vi "main.vi"() -> ()   [LabVIEW 2019]
uses:
  <vilib>/measure/mamon.llb/Trigger Detection for 1 Channel.vi
  <vilib>/addons/Fuzzy Logic/FL Fuzzy Controller (MISO).vi
  Setting Lib.lvlib
  detectedPellet.lvlib
  D02.lvlib
  D03.lvlib
  D04.lvlib
  D05.lvlib
  D01.lvlib
  database.lvlib
  <vilib>/measure/NI_MAPro.lvlib
  User Lib.lvlib
  <vilib>/addons/Fuzzy Logic/NI_Fuzzy_Logic_API.lvlib
  Maintenance.lvlib
  <vilib>/userDefined/High Color/IMAQdx.ctl
  <vilib>/Analysis/NI_AALPro.lvlib
  D06.lvlib
  <userlib>/DAQNavi Polymorphic VI/create/DAQNavi Create Channel(AI-Voltage).vi
  <userlib>/DAQNavi Polymorphic VI/create/DAQNavi Create Channel(DI-Digital Input).vi
  <userlib>/DAQNavi Polymorphic VI/read/DAQNavi Read (Digital 1D U8 NChan 1Samp).vi
  <userlib>/DAQNavi Polymorphic VI/read/DAQNavi Read (Analog 1D DBL NChan 1Samp).vi
  <userlib>/DAQNavi Polymorphic VI/create/DAQNavi Create Channel(DO-Digital Output).vi
  <userlib>/DAQNavi Polymorphic VI/write/DAQNavi Write (Digtial 1D U8 NChan 1Samp).vi
panel:
  out "Warning array 06":bool[](array[boolean])
  out "speed  min 06":bool
  out "speed max 06":bool
  out "10-14 6":dbl(slide) caption="10-14 mm" scale=0.0..100.0 scale format="%#.1f"
  out "8-16mm 6":dbl format="%.1g"
  out "AUTO/MAN 06":bool
  out "DISC 06":bool
  out "SPEED 07":dbl caption="SPEED" format="%#.2g"
  out "AVG 07":dbl caption="AVG" format="%#.2g"
  in  "Info 07":bool
  out "Warning 07":bool
  out "disc name 07":string="DISC 07"
  in  "Graph 07":bool
  in  "Live 07":bool
  out "AUTO/MAN 07":bool
  out "projector 07":bool
  out "cam 07":bool
  out "8-12.5 32":dbl(slide) caption="9-12.5 mm" scale=0.0..100.0 scale format="%#.1f"
  out "12.5-16 32":dbl(slide) caption="12.5-16 mm" scale=0.0..100.0 scale format="%#.1f"
  out "DISC 07":bool
  out "SPEED 06":dbl caption="SPEED" format="%#.2g"
  out "AVG 06":dbl caption="AVG" format="%#.2g"
  in  "Info 06":bool
  out "Warning 06":bool
  out "disc name 06":string="DISC 06"
  in  "Graph 06":bool
  in  "Live 06":bool
  out "projector 06":bool
  out "cam 06":bool
  out "8-12.5 06":dbl(slide) caption="9-12.5 mm" scale=0.0..100.0 scale format="%#.1f"
  out "12.5-16 06":dbl(slide) caption="12.5-16 mm" scale=0.0..100.0 scale format="%#.1f"
  out "rules as text out":string[](array[string])
  out "sudden change D05":bool
  out "pulse width D05":dbl
  out "slope D05":dbl
  out "previouse speed D05":dbl
  out "increase D05":bool
  out "decrease D05":bool
  out "sudden change D04":bool
  out "pulse width D04":dbl
  out "slope D04":dbl
  out "previouse speed D04":dbl
  out "increase D04":bool
  out "decrease D04":bool
  out "slope D03":dbl
  out "sudden change D03":bool
  out "pulse width D03":dbl
  out "previous speed D03":dbl
  out "increase D03":bool
  out "decrease D03":bool
  out "sudden change D02":bool
  out "pulse width D02":dbl
  out "slope D02":dbl
  out "previous speed D02":dbl
  out "increase D02":bool
  out "decrease D02":bool
  out "slope D01":dbl
  out "previous speed D01":dbl
  out "decrease D01":bool
  out "increase D01":bool
  out "last error 05":dbl
  out "no change D05":bool
  out "last error 04":dbl
  out "no change D04":bool
  out "last error 03":dbl
  out "no change D03":bool
  out "last error 02":dbl
  out "no change D02":bool
  out "sudden change D01":bool
  out "last error 01":dbl
  out "speed  min 05":bool
  out "speed max 05":bool
  out "speed  min 03":bool
  out "speed max 03":bool
  out "speed  min 04":bool
  out "speed max 04":bool
  out "speed  min 02":bool
  out "speed max 02":bool
  out "speed max 01":bool
  out "speed  min 01":bool
  out "no change D01":bool
  out "SPEED 05":dbl caption="SPEED" format="%#.2g"
  out "SPEED 04":dbl caption="SPEED" format="%#.2g"
  out "SPEED 03":dbl caption="SPEED" format="%#.2g"
  out "SPEED 02":dbl caption="SPEED" format="%#.2g"
  out "SPEED 01":dbl caption="SPEED" format="%#.2g"
  out "AVG 05":dbl caption="AVG" format="%#.2g"
  out "AVG 04":dbl caption="AVG" format="%#.2g"
  out "AVG 03":dbl caption="AVG" format="%#.2g"
  out "AVG 02":dbl caption="AVG" format="%#.2g"
  out "AVG 01":dbl caption="AVG" format="%#.2g"
  out "8-16mm total":dbl format="%.1g"
  out "8-16mm 05":dbl format="%.1g"
  out "8-16mm 04":dbl format="%.1g"
  out "8-16mm 03":dbl format="%.1g"
  out "8-16mm 27":dbl format="%.1g"
  out "8-16mm 26":dbl format="%.1g"
  out "10-14 total":dbl(slide) caption="10-14 mm" scale=0.0..100.0 scale format="%#.1f"
  out "10-14 05":dbl(slide) caption="10-14 mm" scale=0.0..100.0 scale format="%#.1f"
  out "10-14 04":dbl(slide) caption="10-14 mm" scale=0.0..100.0 scale format="%#.1f"
  out "10-14 03":dbl(slide) caption="10-14 mm" scale=0.0..100.0 scale format="%#.1f"
  out "10-14 02":dbl(slide) caption="10-14 mm" scale=0.0..100.0 scale format="%#.1f"
  out "10-14 01":dbl(slide) caption="10-14 mm" scale=0.0..100.0 scale format="%#.1f"
  out "error out 14":errorcluster
  out "error out 13":errorcluster
  out "error out 12":errorcluster
  in  "Info 05":bool
  in  "Info 04":bool
  in  "Info 03":bool
  in  "Info 02":bool
  in  "Info 01":bool
  out "error out":errorcluster
  out "avg grading array size":i32=4000
  out "live grading array size":i32=2000
  out "error out 8":errorcluster
  out "error out 7":errorcluster
  out "error out 6":errorcluster
  out "Elapsed Time (s) 6":dbl caption="Elapsed Time (s)"
  out "output value 5":dbl
  out "Elapsed Time (s) 5":dbl caption="Elapsed Time (s)"
  out "output value 4":dbl
  out "Elapsed Time (s) 4":dbl caption="Elapsed Time (s)"
  out "output value 3":dbl
  out "error out 5":errorcluster
  out "Elapsed Time (s) 3":dbl caption="Elapsed Time (s)"
  out "output value 2":dbl
  out "error out 3":errorcluster
  out "puls width D01":dbl
  out "Elapsed Time (s) 2":dbl caption="Elapsed Time (s)"
  out "2D array out":dbl[][](array[numeric])
  out "Warning array 01":bool[](array[boolean])
  out "Warning array 02":bool[](array[boolean])
  out "Warning array 03":bool[](array[boolean])
  out "Warning array 04":bool[](array[boolean])
  out "Warning array 05":bool[](array[boolean])
  out "Warning 05":bool
  in  "speed disc 30":i32
  in  "speed disc 29":i32
  in  "Error in 18":errorcluster
  in  "speed disc 28":i32
  in  "speed disc 27":i32
  in  "speed disc 26":i32
  out "Warning 04":bool
  out "Warning 03":bool
  out "Warning 02":bool
  out "Warning 01":bool
  out "overal result":string="Overal Result"
  out "disc name 05":string="DISC 05"
  out "disc name 04":string="DISC 04"
  out "disc name 03":string="DISC 03"
  out "disc name 02":string="DISC 02"
  in  "Setting":bool
  out "disc name 01":string="DISC 01"
  in  "Graph 05":bool
  in  "Live 05":bool
  in  "Graph 04":bool
  in  "Live 04":bool
  in  "Graph 03":bool
  in  "Live 03":bool
  in  "Graph 02":bool
  in  "Live 02":bool
  out "Software name":string="DORSA Smart Grading System (DSGS)"
  out "time&date":string="2020/11/22"
  in  "Maintenance":bool
  in  "Shutdown":bool
  in  "Restart":bool
  in  "Close":bool
  in  "View":bool
  in  "Report":bool
  in  "Login":bool=TRUE
  in  "Graph 01":bool
  in  "Live 01":bool
  out "8-12.5 02":dbl(slide) caption="9-12.5 mm" scale=0.0..100.0 scale format="%#.1f"
  out "12.5-16 02":dbl(slide) caption="12.5-16 mm" scale=0.0..100.0 scale format="%#.1f"
  out "AUTO/MAN 05":bool
  out "projector 05":bool
  out "cam 05":bool
  out "8-12.5 05":dbl(slide) caption="9-12.5 mm" scale=0.0..100.0 scale format="%#.1f"
  out "12.5-16 05":dbl(slide) caption="12.5-16 mm" scale=0.0..100.0 scale format="%#.1f"
  out "DISC 05":bool
  out "AUTO/MAN 04":bool
  out "projector 04":bool
  out "cam 04":bool
  out "8-12.5 04":dbl(slide) caption="9-12.5 mm" scale=0.0..100.0 scale format="%#.1f"
  out "12.5-16 04":dbl(slide) caption="12.5-16 mm" scale=0.0..100.0 scale format="%#.1f"
  out "DISC 04":bool
  out "AUTO/MAN 03":bool
  out "projector 03":bool
  out "cam 03":bool
  out "8-12.5 03":dbl(slide) caption="9-12.5 mm" scale=0.0..100.0 scale format="%#.1f"
  out "12.5-16 03":dbl(slide) caption="12.5-16 mm" scale=0.0..100.0 scale format="%#.1f"
  out "DISC 03":bool
  out "AUTO/MAN 02":bool
  out "projector 02":bool
  out "cam 02":bool
  out "DISC 02":bool
  out "AUTO/MAN 01":bool
  out "projector 01":bool
  out "cam 01":bool
  out "8-12.5 01":dbl(slide) caption="8-12.5 mm" scale=0.0..100.0 scale format="%#.1f"
  out "12.5-16 01":dbl(slide) caption="12.5-16 mm" scale=0.0..100.0 scale format="%#.1f"
  out "DISC 01":bool
  out "12.5-16 total":dbl(slide) caption="12.5-16 mm" scale=0.0..100.0 scale format="%#.1f"
  out "8-12.5 total":dbl(slide) caption="9-12.5mm" scale=0.0..100.0 scale format="%#.1f"
  out "Over Size":dbl format="%#.2g"
  out "AVG":dbl format="%#.2g"
  out "Under Size":dbl format="%#.2g"
types:
  T1 = cluster{"disc 06":bool, "auto/man 06":bool, "projector 06":bool, "cam 06":bool}
  T2 = cluster{"disc 05":bool, "auto/man 05":bool, "projector 05":bool, "cam 05":bool}
  T3 = cluster{"disc 04":bool, "auto/man 04":bool, "projector 04":bool, "cam 04":bool}
  T4 = cluster{"disc 03":bool, "auto/man 03":bool, "projector 03":bool, "cam 03":bool}
  T5 = cluster{"disc 02":bool, "auto/man 02":bool, "projector 02":bool, "cam 02":bool}
  T6 = cluster{"disc 01":bool, "auto/man 01":bool, "projector 01":bool, "cam 01":bool}
  T7 = typedef "IMAQ Image.ctl" = refnum<image>
  T8 = enum32{"Invalid", "Standard", "Closed", "Hidden", "Minimized", "Maximized"}
  T9 = typedef "IMAQdx.ctl" = refnum<k21>
  T10 = enum8{"Enabled", "Disabled", "Disabled and Grayed Out"}
  T11 = cluster{string, "date/time string":string, "date/time string":string, string}
  T12 = cluster{i32, "date/time string":string, "date/time string":string, string}
  T13 = cluster{"disc 01":bool, "auto/man 01":bool, "projector 01":bool, "cam 01":bool}[]
  T14 = cluster{"disc 02":bool, "auto/man 02":bool, "projector 02":bool, "cam 02":bool}[]
  T15 = cluster{"disc 06":bool, "auto/man 06":bool, "projector 06":bool, "cam 06":bool}[]
  T16 = cluster{"disc 05":bool, "auto/man 05":bool, "projector 05":bool, "cam 05":bool}[]
  T17 = cluster{"disc 03":bool, "auto/man 03":bool, "projector 03":bool, "cam 03":bool}[]
  T18 = cluster{"disc 04":bool, "auto/man 04":bool, "projector 04":bool, "cam 04":bool}[]
  T19 = typedef "LVDateTimeRec.ctl" = cluster{"fractional second":dbl, "second":i32, "minute":i32, "hour":i32, "day of month":i32, "month":i32, "year":i32, "day of week":i32, "day of year":i32, "DST":i32}
  T20 = cluster{"date/time string":string, "date/time string":string, dbl, dbl, dbl, dbl, dbl, dbl, dbl, dbl, "f":string, "f":string, "time format string (%c)":string, "time format string (%c)":string}
  T21 = cluster{"date/time string":string, "date/time string":string, dbl, dbl, "f":string, "f":string, "time format string (%c)":string, "time format string (%c)":string}
  T22 = cluster{"date/time string":string, "date/time string":string, string, "spreadsheet string":string}
  T23 = typedef "NI_Fuzzy_Logic_API.lvlib/FL System.ctl" = cluster{"input variables":T24[], "output variables":T24[], "rules":T27[], "defuzzification method":T33, "description":string, "user MF interpolating polynomials":T34[]}
  T24 = typedef "NI_Fuzzy_Logic_API.lvlib/FL Variable.ctl" = cluster{"name":string, "range":dbl[], "MFs":T25[]}
  T25 = typedef "NI_Fuzzy_Logic_API.lvlib/FL Membership Function.ctl" = cluster{"name":string, "shape":T26, "points":dbl[], "color":u32, "user-defined shape index":i32}
  T26 = typedef "NI_Fuzzy_Logic_API.lvlib/FL Membership Function Shape.ctl" = u16
  T27 = typedef "NI_Fuzzy_Logic_API.lvlib/FL Rule.ctl" = cluster{"antecedents":T28[], "antecedent connective":T30, "consequents":T31[], "consequent implication":T32, "degree of support":dbl}
  T28 = typedef "NI_Fuzzy_Logic_API.lvlib/FL Antecedent.ctl" = cluster{"Var Index":i32, "MF Index":i32, "Cond":T29}
  T29 = typedef "NI_Fuzzy_Logic_API.lvlib/FL Modifier.ctl" = u16
  T30 = typedef "NI_Fuzzy_Logic_API.lvlib/FL Antecedent Connective.ctl" = u16
  T31 = typedef "NI_Fuzzy_Logic_API.lvlib/FL Consequent.ctl" = cluster{"Var Index":i32, "MF Index":i32, "Cond":T29}
  T32 = typedef "NI_Fuzzy_Logic_API.lvlib/FL Consequent Implication.ctl" = u16
  T33 = typedef "NI_Fuzzy_Logic_API.lvlib/FL Defuzzification.ctl" = u16
  T34 = typedef "NI_Fuzzy_Logic_API.lvlib/FL Interpolating polynomials.ctl" = cluster{"X":dbl[], "Y":dbl[], "Y(x) coeff":dbl[][], "X(y) coeff":dbl[][], "Area(y) coeff":dbl[][], "coa_x(y) coeff":dbl[][]}
  T35 = cluster{"decrease D01":bool, "increase D01":bool, "no change D01":bool, "sudden change D01":bool, "last error 01":dbl, "previous speed D01":dbl, "puls width D01":dbl, "slope D01":dbl}
  T36 = cluster{"decrease D05":bool, "increase D05":bool, "no change D05":bool, "sudden change D05":bool, "last error 05":dbl, "previouse speed D05":dbl, "pulse width D05":dbl, "slope D05":dbl}
  T37 = cluster{"decrease D02":bool, "increase D02":bool, "no change D02":bool, "sudden change D02":bool, "last error 02":dbl, "previous speed D02":dbl, "pulse width D02":dbl, "slope D02":dbl}
  T38 = cluster{"decrease D04":bool, "increase D04":bool, "no change D04":bool, "sudden change D04":bool, "last error 04":dbl, "previouse speed D04":dbl, "pulse width D04":dbl, "slope D04":dbl}
  T39 = cluster{"decrease D03":bool, "increase D03":bool, "no change D03":bool, "sudden change D03":bool, "last error 03":dbl, "previous speed D03":dbl, "pulse width D03":dbl, "slope D03":dbl}
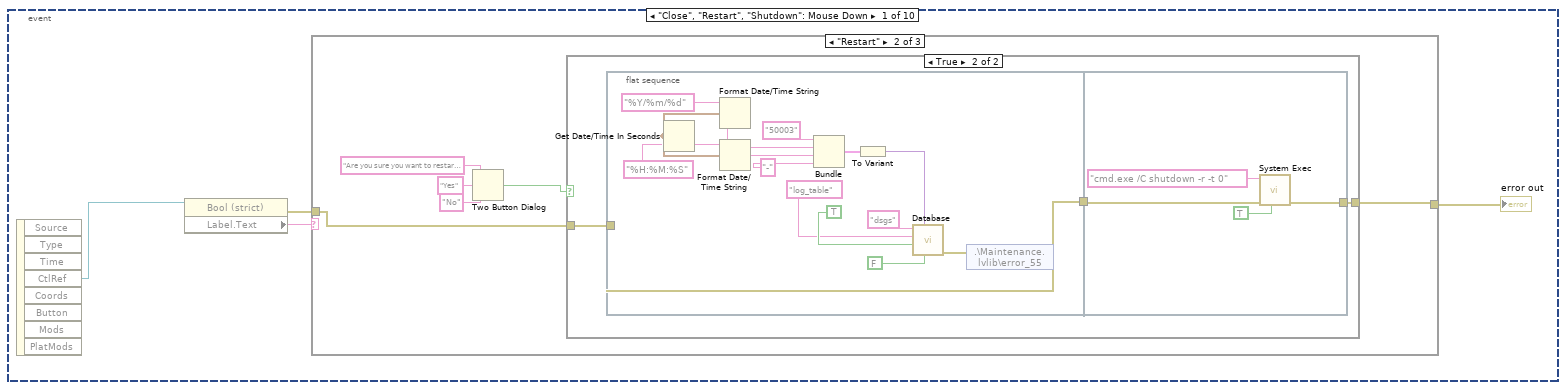
[diagram p3: hidden frame]
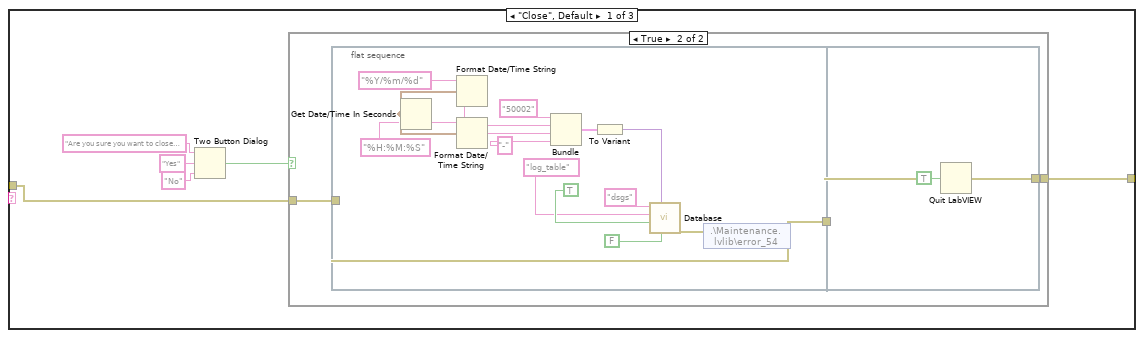
[diagram p4: hidden frame]
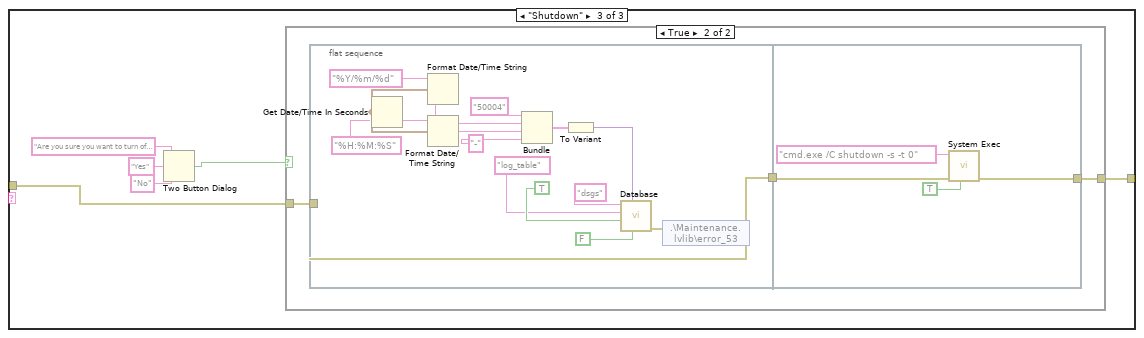
[diagram p7: hidden frame]
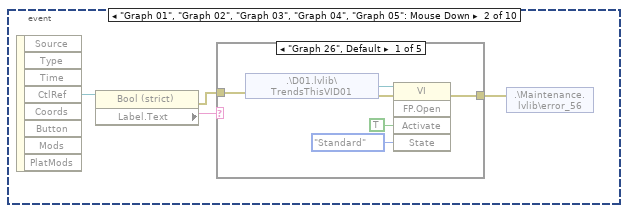
[diagram p9: hidden frame]
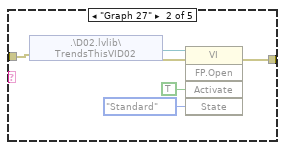
[diagram p10: hidden frame]
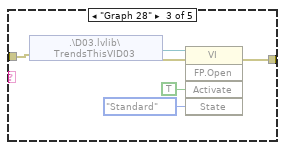
[diagram p11: hidden frame]
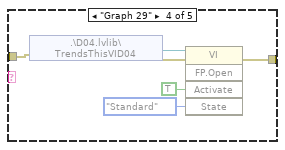
[diagram p12: hidden frame]
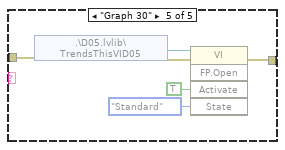
[diagram p13: hidden frame]
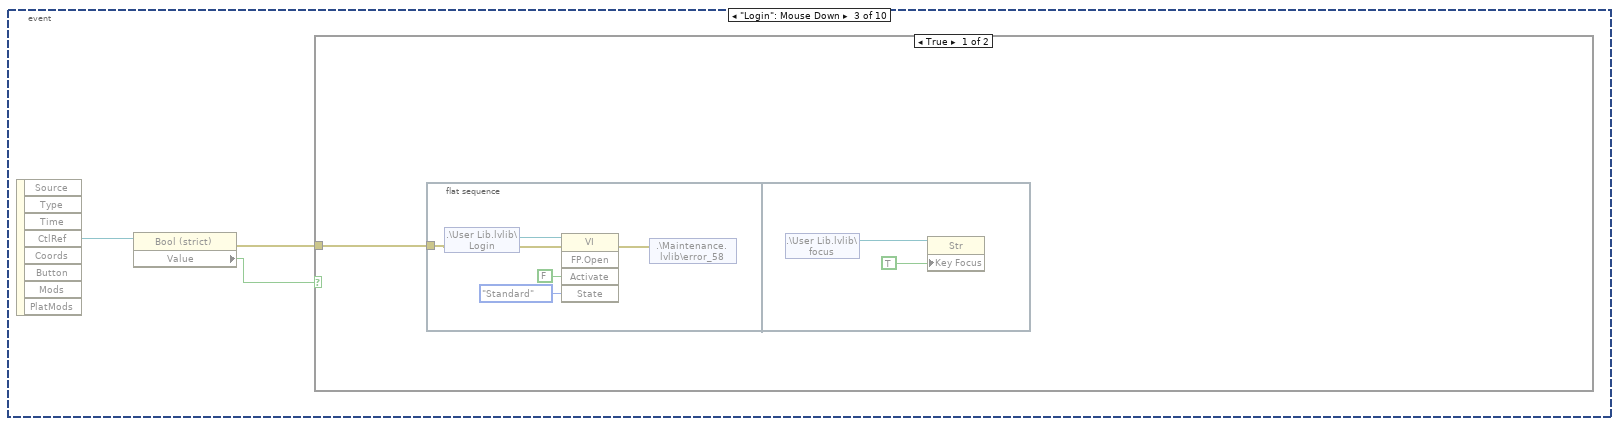
[diagram p14: hidden frame]
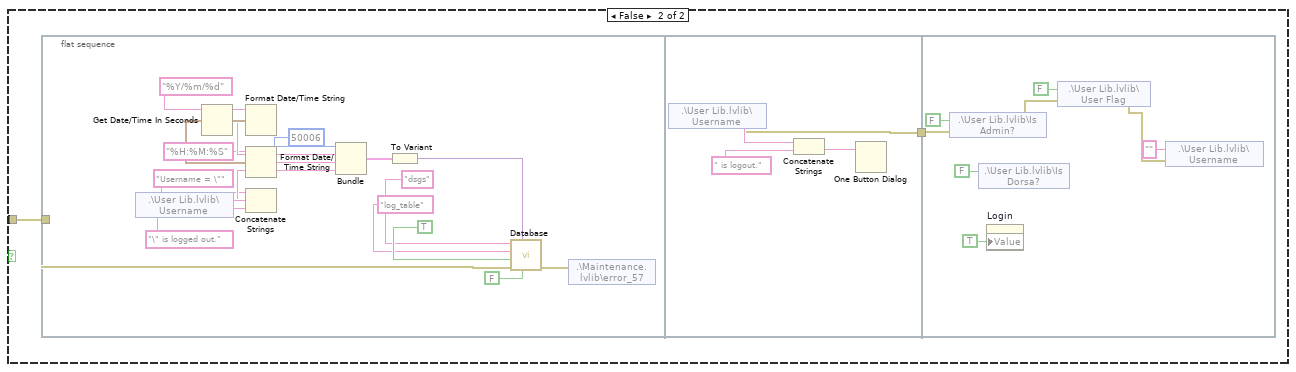
[diagram p15: hidden frame]
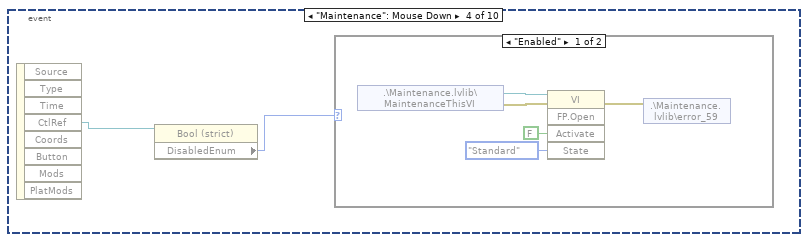
[diagram p16: hidden frame]
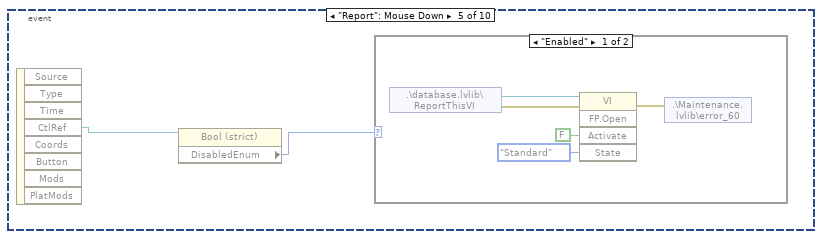
[diagram p18: hidden frame]
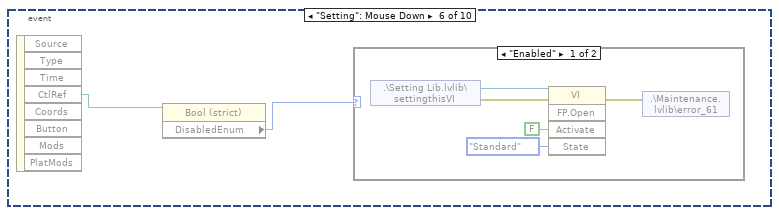
[diagram p20: hidden frame]
diagram:
  w80 = 4000 ("dimension size")
  w85 = 1000 ("dimension size")
  n1 = call "IMAQ Create"("Image Name"="img in D01") -> ("New Image"=w53:T7, "error out"=w44:errorcluster)  [unwired: 4 in]
  n2 = shared-variable ".\\Maintenance.lvlib\\error_2"(w44) -> ()  [unwired: 1 in, 1 out]
  n3 = call "IMAQ Create"("Image Name"="img in D02") -> ("New Image"=w27:T7, "error out"=w43:errorcluster)  [unwired: 4 in]
  n4 = shared-variable ".\\Maintenance.lvlib\\error_3"(w43) -> ()  [unwired: 1 in, 1 out]
  n5 = call "IMAQ Create"("Image Name"="img in D03") -> ("New Image"=w48:T7, "error out"=w42:errorcluster)  [unwired: 4 in]
  n6 = shared-variable ".\\Maintenance.lvlib\\error_4"(w42) -> ()  [unwired: 1 in, 1 out]
  n7 = call "IMAQ Create"("Image Name"="img in D04") -> ("New Image"=w47:T7, "error out"=w41:errorcluster)  [unwired: 4 in]
  n8 = shared-variable ".\\Maintenance.lvlib\\error_5"(w41) -> ()  [unwired: 1 in, 1 out]
  n9 = call "IMAQ Create"("Image Name"="img in D05") -> ("New Image"=w46:T7, "error out"=w40:errorcluster)  [unwired: 4 in]
  n10 = call "IMAQ Create"("Image Name"="img out D01") -> ("New Image"=w96:T7, "error out"=w39:errorcluster)  [unwired: 4 in]
  n11 = shared-variable ".\\Maintenance.lvlib\\error_6"(w40) -> ()  [unwired: 1 in, 1 out]
  n12 = shared-variable ".\\Maintenance.lvlib\\error_7"(w39) -> ()  [unwired: 1 in, 1 out]
  n13 = call "IMAQ Create"("Image Name"="img out D02") -> ("New Image"=w94:T7, "error out"=w38:errorcluster)  [unwired: 4 in]
  n14 = call "IMAQ Create"("Image Name"="img in D06") -> ("New Image"=w6:T7)  [unwired: 4 in, 1 out]
  n15 = shared-variable ".\\Maintenance.lvlib\\error_8"(w38) -> ()  [unwired: 1 in, 1 out]
  n16 = call "IMAQ Create"("Image Name"="img out D03") -> ("New Image"=w92:T7, "error out"=w37:errorcluster)  [unwired: 4 in]
  n17 = shared-variable ".\\Maintenance.lvlib\\error_9"(w37) -> ()  [unwired: 1 in, 1 out]
  n18 = call "IMAQ Create"("Image Name"="img out D04") -> ("New Image"=w89:T7, "error out"=w36:errorcluster)  [unwired: 4 in]
  n19 = shared-variable ".\\Maintenance.lvlib\\error_10"(w36) -> ()  [unwired: 1 in, 1 out]
  n20 = disable-structure shown="Disabled" {
    frame Disabled {
      n21 = call-poly <userlib>:"DAQNavi Create Channel.vi"("physical channels"="PCI-1710,BID#0/ai0:9", "signal type"="Differential", "value range"="0 ~ 10 V") -> ("task out"=w112:i32, "error out"=w111:errorcluster)  [unwired: 11 in]
      n22 = call-poly <userlib>:"DAQNavi Create Channel.vi"("physical channels"="PCI-1710,BID#0/port0:1") -> ("task out"=w110:i32, "error out"=w109:errorcluster)  [unwired: 13 in]
      n23 = while {
        tunnel: w112 -> [w123]
        tunnel: w111 -> [w122]
        tunnel: w110 -> [w121]
        tunnel: w109 -> [w120]
        stop <- FALSE stop-if-true
        n24 = event shown="[9] Timeout" {
          selector: _ -> [_ _ _ _ _ _ _ _ _ _]
          dyn-events: _ -> [_ _ _ _ _ _ _ _ _ _]
          timeout: 0 -> [_ _ _ _ _ _ _ _ _ _]
          tunnel: w123 -> [_ _ _ _ _ _ _ _ _ w610]
          tunnel: w122 -> [_ _ _ _ _ _ _ _ _ w609]
          tunnel: w121 -> [_ _ _ _ _ _ _ _ _ w595]
          tunnel: w120 -> [_ _ _ _ _ _ _ _ _ w594]
          event "Close", "Restart", "Shutdown": Mouse Down {
            n25 = event-data() -> ("CtlRef"=w129:refnum<vi>)  [unwired: 1 in, 7 out]
            n26 = property class="Bool (strict)"(reference=w129) -> (error out=w128:errorcluster, "Label.Text"=w130:string)  [unwired: 1 in, 1 out]
            n27 = case shown="\"Restart\"" w130 {
              tunnel: [w131 w158 w188] -> w127
              tunnel: w128 -> [w132 w159 w187]
              frame "Close", Default {
                n28 = Two Button Dialog(message="Are you sure you want to close the application?", 1:"No" ("F button name (\"Cancel\")"), 2:"Yes" ("T button name (\"OK\")")) -> (T button?=w133:bool)
                n29 = case shown="True" w133 {
                  tunnel: w132 -> [w137 w138]
                  tunnel: [w137 w140] -> w131
                  frame False {
                  }
                  frame True {
                    n30 = flat-sequence {
                      tunnel: [w141] -> w139
                      tunnel: w138 -> [w141]
                      tunnel: [w156] -> w140
                      tunnel: w139 -> [w156]
                      frame #0 {
                        n31 = Get Date/Time In Seconds() -> (seconds since 1Jan1904=w151:timestamp)
                        n32 = Format Date/Time String(time format string (%c)="%Y/%m/%d", seconds (now)=w151) -> (date/time string=w152:string)  [unwired: 1 in]
                        n33 = Format Date/Time String(time format string (%c)="%H:%M:%S", seconds (now)=w151) -> (date/time string=w153:string)  [unwired: 1 in]
                        n34 = Bundle("50002", "date/time string"=w152, "date/time string"=w153, "-") -> (w154:T11)  [unwired: 1 in]
                        n35 = To Variant(anything=w154) -> (Variant=w155:variant)
                        n36 = call "Database.vi"("Delete row?"=FALSE, "Data"=w155, "Auto Increment ID?"=TRUE, "Table"="log_table", "Connection"="dsgs") -> ("Error out"=w142:errorcluster)  [unwired: 6 in]
                        n37 = shared-variable ".\\Maintenance.lvlib\\error_54"(w142) -> ()  [unwired: 1 in, 1 out]
                      }
                      frame #1 {
                        n38 = Quit LabVIEW(quit? (T)=TRUE) -> ()
                      }
                    }
                  }
                }
              }
              frame "Restart" {
                n39 = Two Button Dialog(message="Are you sure you want to restart the system?", 1:"No" ("F button name (\"Cancel\")"), 2:"Yes" ("T button name (\"OK\")")) -> (T button?=w160:bool)
                n40 = case shown="True" w160 {
                  tunnel: w159 -> [w164 w167]
                  tunnel: [w164 w165] -> w158
                  frame False {
                  }
                  frame True {
                    n41 = flat-sequence {
                      tunnel: w167 -> [w169]
                      tunnel: [w169] -> w166
                      tunnel: w166 -> [w184]
                      tunnel: [w183] -> w165
                      frame #0 {
                        n42 = Get Date/Time In Seconds() -> (seconds since 1Jan1904=w178:timestamp)
                        n43 = Format Date/Time String(time format string (%c)="%Y/%m/%d", seconds (now)=w178) -> (date/time string=w179:string)  [unwired: 1 in]
                        n44 = Format Date/Time String(time format string (%c)="%H:%M:%S", seconds (now)=w178) -> (date/time string=w180:string)  [unwired: 1 in]
                        n45 = Bundle("50003", "date/time string"=w179, "date/time string"=w180, "-") -> (w181:T11)  [unwired: 1 in]
                        n46 = To Variant(anything=w181) -> (Variant=w182:variant)
                        n47 = call "Database.vi"("Delete row?"=FALSE, "Data"=w182, "Auto Increment ID?"=TRUE, "Table"="log_table", "Connection"="dsgs") -> ("Error out"=w168:errorcluster)  [unwired: 6 in]
                        n48 = shared-variable ".\\Maintenance.lvlib\\error_55"(w168) -> ()  [unwired: 1 in, 1 out]
                      }
                      frame #1 {
                        n49 = call <vilib>:"System Exec.vi"("run minimized? (F)"=TRUE, "error in (no error)"=w184, "command line"="cmd.exe /C shutdown -r -t 0") -> ("error out"=w183:errorcluster)  [unwired: 5 in, 3 out]
                      }
                    }
                  }
                }
              }
              frame "Shutdown" {
                n50 = Two Button Dialog(message="Are you sure you want to turn off the system?", 1:"No" ("F button name (\"Cancel\")"), 2:"Yes" ("T button name (\"OK\")")) -> (T button?=w189:bool)
                n51 = case shown="True" w189 {
                  tunnel: [w193 w196] -> w188
                  tunnel: w187 -> [w193 w195]
                  frame False {
                  }
                  frame True {
                    n52 = flat-sequence {
                      tunnel: w195 -> [w197]
                      tunnel: [w197] -> w194
                      tunnel: [w213] -> w196
                      tunnel: w194 -> [w212]
                      frame #0 {
                        n53 = Get Date/Time In Seconds() -> (seconds since 1Jan1904=w207:timestamp)
                        n54 = Format Date/Time String(time format string (%c)="%Y/%m/%d", seconds (now)=w207) -> (date/time string=w208:string)  [unwired: 1 in]
                        n55 = Format Date/Time String(time format string (%c)="%H:%M:%S", seconds (now)=w207) -> (date/time string=w209:string)  [unwired: 1 in]
                        n56 = Bundle("50004", "date/time string"=w208, "date/time string"=w209, "-") -> (w210:T11)  [unwired: 1 in]
                        n57 = To Variant(anything=w210) -> (Variant=w211:variant)
                        n58 = call "Database.vi"("Delete row?"=FALSE, "Data"=w211, "Auto Increment ID?"=TRUE, "Table"="log_table", "Connection"="dsgs") -> ("Error out"=w198:errorcluster)  [unwired: 6 in]
                        n59 = shared-variable ".\\Maintenance.lvlib\\error_53"(w198) -> ()  [unwired: 1 in, 1 out]
                      }
                      frame #1 {
                        n60 = call <vilib>:"System Exec.vi"("run minimized? (F)"=TRUE, "error in (no error)"=w212, "command line"="cmd.exe /C shutdown -s -t 0") -> ("error out"=w213:errorcluster)  [unwired: 5 in, 3 out]
                      }
                    }
                  }
                }
              }
            }
            "error out" <- w127
          }
          event "Graph 01", "Graph 02", "Graph 03", "Graph 04", "Graph 05": Mouse Down {
            n61 = event-data() -> ("CtlRef"=w217:refnum<vi>)  [unwired: 1 in, 7 out]
            n62 = property class="Bool (strict)"(reference=w217) -> (error out=w218:errorcluster, "Label.Text"=w219:string)  [unwired: 1 in, 1 out]
            n63 = case shown="\"Graph 26\", Default" w219 {
              tunnel: w218 -> [w222 w227 w233 w239 w245]
              tunnel: [w220 w226 w232 w238 w244] -> w216
              frame "Graph 26", Default {
                n64 = shared-variable ".\\D01.lvlib\\TrendsThisVID01"(error in=w222) -> (w225:refnum<vi>, error out=w221:errorcluster)
                n65 = invoke class="VI" method="FP.Open"(reference=w225, error in=w221, "Activate"=TRUE ("Activate?"), "State"=T8."Standard") -> (error out=w220:errorcluster)  [unwired: 1 in, 4 out]
              }
              frame "Graph 27" {
                n66 = shared-variable ".\\D02.lvlib\\TrendsThisVID02"(error in=w227) -> (w230:refnum<vi>, error out=w231:errorcluster)
                n67 = invoke class="VI" method="FP.Open"(reference=w230, error in=w231, "Activate"=TRUE ("Activate?"), "State"=T8."Standard") -> (error out=w226:errorcluster)  [unwired: 1 in, 4 out]
              }
              frame "Graph 28" {
                n68 = shared-variable ".\\D03.lvlib\\TrendsThisVID03"(error in=w233) -> (w236:refnum<vi>, error out=w237:errorcluster)
                n69 = invoke class="VI" method="FP.Open"(reference=w236, error in=w237, "Activate"=TRUE ("Activate?"), "State"=T8."Standard") -> (error out=w232:errorcluster)  [unwired: 1 in, 4 out]
              }
              frame "Graph 29" {
                n70 = shared-variable ".\\D04.lvlib\\TrendsThisVID04"(error in=w239) -> (w242:refnum<vi>, error out=w243:errorcluster)
                n71 = invoke class="VI" method="FP.Open"(reference=w242, error in=w243, "Activate"=TRUE ("Activate?"), "State"=T8."Standard") -> (error out=w238:errorcluster)  [unwired: 1 in, 4 out]
              }
              frame "Graph 30" {
                n72 = shared-variable ".\\D05.lvlib\\TrendsThisVID05"(error in=w245) -> (w248:refnum<vi>, error out=w249:errorcluster)
                n73 = invoke class="VI" method="FP.Open"(reference=w248, error in=w249, "Activate"=TRUE ("Activate?"), "State"=T8."Standard") -> (error out=w244:errorcluster)  [unwired: 1 in, 4 out]
              }
            }
            n74 = shared-variable ".\\Maintenance.lvlib\\error_56"(w216) -> ()  [unwired: 1 in, 1 out]
          }
          event "Login": Mouse Down {
            n75 = event-data() -> ("CtlRef"=w252:refnum<vi>)  [unwired: 1 in, 7 out]
            n76 = property class="Bool (strict)"(reference=w252) -> (error out=w250:errorcluster, "Value"=w251:bool)  [unwired: 1 in, 1 out]
            n77 = case shown="True" w251 {
              tunnel: w250 -> [w253 w262]
              frame True {
                n78 = flat-sequence {
                  tunnel: w253 -> [w258]
                  frame #0 {
                    n79 = shared-variable ".\\User Lib.lvlib\\Login"() -> (w257:refnum<vi>)  [unwired: 1 in, 1 out]
                    n80 = invoke class="VI" method="FP.Open"(reference=w257, error in=w258, "Activate"=FALSE ("Activate?"), "State"=T8."Standard") -> (error out=w254:errorcluster)  [unwired: 1 in, 4 out]
                    n81 = shared-variable ".\\Maintenance.lvlib\\error_58"(w254) -> ()  [unwired: 1 in, 1 out]
                  }
                  frame #1 {
                    n82 = shared-variable ".\\User Lib.lvlib\\focus"() -> (w260:refnum<vi>)  [unwired: 1 in, 1 out]
                    n83 = property class="Str"(reference=w260, "Key Focus"=TRUE) -> ()  [unwired: 1 in, 2 out]
                  }
                }
              }
              frame False {
                n84 = flat-sequence {
                  tunnel: w262 -> [w264]
                  tunnel: [w281] -> w261
                  tunnel: w261 -> [w288]
                  frame #0 {
                    n85 = shared-variable ".\\User Lib.lvlib\\Username"() -> (w280:string)  [unwired: 1 in, 1 out]
                    n86 = Get Date/Time In Seconds() -> (seconds since 1Jan1904=w278:timestamp)
                    n87 = Format Date/Time String(time format string (%c)="%Y/%m/%d", seconds (now)=w278) -> (date/time string=w277:string)  [unwired: 1 in]
                    n88 = Format Date/Time String(time format string (%c)="%H:%M:%S", seconds (now)=w278) -> (date/time string=w276:string)  [unwired: 1 in]
                    n89 = Concatenate Strings("Username = \"" ("string"), w280, "\" is logged out." ("string")) -> (w279:string)
                    n90 = Bundle(50006, "date/time string"=w277, "date/time string"=w276, w279) -> (w275:T12)  [unwired: 1 in]
                    n91 = To Variant(anything=w275) -> (Variant=w274:variant)
                    n92 = call "Database.vi"("Delete row?"=FALSE, "Data"=w274, "Error in"=w264, "Auto Increment ID?"=TRUE, "Table"="log_table" ("table"), "Connection"="dsgs" ("table")) -> ("Error out"=w263:errorcluster)  [unwired: 5 in]
                    n93 = shared-variable ".\\Maintenance.lvlib\\error_57"(w263) -> ()  [unwired: 1 in, 1 out]
                  }
                  frame #1 {
                    n94 = shared-variable ".\\User Lib.lvlib\\Username"() -> (w283:string, error out=w281:errorcluster)  [unwired: 1 in]
                    n95 = Concatenate Strings(w283, " is logout." ("string")) -> (w284:string)
                    n96 = One Button Dialog(message=w284) -> ()  [unwired: 1 in, 1 out]
                  }
                  frame #2 {
                    n97 = shared-variable ".\\User Lib.lvlib\\Is Admin?"(FALSE ("Is Admin?"), error in=w288) -> (error out=w287:errorcluster)
                    n98 = shared-variable ".\\User Lib.lvlib\\Is Dorsa?"(FALSE ("Is Admin?")) -> ()  [unwired: 1 in, 1 out]
                    n99 = property on="Login" class="Bool (strict)"("Value"=TRUE ("Login")) -> ()  [unwired: 2 in, 2 out]
                    n100 = shared-variable ".\\User Lib.lvlib\\User Flag"(FALSE ("User Flag"), error in=w287) -> (error out=w286:errorcluster)
                    n101 = shared-variable ".\\User Lib.lvlib\\Username"("" ("Username"), error in=w286) -> ()  [unwired: 1 out]
                  }
                }
              }
            }
          }
          event "Maintenance": Mouse Down {
            n102 = event-data() -> ("CtlRef"=w294:refnum<vi>)  [unwired: 1 in, 7 out]
            n103 = property class="Bool (strict)"(reference=w294) -> ("DisabledEnum"=w293:T10)  [unwired: 1 in, 2 out]
            n104 = case shown="\"Enabled\"" w293 {
              frame "Enabled" {
                n105 = shared-variable ".\\Maintenance.lvlib\\MaintenanceThisVI"() -> (w299:refnum<vi>, error out=w298:errorcluster)  [unwired: 1 in]
                n106 = invoke class="VI" method="FP.Open"(reference=w299, error in=w298, "Activate"=FALSE ("Activate?"), "State"=T8."Standard") -> (error out=w297:errorcluster)  [unwired: 1 in, 4 out]
                n107 = shared-variable ".\\Maintenance.lvlib\\error_59"(w297) -> ()  [unwired: 1 in, 1 out]
              }
              frame "Disabled", Default {
              }
            }
          }
          event "Report": Mouse Down {
            n108 = event-data() -> ("CtlRef"=w301:refnum<vi>)  [unwired: 1 in, 7 out]
            n109 = property class="Bool (strict)"(reference=w301) -> ("DisabledEnum"=w300:T10)  [unwired: 1 in, 2 out]
            n110 = case shown="\"Enabled\"" w300 {
              frame "Enabled" {
                n111 = shared-variable ".\\database.lvlib\\ReportThisVI"() -> (w304:refnum<vi>, error out=w306:errorcluster)  [unwired: 1 in]
                n112 = invoke class="VI" method="FP.Open"(reference=w304, error in=w306, "Activate"=FALSE ("Activate?"), "State"=T8."Standard") -> (error out=w305:errorcluster)  [unwired: 1 in, 4 out]
                n113 = shared-variable ".\\Maintenance.lvlib\\error_60"(w305) -> ()  [unwired: 1 in, 1 out]
              }
              frame "Disabled", Default {
              }
            }
          }
          event "Setting": Mouse Down {
            n114 = event-data() -> ("CtlRef"=w308:refnum<vi>)  [unwired: 1 in, 7 out]
            n115 = property class="Bool (strict)"(reference=w308) -> ("DisabledEnum"=w307:T10)  [unwired: 1 in, 2 out]
            n116 = case shown="\"Enabled\"" w307 {
              frame "Enabled" {
                n117 = shared-variable ".\\Setting Lib.lvlib\\settingthisVI"() -> (w312:refnum<vi>, error out=w311:errorcluster)  [unwired: 1 in]
                n118 = invoke class="VI" method="FP.Open"(reference=w312, error in=w311, "Activate"=FALSE ("Activate?"), "State"=T8."Standard") -> (error out=w313:errorcluster)  [unwired: 1 in, 4 out]
                n119 = shared-variable ".\\Maintenance.lvlib\\error_61"(w313) -> ()  [unwired: 1 in, 1 out]
              }
              frame "Disabled", Default {
              }
            }
          }
          event "View", "Live 01", "Live 02", "Live 03", "Live 04", "Live 05": Mouse Down {
            n120 = event-data() -> ("CtlRef"=w315:refnum<vi>)  [unwired: 1 in, 7 out]
            n121 = property class="Bool (strict)"(reference=w315) -> (error out=w316:errorcluster, "Label.Text"=w317:string)  [unwired: 1 in, 1 out]
            n122 = case shown="\"View\"" w317 {
              tunnel: w316 -> [w320 w329 w331 w337 w343 w350]
              tunnel: [w318 w324 w330 w336 w342 w351] -> w314
              frame "Live 26", Default {
                n123 = shared-variable ".\\D01.lvlib\\D01thisVI"(error in=w320) -> (w323:refnum<vi>, error out=w319:errorcluster)
                n124 = invoke class="VI" method="FP.Open"(reference=w323, error in=w319, "Activate"=FALSE ("Activate?"), "State"=T8."Standard") -> (error out=w318:errorcluster)  [unwired: 1 in, 4 out]
              }
              frame "Live 27" {
                n125 = shared-variable ".\\D02.lvlib\\D02thisVI"(error in=w329) -> (w328:refnum<vi>, error out=w327:errorcluster)
                n126 = invoke class="VI" method="FP.Open"(reference=w328, error in=w327, "Activate"=TRUE ("Activate?"), "State"=T8."Standard") -> (error out=w324:errorcluster)  [unwired: 1 in, 4 out]
              }
              frame "Live 28" {
                n127 = shared-variable ".\\D03.lvlib\\D03thisVI"(error in=w331) -> (w333:refnum<vi>, error out=w332:errorcluster)
                n128 = invoke class="VI" method="FP.Open"(reference=w333, error in=w332, "Activate"=TRUE ("Activate?"), "State"=T8."Standard") -> (error out=w330:errorcluster)  [unwired: 1 in, 4 out]
              }
              frame "Live 29" {
                n129 = shared-variable ".\\D04.lvlib\\D04thisVI"(error in=w337) -> (w339:refnum<vi>, error out=w338:errorcluster)
                n130 = invoke class="VI" method="FP.Open"(reference=w339, error in=w338, "Activate"=TRUE ("Activate?"), "State"=T8."Standard") -> (error out=w336:errorcluster)  [unwired: 1 in, 4 out]
              }
              frame "Live 30" {
                n131 = shared-variable ".\\D05.lvlib\\D05thisVI"(error in=w343) -> (w347:refnum<vi>, error out=w346:errorcluster)
                n132 = invoke class="VI" method="FP.Open"(reference=w347, error in=w346, "Activate"=TRUE ("Activate?"), "State"=T8."Standard") -> (error out=w342:errorcluster)  [unwired: 1 in, 4 out]
              }
              frame "View" {
                n133 = shared-variable ".\\detectedPellet.lvlib\\open flag"(TRUE ("open flag"), error in=w350) -> (error out=w349:errorcluster)
                n134 = shared-variable ".\\detectedPellet.lvlib\\DetectedPelletThisVi"(error in=w349) -> (w352:refnum<vi>, error out=w353:errorcluster)
                n135 = invoke class="VI" method="FP.Open"(reference=w352, error in=w353, "Activate"=TRUE ("Activate?"), "State"=T8."Standard") -> (error out=w351:errorcluster)  [unwired: 1 in, 4 out]
              }
            }
            n136 = shared-variable ".\\Maintenance.lvlib\\error_62"(w314) -> ()  [unwired: 1 in, 1 out]
          }
          event "Info 01", "Info 02", "Info 03", "Info 04", "Info 05": Mouse Down {
            n137 = event-data() -> ("CtlRef"=w357:refnum<vi>)  [unwired: 1 in, 7 out]
            n138 = property class="Bool (strict)"(reference=w357) -> ("Label.Text"=w356:string)  [unwired: 1 in, 2 out]
            n139 = case shown="\"Info 26\", Default" w356 {
              frame "Info 26", Default {
                n140 = call "camera info.vi"("Disc Number"="Disc 26", "Camera Name"=T9 "disc26" ("Session In")) -> ()  [unwired: 10 in]
              }
              frame "Info 27" {
                n141 = call "camera info.vi"("Disc Number"="Disc 27", "Camera Name"=T9 "disc27" ("Session In")) -> ()  [unwired: 10 in]
              }
              frame "Info 28" {
                n142 = call "camera info.vi"("Disc Number"="Disc 28", "Camera Name"=T9 "disc28" ("Session In")) -> ()  [unwired: 10 in]
              }
              frame "Info 29" {
                n143 = call "camera info.vi"("Disc Number"="Disc 29", "Camera Name"=T9 "disc29" ("Session In")) -> ()  [unwired: 10 in]
              }
              frame "Info 30" {
                n144 = call "camera info.vi"("Disc Number"="Disc 30", "Camera Name"=T9 "disc30" ("Session In")) -> ()  [unwired: 10 in]
              }
            }
          }
          event "Warning 01", "Warning 02", "Warning 03", "Warning 04", "Warning 05": Mouse Down {
            n145 = event-data() -> ("CtlRef"=w370:refnum<vi>)  [unwired: 1 in, 7 out]
            n146 = property class="Bool (strict)"(reference=w370) -> (error out=w368:errorcluster, "Label.Text"=w369:string)  [unwired: 1 in, 1 out]
            n147 = case shown="\"Warning 26\", Default" w369 {
              tunnel: w368 -> [w371 w406 w441 w476 w511]
              frame "Warning 26", Default {
                n148 = property on="Warning array 01" class="Arr (strict)"(error in=w371) -> ("Value"=w373:bool[])  [unwired: 1 in, 2 out]
                n149 = Boolean Array To Number(Boolean array=w373) -> (number=w372:u32)
                n150 = case shown="15" w372 {
                  frame 0, Default {
                  }
                  frame 1 {
                    n151 = One Button Dialog(message="Warning1: Camera of disc 26 is off.") -> ()  [unwired: 1 in, 1 out]
                  }
                  frame 2 {
                    n152 = One Button Dialog(message="Warning2: Projector of disc 26 is off.") -> ()  [unwired: 1 in, 1 out]
                  }
                  frame 3 {
                    n153 = flat-sequence {
                      frame #0 {
                        n154 = One Button Dialog(message="Warning1: Camera of disc 26 is off.") -> ()  [unwired: 1 in, 1 out]
                      }
                      frame #1 {
                        n155 = One Button Dialog(message="Warning2: Projector of disc 26 is off.") -> ()  [unwired: 1 in, 1 out]
                      }
                    }
                  }
                  frame 4 {
                    n156 = One Button Dialog(message="Warning3: control mode of disc 26 is manual.") -> ()  [unwired: 1 in, 1 out]
                  }
                  frame 5 {
                    n157 = flat-sequence {
                      frame #0 {
                        n158 = One Button Dialog(message="Warning1: Camera of disc 26 is off.") -> ()  [unwired: 1 in, 1 out]
                      }
                      frame #1 {
                        n159 = One Button Dialog(message="Warning3: Control mode of disc 26 is manual.") -> ()  [unwired: 1 in, 1 out]
                      }
                    }
                  }
                  frame 6 {
                    n160 = flat-sequence {
                      frame #0 {
                        n161 = One Button Dialog(message="Warning2: Projector of disc 26 is off.") -> ()  [unwired: 1 in, 1 out]
                      }
                      frame #1 {
                        n162 = One Button Dialog(message="Warning3: Control mode of disc 26 is manual.") -> ()  [unwired: 1 in, 1 out]
                      }
                    }
                  }
                  frame 7 {
                    n163 = flat-sequence {
                      frame #0 {
                        n164 = One Button Dialog(message="Warning1: Camera of disc 26 is off.") -> ()  [unwired: 1 in, 1 out]
                      }
                      frame #1 {
                        n165 = One Button Dialog(message="Warning2: Projector of disc 26 is off.") -> ()  [unwired: 1 in, 1 out]
                      }
                      frame #2 {
                        n166 = One Button Dialog(message="Warning3: Control mode of disc 26 is manual.") -> ()  [unwired: 1 in, 1 out]
                      }
                    }
                  }
                  frame 8 {
                    n167 = One Button Dialog(message="Warning4: Disc 26 is stop.") -> ()  [unwired: 1 in, 1 out]
                  }
                  frame 9 {
                    n168 = flat-sequence {
                      frame #0 {
                        n169 = One Button Dialog(message="Warning1: Camera of disc 26 is off.") -> ()  [unwired: 1 in, 1 out]
                      }
                      frame #1 {
                        n170 = One Button Dialog(message="Warning4: Disc 26 is stop.") -> ()  [unwired: 1 in, 1 out]
                      }
                    }
                  }
                  frame 10 {
                    n171 = flat-sequence {
                      frame #0 {
                        n172 = One Button Dialog(message="Warning2: Projector of disc 26 is off.") -> ()  [unwired: 1 in, 1 out]
                      }
                      frame #1 {
                        n173 = One Button Dialog(message="Warning4: Disc 26 is stop.") -> ()  [unwired: 1 in, 1 out]
                      }
                    }
                  }
                  frame 11 {
                    n174 = flat-sequence {
                      frame #0 {
                        n175 = One Button Dialog(message="Warning1: Camera of disc 26 is off.") -> ()  [unwired: 1 in, 1 out]
                      }
                      frame #1 {
                        n176 = One Button Dialog(message="Warning2: Projector of disc 26 is off.") -> ()  [unwired: 1 in, 1 out]
                      }
                      frame #2 {
                        n177 = One Button Dialog(message="Warning4: Disc 26 is stop.") -> ()  [unwired: 1 in, 1 out]
                      }
                    }
                  }
                  frame 12 {
                    n178 = flat-sequence {
                      frame #0 {
                        n179 = One Button Dialog(message="Warning3: control mode of disc 26 is manual.") -> ()  [unwired: 1 in, 1 out]
                      }
                      frame #1 {
                        n180 = One Button Dialog(message="Warning4: Disc 26 is stop.") -> ()  [unwired: 1 in, 1 out]
                      }
                    }
                  }
                  frame 13 {
                    n181 = flat-sequence {
                      frame #0 {
                        n182 = One Button Dialog(message="Warning1: Camera of disc 26 is off.") -> ()  [unwired: 1 in, 1 out]
                      }
                      frame #1 {
                        n183 = One Button Dialog(message="Warning3: control mode of disc 26 is manual.") -> ()  [unwired: 1 in, 1 out]
                      }
                      frame #2 {
                        n184 = One Button Dialog(message="Warning4: Disc 26 is stop.") -> ()  [unwired: 1 in, 1 out]
                      }
                    }
                  }
                  frame 14 {
                    n185 = flat-sequence {
                      frame #0 {
                        n186 = One Button Dialog(message="Warning2: Projector of disc 26 is off.") -> ()  [unwired: 1 in, 1 out]
                      }
                      frame #1 {
                        n187 = One Button Dialog(message="Warning3: control mode of disc 26 is manual.") -> ()  [unwired: 1 in, 1 out]
                      }
                      frame #2 {
                        n188 = One Button Dialog(message="Warning4: Disc 26 is stop.") -> ()  [unwired: 1 in, 1 out]
                      }
                    }
                  }
                  frame 15 {
                    n189 = flat-sequence {
                      frame #0 {
                        n190 = One Button Dialog(message="Warning1: Camera of disc 26 is off.") -> ()  [unwired: 1 in, 1 out]
                      }
                      frame #1 {
                        n191 = One Button Dialog(message="Warning2: Projector of disc 26 is off.") -> ()  [unwired: 1 in, 1 out]
                      }
                      frame #2 {
                        n192 = One Button Dialog(message="Warning3: control mode of disc 26 is manual.") -> ()  [unwired: 1 in, 1 out]
                      }
                      frame #3 {
                        n193 = One Button Dialog(message="Warning4: Disc 26 is stop.") -> ()  [unwired: 1 in, 1 out]
                      }
                    }
                  }
                }
              }
              frame "Warning 27" {
                n194 = property on="Warning array 02" class="Arr (strict)"(error in=w406) -> ("Value"=w408:bool[])  [unwired: 1 in, 2 out]
                n195 = Boolean Array To Number(Boolean array=w408) -> (number=w407:u32)
                n196 = case shown="14" w407 {
                  frame 0, Default {
                  }
                  frame 1 {
                    n197 = One Button Dialog(message="Warning1: Camera of disc 27 is off.") -> ()  [unwired: 1 in, 1 out]
                  }
                  frame 2 {
                    n198 = One Button Dialog(message="Warning2: Projector of disc 27 is off.") -> ()  [unwired: 1 in, 1 out]
                  }
                  frame 3 {
                    n199 = flat-sequence {
                      frame #0 {
                        n200 = One Button Dialog(message="Warning1: Camera of disc 27 is off.") -> ()  [unwired: 1 in, 1 out]
                      }
                      frame #1 {
                        n201 = One Button Dialog(message="Warning2: Projector of disc 27 is off.") -> ()  [unwired: 1 in, 1 out]
                      }
                    }
                  }
                  frame 4 {
                    n202 = One Button Dialog(message="Warning3: control mode of disc 27 is manual.") -> ()  [unwired: 1 in, 1 out]
                  }
                  frame 5 {
                    n203 = flat-sequence {
                      frame #0 {
                        n204 = One Button Dialog(message="Warning1: Camera of disc 27 is off.") -> ()  [unwired: 1 in, 1 out]
                      }
                      frame #1 {
                        n205 = One Button Dialog(message="Warning3: Control mode of disc 27 is manual.") -> ()  [unwired: 1 in, 1 out]
                      }
                    }
                  }
                  frame 6 {
                    n206 = flat-sequence {
                      frame #0 {
                        n207 = One Button Dialog(message="Warning2: Projector of disc 27 is off.") -> ()  [unwired: 1 in, 1 out]
                      }
                      frame #1 {
                        n208 = One Button Dialog(message="Warning3: Control mode of disc 27 is manual.") -> ()  [unwired: 1 in, 1 out]
                      }
                    }
                  }
                  frame 7 {
                    n209 = flat-sequence {
                      frame #0 {
                        n210 = One Button Dialog(message="Warning1: Camera of disc 27 is off.") -> ()  [unwired: 1 in, 1 out]
                      }
                      frame #1 {
                        n211 = One Button Dialog(message="Warning2: Projector of disc 27 is off.") -> ()  [unwired: 1 in, 1 out]
                      }
                      frame #2 {
                        n212 = One Button Dialog(message="Warning3: Control mode of disc 27 is manual.") -> ()  [unwired: 1 in, 1 out]
                      }
                    }
                  }
                  frame 8 {
                    n213 = One Button Dialog(message="Warning4: Disc 27 is stop.") -> ()  [unwired: 1 in, 1 out]
                  }
                  frame 9 {
                    n214 = flat-sequence {
                      frame #0 {
                        n215 = One Button Dialog(message="Warning1: Camera of disc 27 is off.") -> ()  [unwired: 1 in, 1 out]
                      }
                      frame #1 {
                        n216 = One Button Dialog(message="Warning4: Disc 27 is stop.") -> ()  [unwired: 1 in, 1 out]
                      }
                    }
                  }
                  frame 10 {
                    n217 = flat-sequence {
                      frame #0 {
                        n218 = One Button Dialog(message="Warning2: Projector of disc 27 is off.") -> ()  [unwired: 1 in, 1 out]
                      }
                      frame #1 {
                        n219 = One Button Dialog(message="Warning4: Disc 27 is stop.") -> ()  [unwired: 1 in, 1 out]
                      }
                    }
                  }
                  frame 11 {
                    n220 = flat-sequence {
                      frame #0 {
                        n221 = One Button Dialog(message="Warning1: Camera of disc 27 is off.") -> ()  [unwired: 1 in, 1 out]
                      }
                      frame #1 {
                        n222 = One Button Dialog(message="Warning2: Projector of disc 27 is off.") -> ()  [unwired: 1 in, 1 out]
                      }
                      frame #2 {
                        n223 = One Button Dialog(message="Warning4: Disc 27 is stop.") -> ()  [unwired: 1 in, 1 out]
                      }
                    }
                  }
                  frame 12 {
                    n224 = flat-sequence {
                      frame #0 {
                        n225 = One Button Dialog(message="Warning3: control mode of disc 27 is manual.") -> ()  [unwired: 1 in, 1 out]
                      }
                      frame #1 {
                        n226 = One Button Dialog(message="Warning4: Disc 27 is stop.") -> ()  [unwired: 1 in, 1 out]
                      }
                    }
                  }
                  frame 13 {
                    n227 = flat-sequence {
                      frame #0 {
                        n228 = One Button Dialog(message="Warning1: Camera of disc 27 is off.") -> ()  [unwired: 1 in, 1 out]
                      }
                      frame #1 {
                        n229 = One Button Dialog(message="Warning3: control mode of disc 27 is manual.") -> ()  [unwired: 1 in, 1 out]
                      }
                      frame #2 {
                        n230 = One Button Dialog(message="Warning4: Disc 27 is stop.") -> ()  [unwired: 1 in, 1 out]
                      }
                    }
                  }
                  frame 14 {
                    n231 = flat-sequence {
                      frame #0 {
                        n232 = One Button Dialog(message="Warning2: Projector of disc 27 is off.") -> ()  [unwired: 1 in, 1 out]
                      }
                      frame #1 {
                        n233 = One Button Dialog(message="Warning3: control mode of disc 27 is manual.") -> ()  [unwired: 1 in, 1 out]
                      }
                      frame #2 {
                        n234 = One Button Dialog(message="Warning4: Disc 27 is stop.") -> ()  [unwired: 1 in, 1 out]
                      }
                    }
                  }
                  frame 15 {
                    n235 = flat-sequence {
                      frame #0 {
                        n236 = One Button Dialog(message="Warning1: Camera of disc 27 is off.") -> ()  [unwired: 1 in, 1 out]
                      }
                      frame #1 {
                        n237 = One Button Dialog(message="Warning2: Projector of disc 27 is off.") -> ()  [unwired: 1 in, 1 out]
                      }
                      frame #2 {
                        n238 = One Button Dialog(message="Warning3: control mode of disc 27 is manual.") -> ()  [unwired: 1 in, 1 out]
                      }
                      frame #3 {
                        n239 = One Button Dialog(message="Warning4: Disc 27 is stop.") -> ()  [unwired: 1 in, 1 out]
                      }
                    }
                  }
                }
              }
              frame "Warning 28" {
                n240 = property on="Warning array 03" class="Arr (strict)"(error in=w441) -> ("Value"=w443:bool[])  [unwired: 1 in, 2 out]
                n241 = Boolean Array To Number(Boolean array=w443) -> (number=w442:u32)
                n242 = case shown="0, Default" w442 {
                  frame 0, Default {
                  }
                  frame 1 {
                    n243 = One Button Dialog(message="Warning1: Camera of disc 28 is off.") -> ()  [unwired: 1 in, 1 out]
                  }
                  frame 2 {
                    n244 = One Button Dialog(message="Warning2: Projector of disc 28 is off.") -> ()  [unwired: 1 in, 1 out]
                  }
                  frame 3 {
                    n245 = flat-sequence {
                      frame #0 {
                        n246 = One Button Dialog(message="Warning1: Camera of disc 28 is off.") -> ()  [unwired: 1 in, 1 out]
                      }
                      frame #1 {
                        n247 = One Button Dialog(message="Warning2: Projector of disc 28 is off.") -> ()  [unwired: 1 in, 1 out]
                      }
                    }
                  }
                  frame 4 {
                    n248 = One Button Dialog(message="Warning3: control mode of disc 28 is manual.") -> ()  [unwired: 1 in, 1 out]
                  }
                  frame 5 {
                    n249 = flat-sequence {
                      frame #0 {
                        n250 = One Button Dialog(message="Warning1: Camera of disc 28 is off.") -> ()  [unwired: 1 in, 1 out]
                      }
                      frame #1 {
                        n251 = One Button Dialog(message="Warning3: Control mode of disc 28 is manual.") -> ()  [unwired: 1 in, 1 out]
                      }
                    }
                  }
                  frame 6 {
                    n252 = flat-sequence {
                      frame #0 {
                        n253 = One Button Dialog(message="Warning2: Projector of disc 28 is off.") -> ()  [unwired: 1 in, 1 out]
                      }
                      frame #1 {
                        n254 = One Button Dialog(message="Warning3: Control mode of disc 28 is manual.") -> ()  [unwired: 1 in, 1 out]
                      }
                    }
                  }
                  frame 7 {
                    n255 = flat-sequence {
                      frame #0 {
                        n256 = One Button Dialog(message="Warning1: Camera of disc 28 is off.") -> ()  [unwired: 1 in, 1 out]
                      }
                      frame #1 {
                        n257 = One Button Dialog(message="Warning2: Projector of disc 28 is off.") -> ()  [unwired: 1 in, 1 out]
                      }
                      frame #2 {
                        n258 = One Button Dialog(message="Warning3: Control mode of disc 28 is manual.") -> ()  [unwired: 1 in, 1 out]
                      }
                    }
                  }
                  frame 8 {
                    n259 = One Button Dialog(message="Warning4: Disc 28 is stop.") -> ()  [unwired: 1 in, 1 out]
                  }
                  frame 9 {
                    n260 = flat-sequence {
                      frame #0 {
                        n261 = One Button Dialog(message="Warning1: Camera of disc 28 is off.") -> ()  [unwired: 1 in, 1 out]
                      }
                      frame #1 {
                        n262 = One Button Dialog(message="Warning4: Disc 28 is stop.") -> ()  [unwired: 1 in, 1 out]
                      }
                    }
                  }
                  frame 10 {
                    n263 = flat-sequence {
                      frame #0 {
                        n264 = One Button Dialog(message="Warning2: Projector of disc 28 is off.") -> ()  [unwired: 1 in, 1 out]
                      }
                      frame #1 {
                        n265 = One Button Dialog(message="Warning4: Disc 28 is stop.") -> ()  [unwired: 1 in, 1 out]
                      }
                    }
                  }
                  frame 11 {
                    n266 = flat-sequence {
                      frame #0 {
                        n267 = One Button Dialog(message="Warning1: Camera of disc 28 is off.") -> ()  [unwired: 1 in, 1 out]
                      }
                      frame #1 {
                        n268 = One Button Dialog(message="Warning2: Projector of disc 28 is off.") -> ()  [unwired: 1 in, 1 out]
                      }
                      frame #2 {
                        n269 = One Button Dialog(message="Warning4: Disc 28 is stop.") -> ()  [unwired: 1 in, 1 out]
                      }
                    }
                  }
                  frame 12 {
                    n270 = flat-sequence {
                      frame #0 {
                        n271 = One Button Dialog(message="Warning3: control mode of disc 28 is manual.") -> ()  [unwired: 1 in, 1 out]
                      }
                      frame #1 {
                        n272 = One Button Dialog(message="Warning4: Disc 28 is stop.") -> ()  [unwired: 1 in, 1 out]
                      }
                    }
                  }
                  frame 13 {
                    n273 = flat-sequence {
                      frame #0 {
                        n274 = One Button Dialog(message="Warning1: Camera of disc 28 is off.") -> ()  [unwired: 1 in, 1 out]
                      }
                      frame #1 {
                        n275 = One Button Dialog(message="Warning3: control mode of disc 28 is manual.") -> ()  [unwired: 1 in, 1 out]
                      }
                      frame #2 {
                        n276 = One Button Dialog(message="Warning4: Disc 28 is stop.") -> ()  [unwired: 1 in, 1 out]
                      }
                    }
                  }
                  frame 14 {
                    n277 = flat-sequence {
                      frame #0 {
                        n278 = One Button Dialog(message="Warning2: Projector of disc 28 is off.") -> ()  [unwired: 1 in, 1 out]
                      }
                      frame #1 {
                        n279 = One Button Dialog(message="Warning3: control mode of disc 28 is manual.") -> ()  [unwired: 1 in, 1 out]
                      }
                      frame #2 {
                        n280 = One Button Dialog(message="Warning4: Disc 28 is stop.") -> ()  [unwired: 1 in, 1 out]
                      }
                    }
                  }
                  frame 15 {
                    n281 = flat-sequence {
                      frame #0 {
                        n282 = One Button Dialog(message="Warning1: Camera of disc 28 is off.") -> ()  [unwired: 1 in, 1 out]
                      }
                      frame #1 {
                        n283 = One Button Dialog(message="Warning2: Projector of disc 28 is off.") -> ()  [unwired: 1 in, 1 out]
                      }
                      frame #2 {
                        n284 = One Button Dialog(message="Warning3: control mode of disc 28 is manual.") -> ()  [unwired: 1 in, 1 out]
                      }
                      frame #3 {
                        n285 = One Button Dialog(message="Warning4: Disc 28 is stop.") -> ()  [unwired: 1 in, 1 out]
                      }
                    }
                  }
                }
              }
              frame "Warning 29" {
                n286 = property on="Warning array 04" class="Arr (strict)"(error in=w476) -> ("Value"=w478:bool[])  [unwired: 1 in, 2 out]
                n287 = Boolean Array To Number(Boolean array=w478) -> (number=w477:u32)
                n288 = case shown="0, Default" w477 {
                  frame 0, Default {
                  }
                  frame 1 {
                    n289 = One Button Dialog(message="Warning1: Camera of disc 29 is off.") -> ()  [unwired: 1 in, 1 out]
                  }
                  frame 2 {
                    n290 = One Button Dialog(message="Warning2: Projector of disc 29 is off.") -> ()  [unwired: 1 in, 1 out]
                  }
                  frame 3 {
                    n291 = flat-sequence {
                      frame #0 {
                        n292 = One Button Dialog(message="Warning1: Camera of disc 29 is off.") -> ()  [unwired: 1 in, 1 out]
                      }
                      frame #1 {
                        n293 = One Button Dialog(message="Warning2: Projector of disc 29 is off.") -> ()  [unwired: 1 in, 1 out]
                      }
                    }
                  }
                  frame 4 {
                    n294 = One Button Dialog(message="Warning3: control mode of disc 29 is manual.") -> ()  [unwired: 1 in, 1 out]
                  }
                  frame 5 {
                    n295 = flat-sequence {
                      frame #0 {
                        n296 = One Button Dialog(message="Warning1: Camera of disc 29 is off.") -> ()  [unwired: 1 in, 1 out]
                      }
                      frame #1 {
                        n297 = One Button Dialog(message="Warning3: Control mode of disc 29 is manual.") -> ()  [unwired: 1 in, 1 out]
                      }
                    }
                  }
                  frame 6 {
                    n298 = flat-sequence {
                      frame #0 {
                        n299 = One Button Dialog(message="Warning2: Projector of disc 29 is off.") -> ()  [unwired: 1 in, 1 out]
                      }
                      frame #1 {
                        n300 = One Button Dialog(message="Warning3: Control mode of disc 29 is manual.") -> ()  [unwired: 1 in, 1 out]
                      }
                    }
                  }
                  frame 7 {
                    n301 = flat-sequence {
                      frame #0 {
                        n302 = One Button Dialog(message="Warning1: Camera of disc 29 is off.") -> ()  [unwired: 1 in, 1 out]
                      }
                      frame #1 {
                        n303 = One Button Dialog(message="Warning2: Projector of disc 29 is off.") -> ()  [unwired: 1 in, 1 out]
                      }
                      frame #2 {
                        n304 = One Button Dialog(message="Warning3: Control mode of disc 29 is manual.") -> ()  [unwired: 1 in, 1 out]
                      }
                    }
                  }
                  frame 8 {
                    n305 = One Button Dialog(message="Warning4: Disc 29 is stop.") -> ()  [unwired: 1 in, 1 out]
                  }
                  frame 9 {
                    n306 = flat-sequence {
                      frame #0 {
                        n307 = One Button Dialog(message="Warning1: Camera of disc 29 is off.") -> ()  [unwired: 1 in, 1 out]
                      }
                      frame #1 {
                        n308 = One Button Dialog(message="Warning4: Disc 29 is stop.") -> ()  [unwired: 1 in, 1 out]
                      }
                    }
                  }
                  frame 10 {
                    n309 = flat-sequence {
                      frame #0 {
                        n310 = One Button Dialog(message="Warning2: Projector of disc 29 is off.") -> ()  [unwired: 1 in, 1 out]
                      }
                      frame #1 {
                        n311 = One Button Dialog(message="Warning4: Disc 29 is stop.") -> ()  [unwired: 1 in, 1 out]
                      }
                    }
                  }
                  frame 11 {
                    n312 = flat-sequence {
                      frame #0 {
                        n313 = One Button Dialog(message="Warning1: Camera of disc 29 is off.") -> ()  [unwired: 1 in, 1 out]
                      }
                      frame #1 {
                        n314 = One Button Dialog(message="Warning2: Projector of disc 29 is off.") -> ()  [unwired: 1 in, 1 out]
                      }
                      frame #2 {
                        n315 = One Button Dialog(message="Warning4: Disc 29 is stop.") -> ()  [unwired: 1 in, 1 out]
                      }
                    }
                  }
                  frame 12 {
                    n316 = flat-sequence {
                      frame #0 {
                        n317 = One Button Dialog(message="Warning3: control mode of disc 29 is manual.") -> ()  [unwired: 1 in, 1 out]
                      }
                      frame #1 {
                        n318 = One Button Dialog(message="Warning4: Disc 29 is stop.") -> ()  [unwired: 1 in, 1 out]
                      }
                    }
                  }
                  frame 13 {
                    n319 = flat-sequence {
                      frame #0 {
                        n320 = One Button Dialog(message="Warning1: Camera of disc 29 is off.") -> ()  [unwired: 1 in, 1 out]
                      }
                      frame #1 {
                        n321 = One Button Dialog(message="Warning3: control mode of disc 29 is manual.") -> ()  [unwired: 1 in, 1 out]
                      }
                      frame #2 {
                        n322 = One Button Dialog(message="Warning4: Disc 29 is stop.") -> ()  [unwired: 1 in, 1 out]
                      }
                    }
                  }
                  frame 14 {
                    n323 = flat-sequence {
                      frame #0 {
                        n324 = One Button Dialog(message="Warning2: Projector of disc 29 is off.") -> ()  [unwired: 1 in, 1 out]
                      }
                      frame #1 {
                        n325 = One Button Dialog(message="Warning3: control mode of disc 29 is manual.") -> ()  [unwired: 1 in, 1 out]
                      }
                      frame #2 {
                        n326 = One Button Dialog(message="Warning4: Disc 29 is stop.") -> ()  [unwired: 1 in, 1 out]
                      }
                    }
                  }
                  frame 15 {
                    n327 = flat-sequence {
                      frame #0 {
                        n328 = One Button Dialog(message="Warning1: Camera of disc 29 is off.") -> ()  [unwired: 1 in, 1 out]
                      }
                      frame #1 {
                        n329 = One Button Dialog(message="Warning2: Projector of disc 29 is off.") -> ()  [unwired: 1 in, 1 out]
                      }
                      frame #2 {
                        n330 = One Button Dialog(message="Warning3: control mode of disc 29 is manual.") -> ()  [unwired: 1 in, 1 out]
                      }
                      frame #3 {
                        n331 = One Button Dialog(message="Warning4: Disc 29 is stop.") -> ()  [unwired: 1 in, 1 out]
                      }
                    }
                  }
                }
              }
              frame "Warning 30" {
                n332 = property on="Warning array 05" class="Arr (strict)"(error in=w511) -> ("Value"=w513:bool[])  [unwired: 1 in, 2 out]
                n333 = Boolean Array To Number(Boolean array=w513) -> (number=w512:u32)
                n334 = case shown="14" w512 {
                  frame 0, Default {
                  }
                  frame 1 {
                    n335 = One Button Dialog(message="Warning1: Camera of disc 30 is off.") -> ()  [unwired: 1 in, 1 out]
                  }
                  frame 2 {
                    n336 = One Button Dialog(message="Warning2: Projector of disc 30 is off.") -> ()  [unwired: 1 in, 1 out]
                  }
                  frame 3 {
                    n337 = flat-sequence {
                      frame #0 {
                        n338 = One Button Dialog(message="Warning1: Camera of disc 30 is off.") -> ()  [unwired: 1 in, 1 out]
                      }
                      frame #1 {
                        n339 = One Button Dialog(message="Warning2: Projector of disc 30 is off.") -> ()  [unwired: 1 in, 1 out]
                      }
                    }
                  }
                  frame 4 {
                    n340 = One Button Dialog(message="Warning3: control mode of disc 30 is manual.") -> ()  [unwired: 1 in, 1 out]
                  }
                  frame 5 {
                    n341 = flat-sequence {
                      frame #0 {
                        n342 = One Button Dialog(message="Warning1: Camera of disc 30 is off.") -> ()  [unwired: 1 in, 1 out]
                      }
                      frame #1 {
                        n343 = One Button Dialog(message="Warning3: Control mode of disc 30 is manual.") -> ()  [unwired: 1 in, 1 out]
                      }
                    }
                  }
                  frame 6 {
                    n344 = flat-sequence {
                      frame #0 {
                        n345 = One Button Dialog(message="Warning2: Projector of disc 30 is off.") -> ()  [unwired: 1 in, 1 out]
                      }
                      frame #1 {
                        n346 = One Button Dialog(message="Warning3: Control mode of disc 30 is manual.") -> ()  [unwired: 1 in, 1 out]
                      }
                    }
                  }
                  frame 7 {
                    n347 = flat-sequence {
                      frame #0 {
                        n348 = One Button Dialog(message="Warning1: Camera of disc 30 is off.") -> ()  [unwired: 1 in, 1 out]
                      }
                      frame #1 {
                        n349 = One Button Dialog(message="Warning2: Projector of disc 30 is off.") -> ()  [unwired: 1 in, 1 out]
                      }
                      frame #2 {
                        n350 = One Button Dialog(message="Warning3: Control mode of disc 30 is manual.") -> ()  [unwired: 1 in, 1 out]
                      }
                    }
                  }
                  frame 8 {
                    n351 = One Button Dialog(message="Warning4: Disc 30 is stop.") -> ()  [unwired: 1 in, 1 out]
                  }
                  frame 9 {
                    n352 = flat-sequence {
                      frame #0 {
                        n353 = One Button Dialog(message="Warning1: Camera of disc 30 is off.") -> ()  [unwired: 1 in, 1 out]
                      }
                      frame #1 {
                        n354 = One Button Dialog(message="Warning4: Disc 30 is stop.") -> ()  [unwired: 1 in, 1 out]
                      }
                    }
                  }
                  frame 10 {
                    n355 = flat-sequence {
                      frame #0 {
                        n356 = One Button Dialog(message="Warning2: Projector of disc 30 is off.") -> ()  [unwired: 1 in, 1 out]
                      }
                      frame #1 {
                        n357 = One Button Dialog(message="Warning4: Disc 30 is stop.") -> ()  [unwired: 1 in, 1 out]
                      }
                    }
                  }
                  frame 11 {
                    n358 = flat-sequence {
                      frame #0 {
                        n359 = One Button Dialog(message="Warning1: Camera of disc 30 is off.") -> ()  [unwired: 1 in, 1 out]
                      }
                      frame #1 {
                        n360 = One Button Dialog(message="Warning2: Projector of disc 30 is off.") -> ()  [unwired: 1 in, 1 out]
                      }
                      frame #2 {
                        n361 = One Button Dialog(message="Warning4: Disc 30 is stop.") -> ()  [unwired: 1 in, 1 out]
                      }
                    }
                  }
                  frame 12 {
                    n362 = flat-sequence {
                      frame #0 {
                        n363 = One Button Dialog(message="Warning3: control mode of disc 30 is manual.") -> ()  [unwired: 1 in, 1 out]
                      }
                      frame #1 {
                        n364 = One Button Dialog(message="Warning4: Disc 30 is stop.") -> ()  [unwired: 1 in, 1 out]
                      }
                    }
                  }
                  frame 13 {
                    n365 = flat-sequence {
                      frame #0 {
                        n366 = One Button Dialog(message="Warning1: Camera of disc 30 is off.") -> ()  [unwired: 1 in, 1 out]
                      }
                      frame #1 {
                        n367 = One Button Dialog(message="Warning3: control mode of disc 30 is manual.") -> ()  [unwired: 1 in, 1 out]
                      }
                      frame #2 {
                        n368 = One Button Dialog(message="Warning4: Disc 30 is stop.") -> ()  [unwired: 1 in, 1 out]
                      }
                    }
                  }
                  frame 14 {
                    n369 = flat-sequence {
                      frame #0 {
                        n370 = One Button Dialog(message="Warning2: Projector of disc 30 is off.") -> ()  [unwired: 1 in, 1 out]
                      }
                      frame #1 {
                        n371 = One Button Dialog(message="Warning3: control mode of disc 30 is manual.") -> ()  [unwired: 1 in, 1 out]
                      }
                      frame #2 {
                        n372 = One Button Dialog(message="Warning4: Disc 30 is stop.") -> ()  [unwired: 1 in, 1 out]
                      }
                    }
                  }
                  frame 15 {
                    n373 = flat-sequence {
                      frame #0 {
                        n374 = One Button Dialog(message="Warning1: Camera of disc 30 is off.") -> ()  [unwired: 1 in, 1 out]
                      }
                      frame #1 {
                        n375 = One Button Dialog(message="Warning2: Projector of disc 30 is off.") -> ()  [unwired: 1 in, 1 out]
                      }
                      frame #2 {
                        n376 = One Button Dialog(message="Warning3: control mode of disc 30 is manual.") -> ()  [unwired: 1 in, 1 out]
                      }
                      frame #3 {
                        n377 = One Button Dialog(message="Warning4: Disc 30 is stop.") -> ()  [unwired: 1 in, 1 out]
                      }
                    }
                  }
                }
              }
            }
          }
          event Timeout {
            w579 = 4
            n378 = event-data() -> ()  [unwired: 1 in, 3 out]
            n379 = call-poly <userlib>:"DAQNavi Read.vi"("error in (no error)"=w594, "task in"=w595) -> ("error out"=→"error out 14":errorcluster, "data"=w608:u8[])  [unwired: 7 in, 1 out]
            n380 = call-poly <userlib>:"DAQNavi Read.vi"("error in (no error)"=w609, "task in"=w610) -> ("error out"=→"error out 12":errorcluster, "data"=w582:dbl[])  [unwired: 7 in, 1 out]
            n381 = shared-variable ".\\User Lib.lvlib\\Cancel Login"() -> (w617:bool, error out=w613:errorcluster)  [unwired: 1 in]
            n382 = Get Date/Time In Seconds() -> (seconds since 1Jan1904=w616:timestamp)
            n383 = case shown="True" w617 {
              tunnel: w613 -> [_ w624]
              frame False {
              }
              frame True {
                n384 = property on="Login" class="Bool (strict)"(error in=w624, "Value"=TRUE ("Login")) -> ()  [unwired: 1 in, 2 out]
              }
            }
            n385 = Format Date/Time String(time format string (%c)="%Y/%m/%d  %H:%M:%S", seconds (now)=w616) -> (date/time string=→"time&date":string)  [unwired: 1 in]
            n386 = Index Array(array=w608, index #1=0 ("index")) -> (element #1=w602:u8, element #2=w606:u8)  [unwired: 1 in]
            n387 = Multiply(x=w582, y=w579) -> (x*y=w581:dbl[])
            n388 = Number To Boolean Array(number=w602) -> (Boolean array=w605:bool[])
            n389 = Number To Boolean Array(number=w606) -> (Boolean array=w603:bool[])
            n390 = Round To Nearest(number=w581) -> (nearest integer value=w580:dbl[])
            n391 = shared-variable ".\\User Lib.lvlib\\Is Dorsa?"() -> (w611:bool)  [unwired: 1 in, 1 out]
            n392 = shared-variable ".\\User Lib.lvlib\\User Flag"() -> (w612:bool)  [unwired: 1 in, 1 out]
            n393 = Index Array(array=w603) -> (element #1=w556:bool, element #2=w555:bool, element #3=w554:bool, element #4=w552:bool)  [unwired: 4 in]
            n394 = Index Array(array=w605, index #1=0 ("index")) -> (element #1=w599:bool, element #2=w598:bool, element #3=w597:bool, element #4=w596:bool, element #5=w600:bool, element #6=w558:bool, element #7=w560:bool, element #8=w559:bool)  [unwired: 7 in]
            n395 = Divide(x=w580, y=w579) -> (x/y=w561:dbl[])
            n396 = Not(x=w599) -> (.not. x?=→"DISC 01":bool)
            n397 = Not(x=w598) -> (.not. x?=→"DISC 02":bool)
            n398 = Not(x=w597) -> (.not. x?=→"DISC 03":bool)
            n399 = Not(x=w596) -> (.not. x?=→"DISC 04":bool)
            n400 = Not(x=w600) -> (.not. x?=→"DISC 05":bool)
            n401 = Not(x=w558) -> (.not. x?=→"DISC 06":bool)
            n402 = Not(x=w560) -> (.not. x?=→"AUTO/MAN 01":bool)
            n403 = Not(x=w559) -> (.not. x?=→"AUTO/MAN 02":bool)
            n404 = Not(x=w556) -> (.not. x?=→"AUTO/MAN 03":bool)
            n405 = Not(x=w555) -> (.not. x?=→"AUTO/MAN 04":bool)
            n406 = Not(x=w554) -> (.not. x?=→"AUTO/MAN 05":bool)
            n407 = Not(x=w552) -> (.not. x?=→"AUTO/MAN 06":bool)
            n408 = case shown="False" w612 {
              frame False {
                n409 = property on="Setting" class="Bool (strict)"("DisabledEnum"=T10."Disabled and Grayed Out" ("Disabled")) -> ()  [unwired: 2 in, 2 out]
                n410 = property on="Report" class="Bool (strict)"("DisabledEnum"=T10."Disabled and Grayed Out" ("Disabled")) -> ()  [unwired: 2 in, 2 out]
              }
              frame True {
                n411 = property on="Report" class="Bool (strict)"("DisabledEnum"=T10."Enabled" ("Disabled")) -> ()  [unwired: 2 in, 2 out]
                n412 = property on="Setting" class="Bool (strict)"("DisabledEnum"=T10."Enabled" ("Disabled")) -> ()  [unwired: 2 in, 2 out]
              }
            }
            n413 = case shown="False" w611 {
              frame False {
                n414 = property on="Maintenance" class="Bool (strict)"("DisabledEnum"=T10."Disabled and Grayed Out" ("Disabled")) -> ()  [unwired: 2 in, 2 out]
              }
              frame True {
                n415 = property on="Maintenance" class="Bool (strict)"("DisabledEnum"=T10."Enabled" ("Disabled")) -> ()  [unwired: 2 in, 2 out]
              }
            }
            n416 = shared-variable ".\\trends.lvlib\\SpeedArray"(w561) -> ()  [unwired: 1 in, 1 out]
            n417 = Index Array(array=w561, index #1=0 ("index")) -> (element #1=w574:dbl, element #2=w573:dbl, element #3=w572:dbl, element #4=w571:dbl, element #5=w570:dbl, element #6=w548:dbl)  [unwired: 5 in]
            "SPEED 01" <- w574
            "SPEED 02" <- w573
            "SPEED 03" <- w572
            "SPEED 04" <- w571
            "SPEED 05" <- w570
            "SPEED 06" <- w548
            n418 = shared-variable ".\\control setting.lvlib\\SpeedLimit"() -> (w578:dbl[])  [unwired: 1 in, 1 out]
            n419 = Index Array(array=w578, index #1=0 ("index")) -> (element #1=w546:dbl, element #2=w547:dbl)  [unwired: 1 in]
            n420 = Less Or Equal?(x=w574, y=w547) -> (x <= y?=→"speed  min 01":bool)
            n421 = Greater Or Equal?(x=w574, y=w546) -> (x >= y?=→"speed max 01":bool)
            n422 = Less Or Equal?(x=w573, y=w547) -> (x <= y?=→"speed  min 02":bool)
            n423 = Greater Or Equal?(x=w573, y=w546) -> (x >= y?=→"speed max 02":bool)
            n424 = Less Or Equal?(x=w572, y=w547) -> (x <= y?=→"speed  min 03":bool)
            n425 = Greater Or Equal?(x=w572, y=w546) -> (x >= y?=→"speed max 03":bool)
            n426 = Less Or Equal?(x=w571, y=w547) -> (x <= y?=→"speed  min 04":bool)
            n427 = Greater Or Equal?(x=w571, y=w546) -> (x >= y?=→"speed max 04":bool)
            n428 = Less Or Equal?(x=w570, y=w547) -> (x <= y?=→"speed  min 05":bool)
            n429 = Greater Or Equal?(x=w570, y=w546) -> (x >= y?=→"speed max 05":bool)
            n430 = Less Or Equal?(x=w548, y=w547) -> (x <= y?=→"speed  min 06":bool)
            n431 = Greater Or Equal?(x=w548, y=w546) -> (x >= y?=→"speed max 06":bool)
          }
        }
        n432 = Wait (ms)(milliseconds to wait=u32 100) -> ()  [unwired: 1 out]
      }
      "Software name" <- "DORSA Smart Grading System (DSGS)" ("time format string (%c)")
      "disc name 01" <- "DISC 01" ("disc 26 name")
      "disc name 02" <- "DISC 02" ("disc name 27")
      "disc name 03" <- "DISC 03" ("disc name 28")
      "disc name 04" <- "DISC 04" ("disc name 29")
      "disc name 05" <- "DISC 05" ("disc name 30")
      "overal result" <- "Overal Result" ("overal result")
    }
    frame Enabled {
    }
  }
  n433 = Initialize Array(0.0 ("element"), w80, 5 ("dimension size")) -> (w81:dbl[][])
  n434 = call "IMAQ Create"("Image Name"="img out D05") -> ("New Image"=w88:T7, "error out"=w35:errorcluster)  [unwired: 4 in]
  n435 = shared-variable ".\\Maintenance.lvlib\\error_11"(w35) -> ()  [unwired: 1 in, 1 out]
  n436 = Initialize Array(0.0 ("element"), w85, 5 ("dimension size")) -> (w86:dbl[][])
  n437 = Open Python Session(python version="3.6" ("Python version"), 3:errorcluster {"status"=FALSE, "code"=0, "source"=""} ("error in (no error)")) -> (session out=w103:refnum<k35>, error out=w45:errorcluster)  [unwired: 1 in]
  n438 = shared-variable ".\\Maintenance.lvlib\\error_1"(w45) -> ()  [unwired: 1 in, 1 out]
  n439 = Initialize Array(12.0 ("element"), 24 ("dimension size"), 6 ("dimension size")) -> (w79:dbl[][])
  n440 = Initialize Array(0.0 ("element"), 600 ("dimension size"), 3 ("dimension size")) -> (w98:dbl[][])
  n441 = call "IMAQ Create"("Image Name"="img out D05") -> ("New Image"=w4:T7)  [unwired: 4 in, 1 out]
  n442 = Initialize Array(T6 {"disc 01"=FALSE, "auto/man 01"=FALSE, "projector 01"=FALSE, "cam 01"=FALSE}, 2 ("dimension size")) -> (w72:T13)
  n443 = Initialize Array(T5 {"disc 02"=FALSE, "auto/man 02"=FALSE, "projector 02"=FALSE, "cam 02"=FALSE}, 2 ("dimension size")) -> (w69:T14)
  n444 = Initialize Array(T1 {"disc 06"=FALSE, "auto/man 06"=FALSE, "projector 06"=FALSE, "cam 06"=FALSE}, 2 ("dimension size")) -> (w1:T15)
  n445 = Initialize Array(T2 {"disc 05"=FALSE, "auto/man 05"=FALSE, "projector 05"=FALSE, "cam 05"=FALSE}, 2 ("dimension size")) -> (w60:T16)
  n446 = Initialize Array(T4 {"disc 03"=FALSE, "auto/man 03"=FALSE, "projector 03"=FALSE, "cam 03"=FALSE}, 2 ("dimension size")) -> (w64:T17)
  n447 = Initialize Array(T3 {"disc 04"=FALSE, "auto/man 04"=FALSE, "projector 04"=FALSE, "cam 04"=FALSE}, 2 ("dimension size")) -> (w63:T18)
  n448 = while {
    tunnel: w103 -> [w1264]
    tunnel: w98 -> [w1263]
    tunnel: [w1262] -> w97
    tunnel: w96 -> [w1261]
    tunnel: w94 -> [w1260]
    tunnel: w92 -> [w1259]
    tunnel: w89 -> [w1257]
    tunnel: w88 -> [w1256]
    shift-right: [w1254] -> _
    shift-left: w86 -> [w1255]
    shift-right: [w1252] -> _
    shift-left: w81 -> [w1253]
    shift-right: [w1250] -> _
    shift-left: w79 -> [w1251]
    shift-right: [w1248] -> _
    shift-left: w72 -> [w1249]
    shift-right: [w1244] -> _
    shift-left: w69 -> [w1247]
    shift-right: [w1243] -> _
    shift-left: w63 -> [w1245]
    shift-right: [w1242] -> _
    shift-left: w64 -> [w1246]
    shift-right: [w1240] -> _
    shift-left: w60 -> [w1241]
    tunnel: w53 -> [w988]
    tunnel: w27 -> [w986]
    tunnel: w48 -> [w979]
    tunnel: w47 -> [w970]
    tunnel: w46 -> [w956]
    tunnel: w6 -> [w755]
    tunnel: w4 -> [w728]
    shift-right: [w626] -> _
    shift-left: w1 -> [w662]
    stop <- FALSE stop-if-true
    n449 = Wait (ms)(milliseconds to wait=u32 5) -> ()  [unwired: 1 out]
    n450 = flat-sequence {
      tunnel: w1249 -> [w1353]
      tunnel: w1251 -> [w1368]
      tunnel: w1253 -> [w1369]
      tunnel: w1255 -> [w1370]
      tunnel: w1256 -> [w1371]
      tunnel: w1257 -> [w1372]
      tunnel: w1259 -> [w1373]
      tunnel: w1260 -> [w1374]
      tunnel: w1264 -> [w1375]
      tunnel: w1261 -> [w1376]
      tunnel: w1263 -> [w1377]
      tunnel: [w1377] -> w1238
      tunnel: [w1376] -> w1237
      tunnel: [w1375] -> w1236
      tunnel: [w1374] -> w1235
      tunnel: [w1373] -> w1234
      tunnel: [w1372] -> w1233
      tunnel: [w1371] -> w1232
      tunnel: [w1370] -> w1231
      tunnel: [w1369] -> w1230
      tunnel: [w1368] -> w1229
      tunnel: [w1357] -> w1228
      tunnel: [w1356] -> w1227
      tunnel: [w1355] -> w1226
      tunnel: [w1354] -> w1225
      tunnel: [w1353] -> w1224
      tunnel: w1247 -> [w1306]
      tunnel: [w1340] -> w1223
      tunnel: [w1339] -> w1222
      tunnel: [w1338] -> w1221
      tunnel: [w1337] -> w1220
      tunnel: w1246 -> [w1305]
      tunnel: w1245 -> [w1304]
      tunnel: [w1314] -> w1219
      tunnel: [w1313] -> w1218
      tunnel: [w1312] -> w1217
      tunnel: [w1311] -> w1216
      tunnel: [w1310] -> w1215
      tunnel: [w1309] -> w1214
      tunnel: [w1308] -> w1213
      tunnel: [w1307] -> w1212
      tunnel: [w1306] -> w1211
      tunnel: [w1305] -> w1210
      tunnel: [w1304] -> w1209
      tunnel: w1241 -> [w1292]
      tunnel: [w1292] -> w1208
      tunnel: [w1291] -> w1207
      tunnel: [w1290] -> w1206
      tunnel: [w1289] -> w1205
      tunnel: [w1288] -> w1204
      tunnel: [w1287] -> w989
      tunnel: w988 -> [w1287]
      tunnel: [w1286] -> w987
      tunnel: w986 -> [w1286]
      tunnel: [w1285] -> w980
      tunnel: w979 -> [w1285]
      tunnel: w970 -> [w1284]
      tunnel: [w1284] -> w969
      tunnel: [w1283] -> w957
      tunnel: w956 -> [w1283]
      tunnel: [w1282] -> w756
      tunnel: w755 -> [w1282]
      tunnel: w728 -> [w1281]
      tunnel: [w1281] -> w701
      tunnel: w662 -> [w1265]
      tunnel: [w1269] -> w661
      tunnel: [w1268] -> w660
      tunnel: [w1267] -> w659
      tunnel: [w1266] -> w658
      tunnel: [w1265] -> w656
      tunnel: w1238 -> [w1442]
      tunnel: [w1442] -> w796
      tunnel: w1237 -> [w1441]
      tunnel: [w1441] -> w795
      tunnel: w1236 -> [w1440]
      tunnel: [w1440] -> w794
      tunnel: w1235 -> [w1439]
      tunnel: [w1439] -> w793
      tunnel: w1234 -> [w1438]
      tunnel: [w1438] -> w792
      tunnel: w1233 -> [w1437]
      tunnel: [w1437] -> w791
      tunnel: w1232 -> [w1436]
      tunnel: [w1436] -> w790
      tunnel: w1231 -> [w1435]
      tunnel: [w1435] -> w789
      tunnel: w1230 -> [w1434]
      tunnel: [w1434] -> w788
      tunnel: w1229 -> [w1433]
      tunnel: [w1433] -> w787
      tunnel: w1228 -> [w1410]
      tunnel: w1227 -> [w1409]
      tunnel: w1226 -> [w1408]
      tunnel: w1225 -> [w1411]
      tunnel: w1224 -> [w1432]
      tunnel: [w1432] -> w786
      tunnel: w1223 -> [w1418]
      tunnel: w1222 -> [w1416]
      tunnel: w1221 -> [w1417]
      tunnel: w1220 -> [w1419]
      tunnel: w1219 -> [w1421]
      tunnel: w1218 -> [w1423]
      tunnel: w1217 -> [w1422]
      tunnel: w1216 -> [w1420]
      tunnel: w1215 -> [w1412]
      tunnel: w1214 -> [w1415]
      tunnel: w1213 -> [w1414]
      tunnel: w1212 -> [w1413]
      tunnel: w1211 -> [w1431]
      tunnel: [w1431] -> w785
      tunnel: w1210 -> [w1430]
      tunnel: [w1430] -> w784
      tunnel: w1209 -> [w1429]
      tunnel: [w1429] -> w783
      tunnel: w1208 -> [w1428]
      tunnel: [w1428] -> w782
      tunnel: w1207 -> [w1427]
      tunnel: w1206 -> [w1426]
      tunnel: w1205 -> [w1425]
      tunnel: w1204 -> [w1424]
      tunnel: w989 -> [w1392]
      tunnel: [w1392] -> w781
      tunnel: w987 -> [w1391]
      tunnel: [w1391] -> w780
      tunnel: w980 -> [w1390]
      tunnel: [w1390] -> w779
      tunnel: [w1389] -> w778
      tunnel: w969 -> [w1389]
      tunnel: w957 -> [w1388]
      tunnel: [w1388] -> w777
      tunnel: w756 -> [w1387]
      tunnel: [w1387] -> w729
      tunnel: [w1386] -> w702
      tunnel: w701 -> [w1386]
      tunnel: w661 -> [w1382]
      tunnel: w660 -> [w1381]
      tunnel: w659 -> [w1380]
      tunnel: w658 -> [w1379]
      tunnel: [w1378] -> w657
      tunnel: w656 -> [w1378]
      tunnel: [w1557] -> w1037
      tunnel: [w1619] -> w1035
      tunnel: [w1559] -> w1033
      tunnel: [w1618] -> w1031
      tunnel: [w1617] -> w1029
      tunnel: [w1616] -> w1027
      tunnel: [w1615] -> w1025
      tunnel: [w1614] -> w1023
      tunnel: [w1613] -> w1021
      tunnel: [w1607] -> w1019
      tunnel: [w1602] -> w1017
      tunnel: [w1590] -> w1015
      tunnel: [w1589] -> w1013
      tunnel: [w1583] -> w1011
      tunnel: [w1555] -> w1009
      tunnel: [w1554] -> w993
      tunnel: [w1562] -> w990
      tunnel: [w1550] -> w981
      tunnel: [w1549] -> w971
      tunnel: [w1548] -> w958
      tunnel: [w1547] -> w951
      tunnel: w777 -> [w1547]
      tunnel: w778 -> [w1548]
      tunnel: w779 -> [w1549]
      tunnel: w780 -> [w1550]
      tunnel: w781 -> [w1553]
      tunnel: w782 -> [w1585]
      tunnel: w783 -> [w1592]
      tunnel: w784 -> [w1591]
      tunnel: w785 -> [w1604]
      tunnel: w786 -> [w1611]
      tunnel: w787 -> [w1613]
      tunnel: w788 -> [w1614]
      tunnel: w789 -> [w1615]
      tunnel: w790 -> [w1616]
      tunnel: w791 -> [w1617]
      tunnel: w792 -> [w1618]
      tunnel: w793 -> [w1619]
      tunnel: w794 -> [w1558]
      tunnel: w795 -> [w1561]
      tunnel: w796 -> [w1559]
      tunnel: [w1503] -> w730
      tunnel: w729 -> [w1503]
      tunnel: [w1502] -> w703
      tunnel: w702 -> [w1502]
      tunnel: w657 -> [w1486]
      tunnel: [w1485] -> w655
      tunnel: w1037 -> [w1635]
      tunnel: [w1634] -> w1036
      tunnel: w1035 -> [w1655]
      tunnel: [w1655] -> w1034
      tunnel: w1033 -> [w1654]
      tunnel: [w1654] -> w1032
      tunnel: w1031 -> [w1653]
      tunnel: [w1653] -> w1030
      tunnel: w1029 -> [w1652]
      tunnel: [w1652] -> w1028
      tunnel: w1027 -> [w1651]
      tunnel: [w1651] -> w1026
      tunnel: w1025 -> [w1650]
      tunnel: [w1650] -> w1024
      tunnel: w1023 -> [w1649]
      tunnel: [w1649] -> w1022
      tunnel: w1021 -> [w1648]
      tunnel: [w1648] -> w1020
      tunnel: w1019 -> [w1647]
      tunnel: [w1647] -> w1018
      tunnel: w1017 -> [w1646]
      tunnel: [w1646] -> w1016
      tunnel: w1015 -> [w1645]
      tunnel: [w1645] -> w1014
      tunnel: w1013 -> [w1644]
      tunnel: [w1644] -> w1012
      tunnel: w1011 -> [w1643]
      tunnel: [w1643] -> w1010
      tunnel: w1009 -> [w1628]
      tunnel: w993 -> [w1641]
      tunnel: [w1641] -> w992
      tunnel: w990 -> [w1620]
      tunnel: [w1639] -> w982
      tunnel: w981 -> [w1639]
      tunnel: [w1638] -> w972
      tunnel: w971 -> [w1638]
      tunnel: [w1637] -> w959
      tunnel: w958 -> [w1637]
      tunnel: [w1636] -> w952
      tunnel: w951 -> [w1636]
      tunnel: [w1633] -> w904
      tunnel: [w1623] -> w731
      tunnel: w730 -> [w1623]
      tunnel: [w1622] -> w704
      tunnel: w703 -> [w1622]
      tunnel: w655 -> [w1621]
      tunnel: [w1621] -> w654
      tunnel: w1036 -> [w1709]
      tunnel: [w1709] -> w1008
      tunnel: w1034 -> [w1708]
      tunnel: [w1708] -> w1007
      tunnel: w1032 -> [w1707]
      tunnel: [w1707] -> w1006
      tunnel: w1030 -> [w1706]
      tunnel: [w1706] -> w1005
      tunnel: w1028 -> [w1705]
      tunnel: [w1705] -> w1004
      tunnel: w1026 -> [w1704]
      tunnel: [w1704] -> w1003
      tunnel: w1024 -> [w1703]
      tunnel: [w1702] -> w1002
      tunnel: w1022 -> [w1701]
      tunnel: [w1700] -> w1001
      tunnel: w1020 -> [w1699]
      tunnel: [w1698] -> w1000
      tunnel: [w1686] -> w999
      tunnel: [w1685] -> w998
      tunnel: w1018 -> [w1685]
      tunnel: w1016 -> [w1684]
      tunnel: [w1684] -> w997
      tunnel: [w1683] -> w996
      tunnel: w1014 -> [w1683]
      tunnel: w1012 -> [w1682]
      tunnel: [w1682] -> w995
      tunnel: [w1681] -> w994
      tunnel: w1010 -> [w1681]
      tunnel: w992 -> [w1680]
      tunnel: [w1679] -> w991
      tunnel: [w1678] -> w983
      tunnel: w982 -> [w1678]
      tunnel: [w1677] -> w973
      tunnel: w972 -> [w1677]
      tunnel: [w1676] -> w960
      tunnel: w959 -> [w1676]
      tunnel: [w1675] -> w953
      tunnel: w952 -> [w1675]
      tunnel: w904 -> [w1674]
      tunnel: [w1672] -> w806
      tunnel: [w1670] -> w801
      tunnel: [w1669] -> w732
      tunnel: w731 -> [w1669]
      tunnel: [w1668] -> w705
      tunnel: w704 -> [w1668]
      tunnel: w654 -> [w1667]
      tunnel: [w1667] -> w653
      tunnel: [w1813] -> w1154
      tunnel: [w1812] -> w1152
      tunnel: [w1811] -> w1150
      tunnel: [w1810] -> w1148
      tunnel: [w1809] -> w1146
      tunnel: [w1808] -> w1144
      tunnel: [w1799] -> w1142
      tunnel: [w1807] -> w1140
      tunnel: [w1806] -> w1138
      tunnel: [w1805] -> w1136
      tunnel: [w1804] -> w1134
      tunnel: [w1803] -> w1132
      tunnel: [w1802] -> w1130
      tunnel: [w1801] -> w1128
      tunnel: [w1800] -> w1126
      tunnel: w994 -> [w1800]
      tunnel: w995 -> [w1801]
      tunnel: w996 -> [w1802]
      tunnel: w997 -> [w1803]
      tunnel: w998 -> [w1804]
      tunnel: w999 -> [w1805]
      tunnel: w1000 -> [w1806]
      tunnel: w1001 -> [w1807]
      tunnel: w1002 -> [w1799]
      tunnel: w1003 -> [w1808]
      tunnel: w1004 -> [w1809]
      tunnel: w1005 -> [w1810]
      tunnel: w1006 -> [w1811]
      tunnel: w1007 -> [w1812]
      tunnel: w1008 -> [w1813]
      tunnel: w991 -> [w1791]
      tunnel: [w1788] -> w984
      tunnel: w983 -> [w1788]
      tunnel: [w1787] -> w974
      tunnel: w973 -> [w1787]
      tunnel: [w1786] -> w961
      tunnel: w960 -> [w1786]
      tunnel: [w1785] -> w954
      tunnel: w953 -> [w1785]
      tunnel: w806 -> [w1784]
      tunnel: w801 -> [w1783]
      tunnel: [w1781] -> w800
      tunnel: [w1779] -> w733
      tunnel: w732 -> [w1779]
      tunnel: [w1778] -> w706
      tunnel: w705 -> [w1778]
      tunnel: w653 -> [w1777]
      tunnel: [w1777] -> w627
      tunnel: w1154 -> [w1921]
      tunnel: [w1921] -> w1153
      tunnel: w1152 -> [w1920]
      tunnel: [w1920] -> w1151
      tunnel: w1150 -> [w1919]
      tunnel: [w1919] -> w1149
      tunnel: w1148 -> [w1918]
      tunnel: [w1918] -> w1147
      tunnel: w1146 -> [w1917]
      tunnel: [w1917] -> w1145
      tunnel: w1144 -> [w1916]
      tunnel: [w1916] -> w1143
      tunnel: w1142 -> [w1915]
      tunnel: [w1915] -> w1141
      tunnel: w1140 -> [w1914]
      tunnel: [w1914] -> w1139
      tunnel: w1138 -> [w1913]
      tunnel: [w1913] -> w1137
      tunnel: w1136 -> [w1912]
      tunnel: [w1912] -> w1135
      tunnel: w1134 -> [w1911]
      tunnel: [w1911] -> w1133
      tunnel: w1132 -> [w1910]
      tunnel: [w1910] -> w1131
      tunnel: w1130 -> [w1909]
      tunnel: [w1909] -> w1129
      tunnel: w1128 -> [w1908]
      tunnel: [w1908] -> w1127
      tunnel: w1126 -> [w1907]
      tunnel: [w1907] -> w1125
      tunnel: [w1905] -> w985
      tunnel: w984 -> [w1905]
      tunnel: [w1904] -> w975
      tunnel: w974 -> [w1904]
      tunnel: [w1903] -> w962
      tunnel: w961 -> [w1903]
      tunnel: [w1902] -> w955
      tunnel: w954 -> [w1902]
      tunnel: w800 -> [w1899]
      tunnel: [w1897] -> w734
      tunnel: w733 -> [w1897]
      tunnel: [w1896] -> w707
      tunnel: w706 -> [w1896]
      tunnel: [w1895] -> w628
      tunnel: w627 -> [w1895]
      tunnel: w1153 -> [w2022]
      tunnel: w1151 -> [w2012]
      tunnel: w1149 -> [w2016]
      tunnel: [w2021] -> w941
      tunnel: w1147 -> [w2020]
      tunnel: [w2020] -> w940
      tunnel: [w2016] -> w938
      tunnel: w1145 -> [w2019]
      tunnel: [w2019] -> w936
      tunnel: w1143 -> [w2018]
      tunnel: [w2018] -> w934
      tunnel: [w2017] -> w932
      tunnel: w1141 -> [w2017]
      tunnel: [w2015] -> w930
      tunnel: [w2014] -> w928
      tunnel: w1139 -> [w2014]
      tunnel: [w2013] -> w926
      tunnel: w1137 -> [w2013]
      tunnel: [w1996] -> w924
      tunnel: w1135 -> [w2011]
      tunnel: [w2011] -> w923
      tunnel: [w2010] -> w921
      tunnel: w1133 -> [w2010]
      tunnel: [w2009] -> w919
      tunnel: w1131 -> [w2009]
      tunnel: w1129 -> [w2008]
      tunnel: [w2008] -> w917
      tunnel: [w2007] -> w915
      tunnel: w1127 -> [w2007]
      tunnel: w1125 -> [w2006]
      tunnel: [w2006] -> w913
      tunnel: w985 -> [w2005]
      tunnel: [w2003] -> w911
      tunnel: w975 -> [w2003]
      tunnel: [w2002] -> w909
      tunnel: w962 -> [w2002]
      tunnel: w955 -> [w2001]
      tunnel: [w2001] -> w907
      tunnel: [w2000] -> w901
      tunnel: [w1989] -> w735
      tunnel: w734 -> [w1989]
      tunnel: [w1988] -> w708
      tunnel: w707 -> [w1988]
      tunnel: [w1987] -> w629
      tunnel: w628 -> [w1987]
      tunnel: w941 -> [w2042]
      tunnel: w940 -> [w2059]
      tunnel: [w2059] -> w939
      tunnel: w938 -> [w2058]
      tunnel: [w2058] -> w937
      tunnel: w936 -> [w2057]
      tunnel: [w2057] -> w935
      tunnel: w934 -> [w2056]
      tunnel: [w2056] -> w933
      tunnel: w932 -> [w2055]
      tunnel: [w2055] -> w931
      tunnel: w930 -> [w2034]
      tunnel: [w2040] -> w929
      tunnel: w928 -> [w2054]
      tunnel: [w2054] -> w927
      tunnel: w926 -> [w2053]
      tunnel: [w2053] -> w925
      tunnel: w924 -> [w2025]
      tunnel: w923 -> [w2052]
      tunnel: [w2052] -> w922
      tunnel: w921 -> [w2051]
      tunnel: [w2051] -> w920
      tunnel: w919 -> [w2050]
      tunnel: [w2050] -> w918
      tunnel: w917 -> [w2049]
      tunnel: [w2049] -> w916
      tunnel: w915 -> [w2048]
      tunnel: [w2048] -> w914
      tunnel: w913 -> [w2047]
      tunnel: [w2047] -> w912
      tunnel: w911 -> [w2046]
      tunnel: [w2046] -> w910
      tunnel: w909 -> [w2045]
      tunnel: [w2045] -> w908
      tunnel: w907 -> [w2044]
      tunnel: [w2044] -> w906
      tunnel: [w2041] -> w905
      tunnel: [w2039] -> w902
      tunnel: w901 -> [w2039]
      tunnel: [w2028] -> w736
      tunnel: w735 -> [w2028]
      tunnel: [w2027] -> w709
      tunnel: w708 -> [w2027]
      tunnel: [w2026] -> w630
      tunnel: w629 -> [w2026]
      tunnel: [w2097] -> w1203
      tunnel: w939 -> [w2096]
      tunnel: [w2096] -> w1202
      tunnel: w937 -> [w2095]
      tunnel: [w2095] -> w1201
      tunnel: w935 -> [w2094]
      tunnel: [w2094] -> w1200
      tunnel: w933 -> [w2093]
      tunnel: [w2093] -> w1199
      tunnel: w931 -> [w2091]
      tunnel: [w2090] -> w1198
      tunnel: w929 -> [w2092]
      tunnel: w927 -> [w2089]
      tunnel: [w2088] -> w1197
      tunnel: [w2086] -> w1196
      tunnel: w925 -> [w2087]
      tunnel: [w2085] -> w1195
      tunnel: w922 -> [w2085]
      tunnel: [w2084] -> w1194
      tunnel: w920 -> [w2084]
      tunnel: [w2083] -> w1193
      tunnel: w918 -> [w2083]
      tunnel: [w2082] -> w1192
      tunnel: w916 -> [w2082]
      tunnel: w914 -> [w2081]
      tunnel: [w2081] -> w1191
      tunnel: [w2080] -> w1190
      tunnel: w912 -> [w2080]
      tunnel: [w2079] -> w976
      tunnel: w910 -> [w2079]
      tunnel: [w2078] -> w963
      tunnel: w908 -> [w2078]
      tunnel: [w2077] -> w942
      tunnel: w906 -> [w2077]
      tunnel: w905 -> [w2097]
      tunnel: [w2076] -> w903
      tunnel: w902 -> [w2075]
      tunnel: [w2074] -> w805
      tunnel: [w2073] -> w737
      tunnel: w736 -> [w2073]
      tunnel: [w2072] -> w710
      tunnel: w709 -> [w2072]
      tunnel: [w2071] -> w631
      tunnel: w630 -> [w2071]
      tunnel: w1203 -> [w2198]
      tunnel: [w2198] -> w1124
      tunnel: w1202 -> [w2197]
      tunnel: [w2197] -> w1122
      tunnel: w1201 -> [w2196]
      tunnel: [w2196] -> w1120
      tunnel: w1200 -> [w2195]
      tunnel: [w2195] -> w1118
      tunnel: w1199 -> [w2194]
      tunnel: [w2194] -> w1116
      tunnel: w1198 -> [w2171]
      tunnel: [w2171] -> w1114
      tunnel: w1197 -> [w2193]
      tunnel: [w2193] -> w1112
      tunnel: w1196 -> [w2192]
      tunnel: [w2192] -> w1110
      tunnel: w1195 -> [w2191]
      tunnel: [w2191] -> w1108
      tunnel: w1194 -> [w2190]
      tunnel: [w2190] -> w1106
      tunnel: w1193 -> [w2189]
      tunnel: [w2189] -> w1104
      tunnel: [w2188] -> w1102
      tunnel: w1192 -> [w2188]
      tunnel: [w2187] -> w1100
      tunnel: w1191 -> [w2187]
      tunnel: [w2186] -> w1098
      tunnel: w1190 -> [w2186]
      tunnel: [w2185] -> w977
      tunnel: w976 -> [w2185]
      tunnel: [w2184] -> w964
      tunnel: w963 -> [w2184]
      tunnel: [w2183] -> w943
      tunnel: w942 -> [w2183]
      tunnel: w903 -> [w2182]
      tunnel: w805 -> [w2170]
      tunnel: [w2169] -> w799
      tunnel: [w2167] -> w738
      tunnel: w737 -> [w2167]
      tunnel: [w2166] -> w711
      tunnel: w710 -> [w2166]
      tunnel: [w2165] -> w632
      tunnel: w631 -> [w2165]
      tunnel: w1124 -> [w2303]
      tunnel: [w2303] -> w1123
      tunnel: w1122 -> [w2302]
      tunnel: [w2302] -> w1121
      tunnel: w1120 -> [w2301]
      tunnel: [w2301] -> w1119
      tunnel: w1118 -> [w2300]
      tunnel: [w2300] -> w1117
      tunnel: w1116 -> [w2299]
      tunnel: [w2299] -> w1115
      tunnel: w1114 -> [w2298]
      tunnel: [w2298] -> w1113
      tunnel: w1112 -> [w2297]
      tunnel: [w2297] -> w1111
      tunnel: w1110 -> [w2296]
      tunnel: [w2296] -> w1109
      tunnel: w1108 -> [w2295]
      tunnel: [w2295] -> w1107
      tunnel: w1106 -> [w2294]
      tunnel: [w2294] -> w1105
      tunnel: w1104 -> [w2293]
      tunnel: [w2293] -> w1103
      tunnel: w1102 -> [w2292]
      tunnel: [w2292] -> w1101
      tunnel: w1100 -> [w2291]
      tunnel: [w2291] -> w1099
      tunnel: w1098 -> [w2290]
      tunnel: [w2290] -> w1097
      tunnel: [w2288] -> w978
      tunnel: w977 -> [w2288]
      tunnel: [w2287] -> w965
      tunnel: w964 -> [w2287]
      tunnel: [w2286] -> w944
      tunnel: w943 -> [w2286]
      tunnel: w799 -> [w2284]
      tunnel: [w2281] -> w739
      tunnel: w738 -> [w2281]
      tunnel: [w2280] -> w712
      tunnel: w711 -> [w2280]
      tunnel: [w2279] -> w633
      tunnel: w632 -> [w2279]
      tunnel: w1123 -> [w2402]
      tunnel: w1121 -> [w2393]
      tunnel: w1119 -> [w2400]
      tunnel: [w2401] -> w900
      tunnel: [w2400] -> w898
      tunnel: [w2399] -> w896
      tunnel: w1117 -> [w2399]
      tunnel: [w2398] -> w894
      tunnel: w1115 -> [w2398]
      tunnel: [w2397] -> w892
      tunnel: w1113 -> [w2397]
      tunnel: [w2396] -> w890
      tunnel: [w2395] -> w888
      tunnel: w1111 -> [w2395]
      tunnel: [w2394] -> w886
      tunnel: w1109 -> [w2394]
      tunnel: [w2376] -> w884
      tunnel: [w2392] -> w883
      tunnel: w1107 -> [w2392]
      tunnel: [w2391] -> w881
      tunnel: w1105 -> [w2391]
      tunnel: [w2390] -> w879
      tunnel: w1103 -> [w2390]
      tunnel: w1101 -> [w2389]
      tunnel: [w2389] -> w877
      tunnel: w1099 -> [w2388]
      tunnel: [w2388] -> w875
      tunnel: w1097 -> [w2387]
      tunnel: [w2387] -> w873
      tunnel: w978 -> [w2386]
      tunnel: [w2382] -> w871
      tunnel: w965 -> [w2382]
      tunnel: [w2381] -> w869
      tunnel: w944 -> [w2381]
      tunnel: [w2380] -> w865
      tunnel: [w2371] -> w740
      tunnel: w739 -> [w2371]
      tunnel: [w2370] -> w713
      tunnel: w712 -> [w2370]
      tunnel: [w2369] -> w634
      tunnel: w633 -> [w2369]
      tunnel: w900 -> [w2421]
      tunnel: [w2422] -> w899
      tunnel: w898 -> [w2439]
      tunnel: [w2439] -> w897
      tunnel: w896 -> [w2438]
      tunnel: [w2438] -> w895
      tunnel: w894 -> [w2437]
      tunnel: [w2437] -> w893
      tunnel: w892 -> [w2436]
      tunnel: [w2436] -> w891
      tunnel: w890 -> [w2412]
      tunnel: [w2420] -> w889
      tunnel: w888 -> [w2435]
      tunnel: [w2435] -> w887
      tunnel: w886 -> [w2434]
      tunnel: [w2434] -> w885
      tunnel: w884 -> [w2415]
      tunnel: w883 -> [w2433]
      tunnel: [w2433] -> w882
      tunnel: w881 -> [w2432]
      tunnel: [w2432] -> w880
      tunnel: w879 -> [w2431]
      tunnel: [w2431] -> w878
      tunnel: w877 -> [w2430]
      tunnel: [w2430] -> w876
      tunnel: w875 -> [w2429]
      tunnel: [w2429] -> w874
      tunnel: w873 -> [w2428]
      tunnel: [w2428] -> w872
      tunnel: w871 -> [w2427]
      tunnel: [w2427] -> w870
      tunnel: w869 -> [w2426]
      tunnel: [w2426] -> w868
      tunnel: [w2419] -> w866
      tunnel: w865 -> [w2419]
      tunnel: [w2407] -> w741
      tunnel: w740 -> [w2407]
      tunnel: [w2406] -> w714
      tunnel: w713 -> [w2406]
      tunnel: [w2405] -> w635
      tunnel: w634 -> [w2405]
      tunnel: w899 -> [w2475]
      tunnel: [w2475] -> w1189
      tunnel: w897 -> [w2474]
      tunnel: [w2474] -> w1188
      tunnel: w895 -> [w2473]
      tunnel: [w2473] -> w1187
      tunnel: w893 -> [w2472]
      tunnel: [w2472] -> w1186
      tunnel: w891 -> [w2470]
      tunnel: [w2469] -> w1185
      tunnel: w889 -> [w2471]
      tunnel: w887 -> [w2468]
      tunnel: [w2467] -> w1184
      tunnel: [w2465] -> w1183
      tunnel: w885 -> [w2466]
      tunnel: [w2464] -> w1182
      tunnel: w882 -> [w2464]
      tunnel: [w2463] -> w1181
      tunnel: w880 -> [w2463]
      tunnel: w878 -> [w2462]
      tunnel: [w2462] -> w1180
      tunnel: w876 -> [w2461]
      tunnel: [w2461] -> w1179
      tunnel: [w2460] -> w1178
      tunnel: w874 -> [w2460]
      tunnel: [w2459] -> w1177
      tunnel: w872 -> [w2459]
      tunnel: [w2458] -> w966
      tunnel: w870 -> [w2458]
      tunnel: [w2457] -> w945
      tunnel: w868 -> [w2457]
      tunnel: [w2456] -> w867
      tunnel: w866 -> [w2455]
      tunnel: [w2454] -> w804
      tunnel: [w2453] -> w742
      tunnel: w741 -> [w2453]
      tunnel: [w2452] -> w715
      tunnel: w714 -> [w2452]
      tunnel: [w2451] -> w636
      tunnel: w635 -> [w2451]
      tunnel: w1189 -> [w2573]
      tunnel: [w2573] -> w1096
      tunnel: w1188 -> [w2572]
      tunnel: [w2572] -> w1094
      tunnel: w1187 -> [w2571]
      tunnel: [w2571] -> w1092
      tunnel: w1186 -> [w2570]
      tunnel: [w2570] -> w1090
      tunnel: w1185 -> [w2548]
      tunnel: [w2548] -> w1088
      tunnel: w1184 -> [w2569]
      tunnel: [w2569] -> w1086
      tunnel: w1183 -> [w2568]
      tunnel: [w2568] -> w1084
      tunnel: w1182 -> [w2567]
      tunnel: [w2567] -> w1082
      tunnel: [w2566] -> w1080
      tunnel: w1181 -> [w2566]
      tunnel: [w2565] -> w1078
      tunnel: w1180 -> [w2565]
      tunnel: [w2564] -> w1076
      tunnel: w1179 -> [w2564]
      tunnel: w1178 -> [w2563]
      tunnel: [w2563] -> w1074
      tunnel: [w2562] -> w1072
      tunnel: w1177 -> [w2562]
      tunnel: [w2561] -> w967
      tunnel: w966 -> [w2561]
      tunnel: [w2560] -> w946
      tunnel: w945 -> [w2560]
      tunnel: w867 -> [w2559]
      tunnel: w804 -> [w2547]
      tunnel: [w2546] -> w776
      tunnel: [w2545] -> w743
      tunnel: w742 -> [w2545]
      tunnel: [w2544] -> w716
      tunnel: w715 -> [w2544]
      tunnel: [w2543] -> w637
      tunnel: w636 -> [w2543]
      tunnel: w1096 -> [w2677]
      tunnel: [w2677] -> w1095
      tunnel: w1094 -> [w2676]
      tunnel: [w2676] -> w1093
      tunnel: w1092 -> [w2675]
      tunnel: [w2675] -> w1091
      tunnel: w1090 -> [w2674]
      tunnel: [w2674] -> w1089
      tunnel: w1088 -> [w2673]
      tunnel: [w2673] -> w1087
      tunnel: w1086 -> [w2672]
      tunnel: [w2672] -> w1085
      tunnel: w1084 -> [w2671]
      tunnel: [w2671] -> w1083
      tunnel: w1082 -> [w2670]
      tunnel: [w2670] -> w1081
      tunnel: w1080 -> [w2669]
      tunnel: [w2669] -> w1079
      tunnel: w1078 -> [w2668]
      tunnel: [w2668] -> w1077
      tunnel: w1076 -> [w2667]
      tunnel: [w2667] -> w1075
      tunnel: w1074 -> [w2666]
      tunnel: [w2666] -> w1073
      tunnel: w1072 -> [w2665]
      tunnel: [w2665] -> w1071
      tunnel: [w2662] -> w968
      tunnel: w967 -> [w2662]
      tunnel: [w2661] -> w947
      tunnel: w946 -> [w2661]
      tunnel: w776 -> [w2658]
      tunnel: [w2657] -> w775
      tunnel: [w2656] -> w744
      tunnel: w743 -> [w2656]
      tunnel: [w2655] -> w717
      tunnel: w716 -> [w2655]
      tunnel: [w2654] -> w638
      tunnel: w637 -> [w2654]
      tunnel: w1095 -> [w2775]
      tunnel: [w2774] -> w864
      tunnel: w1093 -> [w2772]
      tunnel: w1091 -> [w2767]
      tunnel: [w2773] -> w862
      tunnel: w1089 -> [w2773]
      tunnel: [w2772] -> w860
      tunnel: [w2771] -> w858
      tunnel: w1087 -> [w2771]
      tunnel: [w2770] -> w856
      tunnel: [w2769] -> w854
      tunnel: w1085 -> [w2769]
      tunnel: [w2768] -> w852
      tunnel: w1083 -> [w2768]
      tunnel: [w2751] -> w850
      tunnel: w1081 -> [w2766]
      tunnel: [w2766] -> w849
      tunnel: [w2765] -> w847
      tunnel: w1079 -> [w2765]
      tunnel: w1077 -> [w2764]
      tunnel: [w2764] -> w845
      tunnel: w1075 -> [w2763]
      tunnel: [w2763] -> w843
      tunnel: w1073 -> [w2762]
      tunnel: [w2762] -> w841
      tunnel: w1071 -> [w2761]
      tunnel: [w2761] -> w839
      tunnel: w968 -> [w2760]
      tunnel: [w2756] -> w837
      tunnel: w947 -> [w2756]
      tunnel: [w2755] -> w833
      tunnel: w775 -> [w2746]
      tunnel: [w2745] -> w745
      tunnel: w744 -> [w2745]
      tunnel: [w2744] -> w718
      tunnel: w717 -> [w2744]
      tunnel: [w2743] -> w639
      tunnel: w638 -> [w2743]
      tunnel: w864 -> [w2792]
      tunnel: [w2794] -> w863
      tunnel: w862 -> [w2808]
      tunnel: [w2808] -> w861
      tunnel: w860 -> [w2807]
      tunnel: [w2807] -> w859
      tunnel: w858 -> [w2806]
      tunnel: [w2806] -> w857
      tunnel: w856 -> [w2786]
      tunnel: [w2793] -> w855
      tunnel: w854 -> [w2805]
      tunnel: [w2805] -> w853
      tunnel: w852 -> [w2804]
      tunnel: [w2804] -> w851
      tunnel: w850 -> [w2778]
      tunnel: w849 -> [w2803]
      tunnel: [w2803] -> w848
      tunnel: w847 -> [w2802]
      tunnel: [w2802] -> w846
      tunnel: w845 -> [w2801]
      tunnel: [w2801] -> w844
      tunnel: w843 -> [w2800]
      tunnel: [w2800] -> w842
      tunnel: w841 -> [w2799]
      tunnel: [w2799] -> w840
      tunnel: w839 -> [w2798]
      tunnel: [w2798] -> w838
      tunnel: w837 -> [w2797]
      tunnel: [w2797] -> w836
      tunnel: [w2791] -> w834
      tunnel: w833 -> [w2791]
      tunnel: [w2781] -> w746
      tunnel: w745 -> [w2781]
      tunnel: [w2780] -> w719
      tunnel: w718 -> [w2780]
      tunnel: [w2779] -> w640
      tunnel: w639 -> [w2779]
      tunnel: w863 -> [w2842]
      tunnel: [w2842] -> w1176
      tunnel: w861 -> [w2841]
      tunnel: [w2841] -> w1175
      tunnel: w859 -> [w2840]
      tunnel: [w2840] -> w1174
      tunnel: w857 -> [w2838]
      tunnel: [w2837] -> w1173
      tunnel: w855 -> [w2839]
      tunnel: w853 -> [w2836]
      tunnel: [w2835] -> w1172
      tunnel: [w2833] -> w1171
      tunnel: w851 -> [w2834]
      tunnel: w848 -> [w2832]
      tunnel: [w2832] -> w1170
      tunnel: [w2831] -> w1169
      tunnel: w846 -> [w2831]
      tunnel: [w2830] -> w1168
      tunnel: w844 -> [w2830]
      tunnel: [w2829] -> w1167
      tunnel: w842 -> [w2829]
      tunnel: w840 -> [w2828]
      tunnel: [w2828] -> w1166
      tunnel: [w2827] -> w1165
      tunnel: w838 -> [w2827]
      tunnel: [w2826] -> w948
      tunnel: w836 -> [w2826]
      tunnel: [w2825] -> w835
      tunnel: w834 -> [w2824]
      tunnel: [w2823] -> w803
      tunnel: [w2822] -> w747
      tunnel: w746 -> [w2822]
      tunnel: [w2821] -> w720
      tunnel: w719 -> [w2821]
      tunnel: [w2820] -> w641
      tunnel: w640 -> [w2820]
      tunnel: w1176 -> [w2939]
      tunnel: [w2939] -> w1070
      tunnel: w1175 -> [w2938]
      tunnel: [w2938] -> w1068
      tunnel: w1174 -> [w2937]
      tunnel: [w2937] -> w1066
      tunnel: w1173 -> [w2916]
      tunnel: [w2916] -> w1064
      tunnel: w1172 -> [w2936]
      tunnel: [w2936] -> w1062
      tunnel: w1171 -> [w2935]
      tunnel: [w2935] -> w1060
      tunnel: w1170 -> [w2934]
      tunnel: [w2934] -> w1058
      tunnel: [w2933] -> w1056
      tunnel: w1169 -> [w2933]
      tunnel: [w2932] -> w1054
      tunnel: w1168 -> [w2932]
      tunnel: [w2931] -> w1052
      tunnel: w1167 -> [w2931]
      tunnel: [w2930] -> w1050
      tunnel: w1166 -> [w2930]
      tunnel: w1165 -> [w2929]
      tunnel: [w2929] -> w1048
      tunnel: [w2928] -> w949
      tunnel: w948 -> [w2928]
      tunnel: w835 -> [w2927]
      tunnel: w803 -> [w2915]
      tunnel: [w2914] -> w798
      tunnel: [w2912] -> w748
      tunnel: w747 -> [w2912]
      tunnel: [w2911] -> w721
      tunnel: w720 -> [w2911]
      tunnel: [w2910] -> w642
      tunnel: w641 -> [w2910]
      tunnel: w1070 -> [w3040]
      tunnel: [w3040] -> w1069
      tunnel: w1068 -> [w3039]
      tunnel: [w3039] -> w1067
      tunnel: w1066 -> [w3038]
      tunnel: [w3038] -> w1065
      tunnel: w1064 -> [w3037]
      tunnel: [w3037] -> w1063
      tunnel: w1062 -> [w3036]
      tunnel: [w3036] -> w1061
      tunnel: w1060 -> [w3035]
      tunnel: [w3035] -> w1059
      tunnel: w1058 -> [w3034]
      tunnel: [w3034] -> w1057
      tunnel: w1056 -> [w3033]
      tunnel: [w3033] -> w1055
      tunnel: w1054 -> [w3032]
      tunnel: [w3032] -> w1053
      tunnel: w1052 -> [w3031]
      tunnel: [w3031] -> w1051
      tunnel: w1050 -> [w3030]
      tunnel: [w3030] -> w1049
      tunnel: w1048 -> [w3029]
      tunnel: [w3029] -> w1047
      tunnel: [w3027] -> w950
      tunnel: w949 -> [w3027]
      tunnel: w798 -> [w3024]
      tunnel: [w3022] -> w749
      tunnel: w748 -> [w3022]
      tunnel: [w3021] -> w722
      tunnel: w721 -> [w3021]
      tunnel: [w3020] -> w643
      tunnel: w642 -> [w3020]
      tunnel: w1069 -> [w3135]
      tunnel: w1067 -> [w3129]
      tunnel: w1065 -> [w3107]
      tunnel: w1063 -> [w3133]
      tunnel: [w3134] -> w832
      tunnel: [w3133] -> w830
      tunnel: [w3132] -> w828
      tunnel: [w3131] -> w827
      tunnel: w1061 -> [w3131]
      tunnel: [w3130] -> w825
      tunnel: w1059 -> [w3130]
      tunnel: [w3115] -> w823
      tunnel: [w3128] -> w822
      tunnel: w1057 -> [w3128]
      tunnel: w1055 -> [w3127]
      tunnel: [w3127] -> w820
      tunnel: w1053 -> [w3126]
      tunnel: [w3126] -> w818
      tunnel: w1051 -> [w3125]
      tunnel: [w3125] -> w816
      tunnel: w1049 -> [w3124]
      tunnel: [w3124] -> w814
      tunnel: [w3123] -> w812
      tunnel: w1047 -> [w3123]
      tunnel: w950 -> [w3122]
      tunnel: [w3118] -> w807
      tunnel: [w3109] -> w750
      tunnel: w749 -> [w3109]
      tunnel: [w3108] -> w723
      tunnel: w722 -> [w3108]
      tunnel: [w3107] -> w700
      tunnel: [w3106] -> w644
      tunnel: w643 -> [w3106]
      tunnel: w832 -> [w3155]
      tunnel: [w3154] -> w831
      tunnel: w830 -> [w3166]
      tunnel: [w3166] -> w829
      tunnel: w828 -> [w3147]
      tunnel: w827 -> [w3165]
      tunnel: [w3165] -> w826
      tunnel: w825 -> [w3164]
      tunnel: [w3164] -> w824
      tunnel: w823 -> [w3138]
      tunnel: w822 -> [w3163]
      tunnel: [w3163] -> w821
      tunnel: w820 -> [w3162]
      tunnel: [w3162] -> w819
      tunnel: w818 -> [w3161]
      tunnel: [w3161] -> w817
      tunnel: w816 -> [w3160]
      tunnel: [w3160] -> w815
      tunnel: w814 -> [w3159]
      tunnel: [w3159] -> w813
      tunnel: w812 -> [w3158]
      tunnel: [w3158] -> w811
      tunnel: [w3153] -> w810
      tunnel: [w3152] -> w808
      tunnel: w807 -> [w3152]
      tunnel: [w3142] -> w751
      tunnel: w750 -> [w3142]
      tunnel: [w3141] -> w724
      tunnel: w723 -> [w3141]
      tunnel: w700 -> [w3140]
      tunnel: [w3140] -> w696
      tunnel: [w3139] -> w645
      tunnel: w644 -> [w3139]
      tunnel: w831 -> [w3198]
      tunnel: w829 -> [w3196]
      tunnel: w826 -> [w3194]
      tunnel: w824 -> [w3192]
      tunnel: [w3198] -> w1164
      tunnel: [w3195] -> w1163
      tunnel: [w3193] -> w1162
      tunnel: [w3191] -> w1161
      tunnel: w821 -> [w3190]
      tunnel: [w3190] -> w1160
      tunnel: [w3189] -> w1159
      tunnel: w819 -> [w3189]
      tunnel: [w3188] -> w1158
      tunnel: w817 -> [w3188]
      tunnel: [w3187] -> w1157
      tunnel: w815 -> [w3187]
      tunnel: [w3186] -> w1156
      tunnel: w813 -> [w3186]
      tunnel: w811 -> [w3185]
      tunnel: [w3185] -> w1155
      tunnel: w810 -> [w3197]
      tunnel: [w3184] -> w809
      tunnel: w808 -> [w3183]
      tunnel: [w3182] -> w802
      tunnel: [w3181] -> w752
      tunnel: w751 -> [w3181]
      tunnel: [w3180] -> w725
      tunnel: w724 -> [w3180]
      tunnel: [w3179] -> w697
      tunnel: w696 -> [w3179]
      tunnel: [w3178] -> w646
      tunnel: w645 -> [w3178]
      tunnel: w1164 -> [w3293]
      tunnel: w1163 -> [w3273]
      tunnel: w1162 -> [w3292]
      tunnel: w1161 -> [w3291]
      tunnel: w1160 -> [w3285]
      tunnel: w1159 -> [w3290]
      tunnel: w1158 -> [w3289]
      tunnel: w1157 -> [w3288]
      tunnel: w1156 -> [w3287]
      tunnel: w1155 -> [w3286]
      tunnel: [w3293] -> w1046
      tunnel: [w3273] -> w1045
      tunnel: [w3292] -> w1044
      tunnel: [w3291] -> w1043
      tunnel: [w3290] -> w1042
      tunnel: [w3289] -> w1041
      tunnel: [w3288] -> w1040
      tunnel: [w3287] -> w1039
      tunnel: [w3286] -> w1038
      tunnel: w809 -> [w3284]
      tunnel: w802 -> [w3272]
      tunnel: [w3271] -> w797
      tunnel: [w3269] -> w753
      tunnel: w752 -> [w3269]
      tunnel: [w3268] -> w726
      tunnel: w725 -> [w3268]
      tunnel: [w3267] -> w698
      tunnel: w697 -> [w3267]
      tunnel: [w3266] -> w647
      tunnel: w646 -> [w3266]
      tunnel: w1046 -> [w3391]
      tunnel: [w3391] -> w766
      tunnel: w1045 -> [w3390]
      tunnel: [w3390] -> w767
      tunnel: w1044 -> [w3389]
      tunnel: [w3389] -> w768
      tunnel: w1043 -> [w3388]
      tunnel: [w3388] -> w769
      tunnel: w1042 -> [w3387]
      tunnel: [w3387] -> w770
      tunnel: w1041 -> [w3386]
      tunnel: [w3386] -> w771
      tunnel: w1040 -> [w3385]
      tunnel: [w3385] -> w772
      tunnel: w1039 -> [w3384]
      tunnel: [w3384] -> w773
      tunnel: w1038 -> [w3383]
      tunnel: [w3383] -> w774
      tunnel: w797 -> [w3379]
      tunnel: [w3377] -> w754
      tunnel: w753 -> [w3377]
      tunnel: [w3376] -> w727
      tunnel: w726 -> [w3376]
      tunnel: [w3375] -> w699
      tunnel: w698 -> [w3375]
      tunnel: [w3374] -> w648
      tunnel: w647 -> [w3374]
      tunnel: w774 -> [w3483]
      tunnel: [w3483] -> w765
      tunnel: w773 -> [w3482]
      tunnel: [w3482] -> w764
      tunnel: w772 -> [w3481]
      tunnel: [w3481] -> w763
      tunnel: w771 -> [w3480]
      tunnel: [w3480] -> w762
      tunnel: w770 -> [w3479]
      tunnel: [w3479] -> w761
      tunnel: w769 -> [w3478]
      tunnel: [w3478] -> w760
      tunnel: w768 -> [w3477]
      tunnel: [w3477] -> w759
      tunnel: w767 -> [w3476]
      tunnel: [w3476] -> w758
      tunnel: w766 -> [w3475]
      tunnel: [w3475] -> w757
      tunnel: w754 -> [w3463]
      tunnel: w727 -> [w3462]
      tunnel: w699 -> [w3461]
      tunnel: [w3460] -> w695
      tunnel: [w3459] -> w694
      tunnel: [w3458] -> w684
      tunnel: [w3457] -> w681
      tunnel: [w3456] -> w649
      tunnel: w648 -> [w3456]
      tunnel: w765 -> [w3509]
      tunnel: [w3509] -> w693
      tunnel: w764 -> [w3508]
      tunnel: [w3508] -> w692
      tunnel: w763 -> [w3507]
      tunnel: [w3507] -> w691
      tunnel: w762 -> [w3506]
      tunnel: [w3506] -> w690
      tunnel: w761 -> [w3505]
      tunnel: [w3505] -> w689
      tunnel: w760 -> [w3504]
      tunnel: [w3504] -> w688
      tunnel: w759 -> [w3503]
      tunnel: [w3503] -> w687
      tunnel: w758 -> [w3502]
      tunnel: [w3502] -> w686
      tunnel: w757 -> [w3501]
      tunnel: [w3501] -> w685
      tunnel: w695 -> [w3489]
      tunnel: w694 -> [w3488]
      tunnel: w684 -> [w3487]
      tunnel: [w3486] -> w683
      tunnel: [w3485] -> w682
      tunnel: w681 -> [w3485]
      tunnel: [w3484] -> w650
      tunnel: w649 -> [w3484]
      tunnel: w693 -> [w3535]
      tunnel: [w3535] -> w680
      tunnel: w692 -> [w3534]
      tunnel: [w3534] -> w678
      tunnel: w691 -> [w3533]
      tunnel: [w3533] -> w676
      tunnel: w690 -> [w3532]
      tunnel: [w3532] -> w674
      tunnel: w689 -> [w3531]
      tunnel: [w3531] -> w672
      tunnel: w688 -> [w3529]
      tunnel: [w3528] -> w670
      tunnel: w687 -> [w3524]
      tunnel: [w3523] -> w668
      tunnel: w686 -> [w3527]
      tunnel: [w3526] -> w666
      tunnel: w685 -> [w3530]
      tunnel: [w3530] -> w664
      tunnel: w683 -> [w3525]
      tunnel: w682 -> [w3522]
      tunnel: [w3521] -> w651
      tunnel: w650 -> [w3521]
      tunnel: w680 -> [w3612]
      tunnel: [w3612] -> w679
      tunnel: w678 -> [w3611]
      tunnel: [w3611] -> w677
      tunnel: w676 -> [w3610]
      tunnel: [w3610] -> w675
      tunnel: w674 -> [w3609]
      tunnel: [w3609] -> w673
      tunnel: w672 -> [w3608]
      tunnel: [w3608] -> w671
      tunnel: w670 -> [w3607]
      tunnel: [w3607] -> w669
      tunnel: w668 -> [w3606]
      tunnel: [w3606] -> w667
      tunnel: w666 -> [w3605]
      tunnel: [w3605] -> w665
      tunnel: w664 -> [w3604]
      tunnel: [w3604] -> w663
      tunnel: [w3603] -> w652
      tunnel: w651 -> [w3603]
      tunnel: [w3742] -> w1240
      tunnel: [w3743] -> w1242
      tunnel: [w3744] -> w1243
      tunnel: [w3745] -> w1244
      tunnel: [w3746] -> w1248
      tunnel: [w3619] -> w1250
      tunnel: [w3747] -> w1252
      tunnel: [w3748] -> w1254
      tunnel: [w3749] -> w1262
      tunnel: w679 -> [w3742]
      tunnel: w677 -> [w3743]
      tunnel: w675 -> [w3744]
      tunnel: w673 -> [w3745]
      tunnel: w671 -> [w3746]
      tunnel: w669 -> [w3619]
      tunnel: w667 -> [w3747]
      tunnel: w665 -> [w3748]
      tunnel: w663 -> [w3749]
      tunnel: [w3613] -> w626
      tunnel: w652 -> [w3613]
      frame #0 {
        n451 = Index Array(array=w1292, index #1=0 ("index")) -> (element #1=w1294:T2, element #2=w1295:T2)  [unwired: 1 in]
        n452 = Index Array(array=w1304, index #1=0 ("index")) -> (element #1=w1327:T3, element #2=w1328:T3)  [unwired: 1 in]
        n453 = Index Array(array=w1306, index #1=0 ("index")) -> (element #1=w1350:T5, element #2=w1349:T5)  [unwired: 1 in]
        n454 = Index Array(array=w1305, index #1=0 ("index")) -> (element #1=w1315:T4, element #2=w1316:T4)  [unwired: 1 in]
        n455 = Index Array(array=w1353, index #1=0 ("index")) -> (element #1=w1367:T6, element #2=w1366:T6)  [unwired: 1 in]
        n456 = Index Array(array=w1265, index #1=0 ("index")) -> (element #1=w1279:T1, element #2=w1278:T1)  [unwired: 1 in]
        n457 = Unbundle By Name(w1294) -> ("disc 05"=w1296:bool, "auto/man 05"=w1297:bool, "projector 05"=w1298:bool, "cam 05"=w1299:bool)
        n458 = Unbundle By Name(w1295) -> ("cam 05"=w1300:bool, "projector 05"=w1301:bool, "auto/man 05"=w1302:bool, "disc 05"=w1303:bool)
        n459 = Unbundle By Name(w1327) -> ("disc 04"=w1329:bool, "auto/man 04"=w1330:bool, "projector 04"=w1331:bool, "cam 04"=w1332:bool)
        n460 = Unbundle By Name(w1328) -> ("cam 04"=w1333:bool, "projector 04"=w1334:bool, "auto/man 04"=w1335:bool, "disc 04"=w1336:bool)
        n461 = Unbundle By Name(w1315) -> ("disc 03"=w1317:bool, "auto/man 03"=w1319:bool, "projector 03"=w1321:bool, "cam 03"=w1323:bool)
        n462 = Unbundle By Name(w1316) -> ("cam 03"=w1324:bool, "projector 03"=w1322:bool, "auto/man 03"=w1320:bool, "disc 03"=w1318:bool)
        n463 = Unbundle By Name(w1350) -> ("disc 02"=w1348:bool, "auto/man 02"=w1347:bool, "projector 02"=w1346:bool, "cam 02"=w1345:bool)
        n464 = Unbundle By Name(w1349) -> ("cam 02"=w1344:bool, "projector 02"=w1343:bool, "auto/man 02"=w1342:bool, "disc 02"=w1341:bool)
        n465 = Unbundle By Name(w1367) -> ("disc 01"=w1365:bool, "auto/man 01"=w1363:bool, "projector 01"=w1361:bool, "cam 01"=w1359:bool)
        n466 = Unbundle By Name(w1366) -> ("cam 01"=w1358:bool, "projector 01"=w1360:bool, "auto/man 01"=w1362:bool, "disc 01"=w1364:bool)
        n467 = Unbundle By Name(w1279) -> ("disc 06"=w1277:bool, "auto/man 06"=w1276:bool, "projector 06"=w1275:bool, "cam 06"=w1274:bool)
        n468 = Unbundle By Name(w1278) -> ("cam 06"=w1273:bool, "projector 06"=w1272:bool, "auto/man 06"=w1271:bool, "disc 06"=w1270:bool)
        n469 = Not Equal?(x=w1323, y=w1324) -> (x != y?=w1314:bool)
        n470 = Not Equal?(x=w1359, y=w1358) -> (x != y?=w1354:bool)
        n471 = Not Equal?(x=w1299, y=w1300) -> (x != y?=w1291:bool)
        n472 = Not Equal?(x=w1332, y=w1333) -> (x != y?=w1310:bool)
        n473 = Not Equal?(x=w1345, y=w1344) -> (x != y?=w1337:bool)
        n474 = Not Equal?(x=w1274, y=w1273) -> (x != y?=w1269:bool)
        n475 = Not Equal?(x=w1321, y=w1322) -> (x != y?=w1313:bool)
        n476 = Not Equal?(x=w1361, y=w1360) -> (x != y?=w1355:bool)
        n477 = Not Equal?(x=w1298, y=w1301) -> (x != y?=w1290:bool)
        n478 = Not Equal?(x=w1331, y=w1334) -> (x != y?=w1309:bool)
        n479 = Not Equal?(x=w1346, y=w1343) -> (x != y?=w1338:bool)
        n480 = Not Equal?(x=w1275, y=w1272) -> (x != y?=w1268:bool)
        n481 = Not Equal?(x=w1319, y=w1320) -> (x != y?=w1312:bool)
        n482 = Not Equal?(x=w1363, y=w1362) -> (x != y?=w1356:bool)
        n483 = Not Equal?(x=w1297, y=w1302) -> (x != y?=w1289:bool)
        n484 = Not Equal?(x=w1330, y=w1335) -> (x != y?=w1308:bool)
        n485 = Not Equal?(x=w1347, y=w1342) -> (x != y?=w1339:bool)
        n486 = Not Equal?(x=w1276, y=w1271) -> (x != y?=w1267:bool)
        n487 = Not Equal?(x=w1317, y=w1318) -> (x != y?=w1311:bool)
        n488 = Not Equal?(x=w1365, y=w1364) -> (x != y?=w1357:bool)
        n489 = Not Equal?(x=w1296, y=w1303) -> (x != y?=w1288:bool)
        n490 = Not Equal?(x=w1329, y=w1336) -> (x != y?=w1307:bool)
        n491 = Not Equal?(x=w1348, y=w1341) -> (x != y?=w1340:bool)
        n492 = Not Equal?(x=w1277, y=w1270) -> (x != y?=w1266:bool)
      }
      frame #1 {
        n493 = Build Array(w1427, w1426, w1425, w1424) -> (w1393:bool[])
        n494 = Build Array(w1412, w1415, w1414, w1413) -> (w1397:bool[])
        n495 = Build Array(w1421, w1423, w1422, w1420) -> (w1403:bool[])
        n496 = Build Array(w1411, w1408, w1409, w1410) -> (w1406:bool[])
        n497 = Build Array(w1419, w1417, w1416, w1418) -> (w1404:bool[])
        n498 = Build Array(w1382, w1381, w1380, w1379) -> (w1385:bool[])
        n499 = Or Array Elements(Boolean array=w1403) -> (logical OR=w1400:bool)
        n500 = Boolean Array To Number(Boolean array=w1403) -> (number=w1399:u32)
        n501 = Or Array Elements(Boolean array=w1393) -> (logical OR=w1394:bool)
        n502 = Or Array Elements(Boolean array=w1397) -> (logical OR=w1398:bool)
        n503 = Boolean Array To Number(Boolean array=w1393) -> (number=w1395:u32)
        n504 = Boolean Array To Number(Boolean array=w1397) -> (number=w1396:u32)
        n505 = Or Array Elements(Boolean array=w1404) -> (logical OR=w1402:bool)
        n506 = Boolean Array To Number(Boolean array=w1404) -> (number=w1401:u32)
        n507 = Or Array Elements(Boolean array=w1406) -> (logical OR=w1407:bool)
        n508 = Boolean Array To Number(Boolean array=w1406) -> (number=w1405:u32)
        n509 = Or Array Elements(Boolean array=w1385) -> (logical OR=w1384:bool)
        n510 = Boolean Array To Number(Boolean array=w1385) -> (number=w1383:u32)
        n511 = case shown="True" w1394 {
          tunnel: w1395 -> [_ w1455]
          frame False {
          }
          frame True {
            n512 = property on="DISC 05" class="Bool (strict)"() -> ("Value"=w1452:bool)  [unwired: 2 in, 2 out]
            n513 = property on="projector 05" class="Bool (strict)"() -> ("Value"=w1453:bool)  [unwired: 2 in, 2 out]
            n514 = property on="AUTO/MAN 05" class="Bool (strict)"() -> ("Value"=w1451:bool)  [unwired: 2 in, 2 out]
            n515 = property on="cam 05" class="Bool (strict)"() -> ("Value"=w1454:bool)  [unwired: 2 in, 2 out]
            n516 = call "save log.vi"("camera"=w1454, "auto/man"=w1451, "projector"=w1453, "disc"=w1452, "Case Num"=w1455, "Disc Number"="Disc 30") -> ("Error out"=w1450:errorcluster)  [unwired: 5 in]
            n517 = shared-variable ".\\Maintenance.lvlib\\error_16"(w1450) -> ()  [unwired: 1 in, 1 out]
          }
        }
        n518 = case shown="True" w1398 {
          tunnel: w1396 -> [_ w1462]
          frame False {
          }
          frame True {
            n519 = property on="DISC 04" class="Bool (strict)"() -> ("Value"=w1459:bool)  [unwired: 2 in, 2 out]
            n520 = property on="projector 04" class="Bool (strict)"() -> ("Value"=w1460:bool)  [unwired: 2 in, 2 out]
            n521 = property on="AUTO/MAN 04" class="Bool (strict)"() -> ("Value"=w1458:bool)  [unwired: 2 in, 2 out]
            n522 = property on="cam 04" class="Bool (strict)"() -> ("Value"=w1461:bool)  [unwired: 2 in, 2 out]
            n523 = call "save log.vi"("camera"=w1461, "auto/man"=w1458, "projector"=w1460, "disc"=w1459, "Case Num"=w1462, "Disc Number"="Disc 29") -> ("Error out"=w1457:errorcluster)  [unwired: 5 in]
            n524 = shared-variable ".\\Maintenance.lvlib\\error_15"(w1457) -> ()  [unwired: 1 in, 1 out]
          }
        }
        n525 = case shown="True" w1400 {
          tunnel: w1399 -> [_ w1469]
          frame False {
          }
          frame True {
            n526 = property on="DISC 03" class="Bool (strict)"() -> ("Value"=w1466:bool)  [unwired: 2 in, 2 out]
            n527 = property on="projector 03" class="Bool (strict)"() -> ("Value"=w1467:bool)  [unwired: 2 in, 2 out]
            n528 = property on="AUTO/MAN 03" class="Bool (strict)"() -> ("Value"=w1465:bool)  [unwired: 2 in, 2 out]
            n529 = property on="cam 03" class="Bool (strict)"() -> ("Value"=w1468:bool)  [unwired: 2 in, 2 out]
            n530 = call "save log.vi"("camera"=w1468, "auto/man"=w1465, "projector"=w1467, "disc"=w1466, "Case Num"=w1469, "Disc Number"="Disc 28") -> ("Error out"=w1464:errorcluster)  [unwired: 5 in]
            n531 = shared-variable ".\\Maintenance.lvlib\\error_14"(w1464) -> ()  [unwired: 1 in, 1 out]
          }
        }
        n532 = case shown="True" w1402 {
          tunnel: w1401 -> [_ w1476]
          frame False {
          }
          frame True {
            n533 = property on="DISC 02" class="Bool (strict)"() -> ("Value"=w1473:bool)  [unwired: 2 in, 2 out]
            n534 = property on="projector 02" class="Bool (strict)"() -> ("Value"=w1474:bool)  [unwired: 2 in, 2 out]
            n535 = property on="AUTO/MAN 02" class="Bool (strict)"() -> ("Value"=w1472:bool)  [unwired: 2 in, 2 out]
            n536 = property on="cam 02" class="Bool (strict)"() -> ("Value"=w1475:bool)  [unwired: 2 in, 2 out]
            n537 = call "save log.vi"("camera"=w1475, "auto/man"=w1472, "projector"=w1474, "disc"=w1473, "Case Num"=w1476, "Disc Number"="Disc 27") -> ("Error out"=w1471:errorcluster)  [unwired: 5 in]
            n538 = shared-variable ".\\Maintenance.lvlib\\error_13"(w1471) -> ()  [unwired: 1 in, 1 out]
          }
        }
        n539 = case shown="True" w1407 {
          tunnel: w1405 -> [_ w1483]
          frame False {
          }
          frame True {
            n540 = property on="DISC 01" class="Bool (strict)"() -> ("Value"=w1480:bool)  [unwired: 2 in, 2 out]
            n541 = property on="projector 01" class="Bool (strict)"() -> ("Value"=w1481:bool)  [unwired: 2 in, 2 out]
            n542 = property on="AUTO/MAN 01" class="Bool (strict)"() -> ("Value"=w1479:bool)  [unwired: 2 in, 2 out]
            n543 = property on="cam 01" class="Bool (strict)"() -> ("Value"=w1482:bool)  [unwired: 2 in, 2 out]
            n544 = call "save log.vi"("camera"=w1482, "auto/man"=w1479, "projector"=w1481, "disc"=w1480, "Case Num"=w1483, "Disc Number"="Disc 26") -> ("Error out"=w1478:errorcluster)  [unwired: 5 in]
            n545 = shared-variable ".\\Maintenance.lvlib\\error_12"(w1478) -> ()  [unwired: 1 in, 1 out]
          }
        }
        n546 = case shown="True" w1384 {
          tunnel: w1383 -> [_ w1448]
          frame False {
          }
          frame True {
            n547 = property on="DISC 06" class="Bool (strict)"() -> ("Value"=w1445:bool)  [unwired: 2 in, 2 out]
            n548 = property on="projector 06" class="Bool (strict)"() -> ("Value"=w1446:bool)  [unwired: 2 in, 2 out]
            n549 = property on="AUTO/MAN 06" class="Bool (strict)"() -> ("Value"=w1444:bool)  [unwired: 2 in, 2 out]
            n550 = property on="cam 06" class="Bool (strict)"() -> ("Value"=w1447:bool)  [unwired: 2 in, 2 out]
            n551 = call "save log.vi"("camera"=w1447, "auto/man"=w1444, "projector"=w1446, "disc"=w1445, "Case Num"=w1448, "Disc Number"="Disc 06") -> ("Error out"=w1443:errorcluster)  [unwired: 5 in]
            n552 = shared-variable ".\\Maintenance.lvlib\\error_16"(w1443) -> ()  [unwired: 1 in, 1 out]
          }
        }
      }
      frame #2 {
        n553 = shared-variable ".\\Maintenance.lvlib\\error_104"() -> (w1498:errorcluster)  [unwired: 1 in, 1 out]
        n554 = shared-variable ".\\Maintenance.lvlib\\error_104"() -> (w1526:errorcluster)  [unwired: 1 in, 1 out]
        n555 = shared-variable ".\\Maintenance.lvlib\\error_84"() -> (w1538:errorcluster)  [unwired: 1 in, 1 out]
        n556 = shared-variable ".\\Maintenance.lvlib\\error_94"() -> (w1532:errorcluster)  [unwired: 1 in, 1 out]
        n557 = shared-variable ".\\D01.lvlib\\LiveViewD01"() -> (w1552:refnum<image>, error out=w1545:errorcluster)  [unwired: 1 in]
        n558 = shared-variable ".\\Maintenance.lvlib\\error_89"() -> (w1535:errorcluster)  [unwired: 1 in, 1 out]
        n559 = shared-variable ".\\Maintenance.lvlib\\error_99"() -> (w1529:errorcluster)  [unwired: 1 in, 1 out]
        n560 = shared-variable ".\\Setting Lib.lvlib\\processing file path"() -> (w1546:path, error out=w1542:errorcluster)  [unwired: 1 in]
        n561 = property on="AUTO/MAN 06" class="Bool (strict)"() -> ("Value"=w1500:bool)  [unwired: 2 in, 2 out]
        n562 = property on="AUTO/MAN 05" class="Bool (strict)"() -> ("Value"=w1513:bool)  [unwired: 2 in, 2 out]
        n563 = property on="DISC 03" class="Bool (strict)"() -> ("Value"=w1522:bool)  [unwired: 2 in, 2 out]
        n564 = property on="AUTO/MAN 03" class="Bool (strict)"() -> ("Value"=w1511:bool)  [unwired: 2 in, 2 out]
        n565 = property on="AUTO/MAN 04" class="Bool (strict)"() -> ("Value"=w1512:bool)  [unwired: 2 in, 2 out]
        n566 = shared-variable ".\\D06.lvlib\\projector 06"() -> (w1489:bool)  [unwired: 1 in, 1 out]
        "projector 06" <- w1489
        n567 = property on="AUTO/MAN 02" class="Bool (strict)"() -> ("Value"=w1510:bool)  [unwired: 2 in, 2 out]
        n568 = property on="DISC 01" class="Bool (strict)"() -> ("Value"=w1520:bool)  [unwired: 2 in, 2 out]
        n569 = property on="AUTO/MAN 01" class="Bool (strict)"() -> ("Value"=w1509:bool)  [unwired: 2 in, 2 out]
        n570 = shared-variable ".\\D05.lvlib\\projector 05"() -> (w1514:bool)  [unwired: 1 in, 1 out]
        "projector 05" <- w1514
        n571 = Unbundle By Name(w1538) -> ("status"=w1537:bool)
        n572 = Unbundle By Name(w1498) -> ("status"=w1497:bool)
        n573 = shared-variable ".\\D04.lvlib\\projector 04"() -> (w1515:bool)  [unwired: 1 in, 1 out]
        "projector 04" <- w1515
        n574 = property on="DISC 02" class="Bool (strict)"() -> ("Value"=w1521:bool)  [unwired: 2 in, 2 out]
        n575 = Unbundle By Name(w1526) -> ("status"=w1527:bool)
        n576 = shared-variable ".\\D02.lvlib\\projector 02"() -> (w1517:bool)  [unwired: 1 in, 1 out]
        "projector 02" <- w1517
        n577 = shared-variable ".\\D01.lvlib\\projector 01"() -> (w1518:bool)  [unwired: 1 in, 1 out]
        "projector 01" <- w1518
        n578 = Unbundle By Name(w1532) -> ("status"=w1533:bool)
        n579 = Unbundle By Name(w1529) -> ("status"=w1530:bool)
        n580 = Unbundle By Name(w1535) -> ("status"=w1536:bool)
        n581 = shared-variable ".\\D03.lvlib\\projector 03"() -> (w1516:bool)  [unwired: 1 in, 1 out]
        "projector 03" <- w1516
        n582 = property on="DISC 04" class="Bool (strict)"() -> ("Value"=w1523:bool)  [unwired: 2 in, 2 out]
        n583 = property on="DISC 06" class="Bool (strict)"() -> ("Value"=w1499:bool)  [unwired: 2 in, 2 out]
        n584 = call "IMAQ Copy"("error in (no error)"=w1545, "Image Dst"=w1553, "Image Src"=w1552) -> ("error out"=w1544:errorcluster, "Image Dst Out"=w1551:T7)  [unwired: 3 in]
        n585 = shared-variable ".\\D01.lvlib\\GradingThrD01"() -> (w1541:dbl[], error out=w1540:errorcluster)  [unwired: 1 in]
        n586 = property on="DISC 05" class="Bool (strict)"() -> ("Value"=w1524:bool)  [unwired: 2 in, 2 out]
        n587 = Not(x=w1537) -> (.not. x?=w1539:bool)
        "cam 01" <- w1539
        n588 = Not(x=w1497) -> (.not. x?=w1488:bool)
        "cam 06" <- w1488
        n589 = property on="DISC 01" class="Bool (strict)"() -> ("Value"=w1519:bool)  [unwired: 2 in, 2 out]
        n590 = Not(x=w1527) -> (.not. x?=w1525:bool)
        "cam 05" <- w1525
        n591 = Not(x=w1533) -> (.not. x?=w1531:bool)
        "cam 03" <- w1531
        n592 = Not(x=w1530) -> (.not. x?=w1528:bool)
        "cam 04" <- w1528
        n593 = Not(x=w1536) -> (.not. x?=w1534:bool)
        "cam 02" <- w1534
        n594 = shared-variable ".\\Maintenance.lvlib\\error_17"(w1544) -> ()  [unwired: 1 in, 1 out]
        n595 = Build Array(w1488, w1489, TRUE ("element"), w1499) -> (w1496:bool[])
        n596 = call "find and draw circles.vi"("Image Src"=w1551, "module path"=w1546, "function name"="get_circels", "initialized array"=w1559, "Image Dst"=w1561, "error in (no error)"=w1542, "session in"=w1558, "Run/Stop"=w1519, "grading Thr"=w1541) -> ("session out"=w1557:refnum<k35>, "circle info"=w1555:dbl[][], "Image Out"=w1556:T7, "error out"=w1543:errorcluster, "pellet detected?"=w1554:bool)  [unwired: 6 in]
        n597 = Build Array(w1525, w1514, TRUE ("element"), w1524) -> (w1563:bool[])
        n598 = Build Array(w1528, w1515, TRUE ("element"), w1523) -> (w1565:bool[])
        n599 = Build Array(w1539, w1518, TRUE ("element"), w1520) -> (w1572:bool[])
        n600 = Build Array(w1531, w1516, TRUE ("element"), w1522) -> (w1567:bool[])
        n601 = Build Array(w1534, w1517, TRUE ("element"), w1521) -> (w1570:bool[])
        n602 = shared-variable ".\\Maintenance.lvlib\\error_22"(w1543) -> ()  [unwired: 1 in, 1 out]
        n603 = And Array Elements(Boolean array=w1567) -> (logical AND=w1579:bool)
        n604 = Not(x=w1496) -> (.not. x?=→"Warning array 06":bool[])
        n605 = Not(x=w1563) -> (.not. x?=→"Warning array 05":bool[])
        n606 = Not(x=w1567) -> (.not. x?=→"Warning array 03":bool[])
        n607 = And Array Elements(Boolean array=w1572) -> (logical AND=w1575:bool)
        n608 = And Array Elements(Boolean array=w1570) -> (logical AND=w1577:bool)
        n609 = And Array Elements(Boolean array=w1565) -> (logical AND=w1580:bool)
        n610 = Not(x=w1579) -> (.not. x?=→"Warning 03":bool)
        n611 = Not(x=w1570) -> (.not. x?=→"Warning array 02":bool[])
        n612 = And Array Elements(Boolean array=w1496) -> (logical AND=w1494:bool)
        n613 = Not(x=w1565) -> (.not. x?=→"Warning array 04":bool[])
        n614 = Not(x=w1572) -> (.not. x?=→"Warning array 01":bool[])
        n615 = And Array Elements(Boolean array=w1563) -> (logical AND=w1582:bool)
        n616 = shared-variable ".\\D01.lvlib\\PelletDetectedD 01"(w1556, error in=w1540) -> (error out=w1562:errorcluster)
        n617 = Bundle By Name(cluster=T2 {"disc 05"=FALSE, "auto/man 05"=FALSE, "projector 05"=FALSE, "cam 05"=FALSE}, "disc 05"=w1499, "auto/man 05"=w1500, "projector 05"=w1489, "cam 05"=w1488) -> (w1492:T2)
        n618 = Bundle By Name(cluster=T2 {"disc 05"=FALSE, "auto/man 05"=FALSE, "projector 05"=FALSE, "cam 05"=FALSE}, "disc 05"=w1524, "auto/man 05"=w1513, "projector 05"=w1514, "cam 05"=w1525) -> (w1586:T2)
        n619 = Bundle By Name(cluster=T5 {"disc 02"=FALSE, "auto/man 02"=FALSE, "projector 02"=FALSE, "cam 02"=FALSE}, "disc 02"=w1521, "auto/man 02"=w1510, "projector 02"=w1517, "cam 02"=w1534) -> (w1603:T5)
        n620 = Bundle By Name(cluster=T3 {"disc 04"=FALSE, "auto/man 04"=FALSE, "projector 04"=FALSE, "cam 04"=FALSE}, "disc 04"=w1523, "auto/man 04"=w1512, "projector 04"=w1515, "cam 04"=w1528) -> (w1599:T3)
        n621 = Bundle By Name(cluster=T6 {"disc 01"=FALSE, "auto/man 01"=FALSE, "projector 01"=FALSE, "cam 01"=FALSE}, "disc 01"=w1520, "auto/man 01"=w1509, "projector 01"=w1518, "cam 01"=w1539) -> (w1608:T6)
        n622 = Bundle By Name(cluster=T4 {"disc 03"=FALSE, "auto/man 03"=FALSE, "projector 03"=FALSE, "cam 03"=FALSE}, "disc 03"=w1522, "auto/man 03"=w1511, "projector 03"=w1516, "cam 03"=w1531) -> (w1596:T4)
        n623 = Not(x=w1575) -> (.not. x?=→"Warning 01":bool)
        n624 = Not(x=w1577) -> (.not. x?=→"Warning 02":bool)
        n625 = Not(x=w1580) -> (.not. x?=→"Warning 04":bool)
        n626 = Not(x=w1494) -> (.not. x?=→"Warning 06":bool)
        n627 = Not(x=w1582) -> (.not. x?=→"Warning 05":bool)
        n628 = Delete From Array(array=w1486, index=1) -> (array with subset deleted=w1493:T15)  [unwired: 1 in, 1 out]
        n629 = Delete From Array(array=w1585, index=1) -> (array with subset deleted=w1584:T16)  [unwired: 1 in, 1 out]
        n630 = Delete From Array(array=w1604, index=1) -> (array with subset deleted=w1601:T14)  [unwired: 1 in, 1 out]
        n631 = Delete From Array(array=w1592, index=1) -> (array with subset deleted=w1600:T18)  [unwired: 1 in, 1 out]
        n632 = Delete From Array(array=w1611, index=1) -> (array with subset deleted=w1609:T13)  [unwired: 1 in, 1 out]
        n633 = Delete From Array(array=w1591, index=1) -> (array with subset deleted=w1595:T17)  [unwired: 1 in, 1 out]
        n634 = Build Array (concatenate)(w1492, w1493) -> (w1485:T15)
        n635 = Build Array (concatenate)(w1608, w1609) -> (w1607:T13)
        n636 = Build Array (concatenate)(w1586, w1584) -> (w1583:T16)
        n637 = Build Array (concatenate)(w1603, w1601) -> (w1602:T14)
        n638 = Build Array (concatenate)(w1599, w1600) -> (w1590:T18)
        n639 = Build Array (concatenate)(w1596, w1595) -> (w1589:T17)
      }
      frame #3 {
        # "Method selection\nMethod 1: threshold calibration (weigth of pelletizes)\nMethod 2: chess calibration (image processing)"
        n640 = shared-variable ".\\Calibration Lib.lvlib\\Method Selection"() -> (w1642:enum32{"Method 1", "Method 2"}, error out=w1632:errorcluster)  [unwired: 1 in]
        n641 = shared-variable ".\\Calibration Lib.lvlib\\calibration matrix D01"(error in=w1632) -> (w1640:dbl[], error out=w1631:errorcluster)
        n642 = Matrix Size(0:w1628) -> (1:w1626:i32)  [unwired: 1 out]
        n643 = property on="DISC 01" class="Bool (strict)"() -> ("Value"=w1624:bool)  [unwired: 2 in, 2 out]
        n644 = Select(t=w1626, s=w1624, f=0) -> (s? t:f=w1625:i32)
        n645 = case shown="\"Method 2\"" w1642 {
          tunnel: w1635 -> [w1658 w1660]
          tunnel: w1640 -> [_ w1666]
          tunnel: w1628 -> [w1659 w1665]
          tunnel: [w1659 w1663] -> w1633
          tunnel: w1620 -> [w1657 w1664]
          tunnel: [w1658 w1660] -> w1634
          tunnel: w1631 -> [w1656 w1661]
          tunnel: [w1657 w1662] -> w1630
          tunnel: [w1656 w1661] -> w1629
          frame "Method 1", Default {
          }
          frame "Method 2" {
            n646 = call "pixel2milimetr.vi"("1*3 Transform Matrix"=w1666, "circle array"=w1665, "Error in"=w1664) -> ("calibrated circles"=w1663:dbl[][], "Error out"=w1662:errorcluster)  [unwired: 11 in]
          }
        }
        n647 = shared-variable ".\\D01.lvlib\\number of pellet 01"(w1625) -> ()  [unwired: 1 in, 1 out]
        n648 = shared-variable ".\\Maintenance.lvlib\\error_27"(w1630, error in=w1629) -> ()  [unwired: 1 out]
      }
      frame #4 {
        w1687 = u16 1 items=["Falling Edge", "Rising Edge"] ("trigger slope")
        n649 = case shown="True" w1680 {
          tunnel: w1703 -> [w1713 w1775]
          tunnel: [w1713 w1771] -> w1702
          tunnel: w1701 -> [w1712 w1770]
          tunnel: [w1712 w1766] -> w1700
          tunnel: w1699 -> [w1714 w1765]
          tunnel: [w1714 w1763] -> w1698
          tunnel: [dbl[] [0.0, 0.0, 0.0, 0.0, 0.0, 0.0, 0.0, 0.0] w1722] -> w1679
          tunnel: w1674 -> [_ w1750]
          tunnel: [errorcluster {"status"=FALSE, "code"=0, "source"=""} ("error IO") w1745] -> w1672
          frame False {
          }
          frame True {
            w1744 = dbl[] [250.047, 512.0, 1000.0, 1953.125, 2744.0, 4096.0, 5832.0]  # fixed threshoulds
            n650 = shared-variable ".\\D01.lvlib\\GradingThrD01"() -> (w1758:dbl[], error out=w1748:errorcluster)  [unwired: 1 in]
            n651 = Index Array(array=w1750, index (col)=2 ("disabled index (col)")) -> (element=w1749:dbl[])  [unwired: 1 in]
            n652 = property on="live grading array size" class="DigNum (strict)"() -> ("Value"=w1753:i32)  [unwired: 2 in, 2 out]
            n653 = shared-variable ".\\Calibration Lib.lvlib\\Method Selection"(error in=w1748) -> (w1754:enum32{"Method 1", "Method 2"}, error out=w1747:errorcluster)
            n654 = property on="avg grading array size" class="DigNum (strict)"() -> ("Value"=w1752:i32)  [unwired: 2 in, 2 out]
            n655 = Array Size(array=w1749) -> (size(s)=w1764:i32)
            n656 = Multiply(x=w1744, y=0.125) -> (x*y=w1743:dbl[])
            n657 = Subtract(x=w1753, y=w1764) -> (x-y=w1773:i32)
            n658 = Subtract(x=w1752, y=w1764) -> (x-y=w1769:i32)
            n659 = Equal?(x=w1754, y=enum32{"Method 1", "Method 2"}."Method 1" ("Method Selection")) -> (x = y?=w1755:bool)
            n660 = property on="DISC 01" class="Bool (strict)"() -> ("Value"=w1737:bool)  [unwired: 2 in, 2 out]
            n661 = Select(t=w1758, s=w1755, f=w1743) -> (s? t:f=w1757:dbl[])
            n662 = property on="DISC 01" class="Bool (strict)"() -> ("Value"=w1736:bool)  [unwired: 2 in, 2 out]
            n663 = call "array managment.vi"("2D array in"=w1775, "col sel"=0, "cir num"=w1764, "index"=w1773, "subarray"=w1749) -> ("2D array out"=w1771:dbl[][], "1D array out"=w1772:dbl[])  [unwired: 13 in]
            n664 = call "array managment.vi"("2D array in"=w1770, "col sel"=0, "cir num"=w1764, "index"=w1769, "subarray"=w1749) -> ("2D array out"=w1766:dbl[][], "1D array out"=w1767:dbl[])  [unwired: 13 in]
            n665 = call "pelletpercents.vi"("Run/Stop"=w1737, "grading threshoulds"=w1757, "Sorted data"=w1772) -> ("Percentage"=w1761:dbl[])  [unwired: 8 in]
            n666 = call "pelletpercents.vi"("Run/Stop"=w1736, "grading threshoulds"=w1757, "Sorted data"=w1767) -> ("Percentage"=w1738:dbl[])  [unwired: 8 in]
            n667 = Number To Fractional String(number=w1761, precision (6)=i16 2) -> (F-format string=w1759:string[])  [unwired: 2 in]
            n668 = Number To Fractional String(number=w1738, precision (6)=i16 2) -> (F-format string=w1741:string[])  [unwired: 2 in]
            n669 = Fract/Exp String To Number(string=w1759) -> (number=w1722:dbl[])  [unwired: 3 in, 1 out]
            n670 = Fract/Exp String To Number(string=w1741) -> (number=w1739:dbl[])  [unwired: 3 in, 1 out]
            n671 = shared-variable ".\\D01.lvlib\\AvgResultArray"(w1739, error in=w1747) -> (error out=w1746:errorcluster)
            n672 = Index Array(array=w1722, index #1=2 ("index")) -> (element #1=w1735:dbl, element #2=w1732:dbl, element #3=w1733:dbl, element #4=w1734:dbl)  [unwired: 3 in]
            n673 = call "grading average.vi"("input array"=w1722) -> ("avg"=w1716:dbl)  [unwired: 10 in]
            n674 = Add(x=w1735, y=w1732) -> (x+y=w1724:dbl)
            "8-12.5 01" <- w1724
            n675 = Add(x=w1733, y=w1734) -> (x+y=w1725:dbl)
            "12.5-16 01" <- w1725
            n676 = Not A Number/Path/Refnum?(number/path/refnum=w1716) -> (NaN/Path/Refnum?=w1718:bool)
            n677 = Select(t=12.0, s=w1718, f=w1716) -> (s? t:f=w1715:dbl)
            "AVG 01" <- w1715
            n678 = property on="DISC 01" class="Bool (strict)"() -> ("Value"=w1721:bool)  [unwired: 2 in, 2 out]
            n679 = shared-variable ".\\D01.lvlib\\liveResultArray"(w1722, error in=w1746) -> (error out=w1745:errorcluster)
            n680 = Add(x=w1725, y=w1724) -> (x+y=→"8-16mm 26":dbl)
            n681 = Select(t=w1715, s=w1721, f=12.0) -> (s? t:f=w1719:dbl)
            n682 = Add(x=w1732, y=w1733) -> (x+y=w1731:dbl)
            "10-14 01" <- w1731
            n683 = call "dif array management.vi"("2D array in"=w1765, "col sel"=0, "new element/subarray"=w1719) -> ("2D array out"=w1763:dbl[][])  [unwired: 15 in, 1 out]
            n684 = Greater Or Equal?(x=w1731, y=70.0) -> (x >= y?=w1729:bool)
            n685 = Select(t=u32 65282 ("Fill Color"), s=w1729, f=u32 4018019 ("Fill Color")) -> (s? t:f=w1727:u32)
            n686 = property on="10-14 01" class="Slide (strict)"("Fill Color"=w1727) -> ()  [unwired: 2 in, 2 out]
          }
        }
        n687 = shared-variable ".\\Setting Lib.lvlib\\data saving period"() -> (w1673:i32, error out=w1671:errorcluster)  [unwired: 1 in]
        n688 = Get Date/Time In Seconds() -> (seconds since 1Jan1904=w1697:timestamp)
        n689 = Seconds To Date/Time(time stamp (now)=w1697) -> (date time rec=w1696:T19)  [unwired: 1 in]
        n690 = Unbundle By Name(w1696) -> ("minute"=w1695:i32)
        n691 = Quotient & Remainder(x=w1695, y=w1673) -> (x-y*floor(x/y)=w1694:i32)  [unwired: 1 out]
        n692 = Equal To 0?(x=w1694) -> (x = 0?=w1693:bool)
        n693 = Boolean To (0,1)(Boolean=w1693) -> (0, 1=w1692:i16)
        n694 = Get Date/Time In Seconds() -> (seconds since 1Jan1904=w1690:timestamp)
        n695 = Build Array(w1692) -> (w1691:i16[])
        n696 = Bundle By Name("Y"=w1691, "t0"=w1690) -> (w1689:waveform(i16))  [unwired: 1 in]
        n697 = call-poly <vilib>:"Basic Level Trigger Detection.vi"("signal in"=w1689, "level"=0.5, "error in (no error)"=w1671, "trigger slope"=w1687) -> ("trigger detected?"=w1686:bool, "error out"=w1670:errorcluster)  [unwired: 9 in, 1 out]
      }
      frame #5 {
        n698 = shared-variable ".\\D01.lvlib\\SaveD01"(error in=w1784) -> (w1794:bool, error out=w1790:errorcluster)
        n699 = case shown="True" w1805 {
          tunnel: w1791 -> [_ w1840]
          tunnel: w1783 -> [_ w1838]
          frame False {
          }
          frame True {
            w1834 = enum16{"ID Delete", "Time Delete"}."Time Delete" ("Enum")
            n700 = property on="projector 01" class="Bool (strict)"(error in=w1838) -> ("Value"=w1870:bool)  [unwired: 1 in, 2 out]
            n701 = Select(t="ON" ("time format string (%c)"), s=w1870, f="OFF" ("time format string (%c)")) -> (s? t:f=w1871:string)
            n702 = property on="cam 01" class="Bool (strict)"() -> ("Value"=w1868:bool)  [unwired: 2 in, 2 out]
            n703 = Select(t="ON" ("time format string (%c)"), s=w1868, f="OFF" ("time format string (%c)")) -> (s? t:f=w1869:string)
            n704 = property on="AUTO/MAN 01" class="Bool (strict)"() -> ("Value"=w1866:bool)  [unwired: 2 in, 2 out]
            n705 = Select(t="Auto", s=w1866, f="Manual") -> (s? t:f=w1867:string)
            n706 = property on="DISC 01" class="Bool (strict)"() -> ("Value"=w1864:bool)  [unwired: 2 in, 2 out]
            n707 = Select(t="Run", s=w1864, f="Stop") -> (s? t:f=w1865:string)
            n708 = Get Date/Time In Seconds() -> (seconds since 1Jan1904=w1861:timestamp)
            n709 = Format Date/Time String(time format string (%c)="%Y/%m/%d", seconds (now)=w1861) -> (date/time string=w1862:string)  [unwired: 1 in]
            n710 = Format Date/Time String(time format string (%c)="%H:%M:%S", seconds (now)=w1861) -> (date/time string=w1863:string)  [unwired: 1 in]
            n711 = Index Array(array=w1840, index #1=0 ("index")) -> (element #1=w1853:dbl, element #2=w1854:dbl, element #3=w1855:dbl, element #4=w1856:dbl, element #5=w1857:dbl, element #6=w1858:dbl, element #7=w1859:dbl, element #8=w1860:dbl)  [unwired: 7 in]
            n712 = shared-variable ".\\Setting Lib.lvlib\\database refresh period"() -> (w1839:i32, error out=w1837:errorcluster)  [unwired: 1 in]
            n713 = Bundle("date/time string"=w1862, "date/time string"=w1863, w1853, w1854, w1855, w1856, w1857, w1858, w1859, w1860, "f"=w1865, "f"=w1867, "time format string (%c)"=w1869, "time format string (%c)"=w1871) -> (w1841:T20)  [unwired: 1 in]
            n714 = Unbundle(w1841) -> ("date/time string"=w1885:string, "date/time string"=w1884:string, w1883:dbl, w1880:dbl, w1879:dbl, w1882:dbl, "f"=w1877:string, "f"=w1876:string, "time format string (%c)"=w1875:string, "time format string (%c)"=w1872:string)  [unwired: 4 out]
            n715 = Add(x=w1880, y=w1879) -> (x+y=w1878:dbl)
            n716 = Compound Arithmetic op=ADD(w1883, w1880, w1879, w1882) -> (w1881:dbl)
            n717 = To Variant(anything=w1841) -> (Variant=w1886:variant)
            n718 = call "Database.vi"("Maximum Row"=w1839, "Enum"=w1834, "Delete row?"=TRUE, "Data"=w1886, "Error in"=w1837, "Auto Increment ID?"=TRUE, "Table"="grading_disc_26", "Connection"="dsgs") -> ("Error out"=w1836:errorcluster)  [unwired: 3 in]
            n719 = Bundle("date/time string"=w1885, "date/time string"=w1884, w1881, w1878, "f"=w1877, "f"=w1876, "time format string (%c)"=w1875, "time format string (%c)"=w1872) -> (w1874:T21)  [unwired: 1 in]
            n720 = To Variant(anything=w1874) -> (Variant=w1873:variant)
            n721 = call "Database.vi"("Maximum Row"=w1839, "Enum"=w1834, "Delete row?"=TRUE, "Data"=w1873, "Auto Increment ID?"=TRUE, "Table"="main_grading_group_disc_26", "Connection"="dsgs") -> ("Error out"=w1835:errorcluster)  [unwired: 4 in]
            n722 = shared-variable ".\\Maintenance.lvlib\\error_32"(w1836) -> ()  [unwired: 1 in, 1 out]
            n723 = shared-variable ".\\Maintenance.lvlib\\error_33"(w1835) -> ()  [unwired: 1 in, 1 out]
          }
        }
        n724 = Index Array(array=w1799, index (col)=0 ("disabled index (col)")) -> (element=w1797:dbl[])  [unwired: 1 in]
        n725 = Boolean To (0,1)(Boolean=w1794) -> (0, 1=w1795:i16)
        n726 = Build Array(w1795) -> (w1796:i16[])
        n727 = call-poly <vilib>:"Basic Level Trigger Detection.vi"("signal in"=w1796, "level"=0.5, "error in (no error)"=w1790) -> ("trigger detected?"=w1798:bool, "error out"=w1789:errorcluster)  [unwired: 10 in, 1 out]
        n728 = case shown="True" w1798 {
          selector: w1798 -> [_ w1829]
          tunnel: [FALSE w1829] -> w1780
          tunnel: w1797 -> [_ w1824]
          tunnel: w1789 -> [w1815 w1817]
          tunnel: [w1815 w1816] -> w1782
          frame False {
          }
          frame True {
            n729 = Array To Spreadsheet String(array=w1824, 3:"%.2f" ("format string")) -> (spreadsheet string=w1828:string)  [unwired: 1 in]
            n730 = Get Date/Time In Seconds() -> (seconds since 1Jan1904=w1825:timestamp)
            n731 = Format Date/Time String(time format string (%c)="%H:%M:%S", seconds (now)=w1825) -> (date/time string=w1827:string)  [unwired: 1 in]
            n732 = Format Date/Time String(time format string (%c)="%Y/%m/%d", seconds (now)=w1825) -> (date/time string=w1826:string)  [unwired: 1 in]
            n733 = Bundle("date/time string"=w1826, "date/time string"=w1827, "disc 01", "spreadsheet string"=w1828) -> (w1819:T22)  [unwired: 1 in]
            n734 = To Variant(anything=w1819) -> (Variant=w1818:variant)
            n735 = call "Database.vi"("Delete row?"=FALSE, "Data"=w1818, "Error in"=w1817, "Auto Increment ID?"=TRUE, "Table"="thresholds_calibration_table", "Connection"="dsgs") -> ("Error out"=w1816:errorcluster)  [unwired: 5 in]
          }
        }
        n736 = shared-variable ".\\D01.lvlib\\SaveD01Ok"(w1780) -> ()  [unwired: 1 in, 1 out]
        n737 = shared-variable ".\\Maintenance.lvlib\\error_42"(w1782) -> (error out=w1781:errorcluster)  [unwired: 1 in]
      }
      frame #6 {
        n738 = shared-variable ".\\D01.lvlib\\SaveD01"(FALSE ("SaveD26"), error in=w1899) -> (error out=w1898:errorcluster)
        n739 = case shown="8" "speed disc 26" {
          tunnel: w1898 -> [w1922 w1924 w1940 w1956 w1972]
          tunnel: [w1922 w1923 w1939 w1955 w1971] -> w1901
          frame 0, Default {
          }
          frame 1 {
            n740 = Get Date/Time In Seconds() -> (seconds since 1Jan1904=w1938:timestamp)
            n741 = Format Date/Time String(time format string (%c)="%Y/%m/%d", seconds (now)=w1938) -> (date/time string=w1937:string)  [unwired: 1 in]
            n742 = Format Date/Time String(time format string (%c)="%H:%M:%S", seconds (now)=w1938) -> (date/time string=w1936:string)  [unwired: 1 in]
            n743 = Bundle("60001", "date/time string"=w1937, "date/time string"=w1936, "Speed signal is changed and applied in disc 26") -> (w1935:T11)  [unwired: 1 in]
            n744 = To Variant(anything=w1935) -> (Variant=w1934:variant)
            n745 = call "Database.vi"("Maximum Row"=u64 0 ("Storage Time (Day)"), "Delete row?"=FALSE, "Data"=w1934, "Error in"=w1924, "Auto Increment ID?"=TRUE, "Table"="log_table", "Connection"="dsgs") -> ("Error out"=w1923:errorcluster)  [unwired: 4 in]
          }
          frame 2 {
            n746 = Get Date/Time In Seconds() -> (seconds since 1Jan1904=w1954:timestamp)
            n747 = Format Date/Time String(time format string (%c)="%Y/%m/%d", seconds (now)=w1954) -> (date/time string=w1953:string)  [unwired: 1 in]
            n748 = Format Date/Time String(time format string (%c)="%H:%M:%S", seconds (now)=w1954) -> (date/time string=w1952:string)  [unwired: 1 in]
            n749 = Bundle("60002", "date/time string"=w1953, "date/time string"=w1952, "Speed signal is changed and applied in disc 26") -> (w1951:T11)  [unwired: 1 in]
            n750 = To Variant(anything=w1951) -> (Variant=w1950:variant)
            n751 = call "Database.vi"("Maximum Row"=u64 0 ("Storage Time (Day)"), "Delete row?"=FALSE, "Data"=w1950, "Error in"=w1940, "Auto Increment ID?"=TRUE, "Table"="log_table", "Connection"="dsgs") -> ("Error out"=w1939:errorcluster)  [unwired: 4 in]
          }
          frame 4 {
            n752 = Get Date/Time In Seconds() -> (seconds since 1Jan1904=w1970:timestamp)
            n753 = Format Date/Time String(time format string (%c)="%Y/%m/%d", seconds (now)=w1970) -> (date/time string=w1969:string)  [unwired: 1 in]
            n754 = Format Date/Time String(time format string (%c)="%H:%M:%S", seconds (now)=w1970) -> (date/time string=w1968:string)  [unwired: 1 in]
            n755 = Bundle("60003", "date/time string"=w1969, "date/time string"=w1968, "Speed signal is changed but not applied in disc 26") -> (w1967:T11)  [unwired: 1 in]
            n756 = To Variant(anything=w1967) -> (Variant=w1966:variant)
            n757 = call "Database.vi"("Maximum Row"=u64 0 ("Storage Time (Day)"), "Delete row?"=FALSE, "Data"=w1966, "Error in"=w1956, "Auto Increment ID?"=TRUE, "Table"="log_table", "Connection"="dsgs") -> ("Error out"=w1955:errorcluster)  [unwired: 4 in]
          }
          frame 8 {
            n758 = Get Date/Time In Seconds() -> (seconds since 1Jan1904=w1986:timestamp)
            n759 = Format Date/Time String(time format string (%c)="%Y/%m/%d", seconds (now)=w1986) -> (date/time string=w1985:string)  [unwired: 1 in]
            n760 = Format Date/Time String(time format string (%c)="%H:%M:%S", seconds (now)=w1986) -> (date/time string=w1984:string)  [unwired: 1 in]
            n761 = Bundle("60004", "date/time string"=w1985, "date/time string"=w1984, "Speed signal is changed but not applied in disc 26") -> (w1983:T11)  [unwired: 1 in]
            n762 = To Variant(anything=w1983) -> (Variant=w1982:variant)
            n763 = call "Database.vi"("Maximum Row"=u64 0 ("Storage Time (Day)"), "Delete row?"=FALSE, "Data"=w1982, "Error in"=w1972, "Auto Increment ID?"=TRUE, "Table"="log_table", "Connection"="dsgs") -> ("Error out"=w1971:errorcluster)  [unwired: 4 in]
          }
        }
        n764 = shared-variable ".\\Maintenance.lvlib\\error_47"(w1901) -> ()  [unwired: 1 in, 1 out]
      }
      frame #7 {
        n765 = shared-variable ".\\D02.lvlib\\LiveViewD02"() -> (w1991:refnum<image>, error out=w1990:errorcluster)  [unwired: 1 in]
        n766 = property on="DISC 02" class="Bool (strict)"() -> ("Value"=w1992:bool)  [unwired: 2 in, 2 out]
        n767 = shared-variable ".\\Setting Lib.lvlib\\processing file path"() -> (w1999:path, error out=w1995:errorcluster)  [unwired: 1 in]
        n768 = shared-variable ".\\D02.lvlib\\GradingThrD02"() -> (w1994:dbl[], error out=w1993:errorcluster)  [unwired: 1 in]
        n769 = call "IMAQ Copy"("error in (no error)"=w1990, "Image Dst"=w2005, "Image Src"=w1991) -> ("error out"=w1998:errorcluster, "Image Dst Out"=w2004:T7)  [unwired: 3 in]
        n770 = call "find and draw circles.vi"("Image Src"=w2004, "module path"=w1999, "function name"="get_circels", "initialized array"=w2016, "Image Dst"=w2012, "error in (no error)"=w1995, "session in"=w2022, "Run/Stop"=w1992, "grading Thr"=w1994) -> ("session out"=w2021:refnum<k35>, "circle info"=w2015:dbl[][], "Image Out"=w2023:T7, "error out"=w1997:errorcluster, "pellet detected?"=w2000:bool)  [unwired: 6 in]
        n771 = shared-variable ".\\Maintenance.lvlib\\error_18"(w1998) -> ()  [unwired: 1 in, 1 out]
        n772 = shared-variable ".\\Maintenance.lvlib\\error_23"(w1997) -> ()  [unwired: 1 in, 1 out]
        n773 = shared-variable ".\\D02.lvlib\\PelletDetectedD02"(w2023, error in=w1993) -> (error out=w1996:errorcluster)
      }
      frame #8 {
        n774 = shared-variable ".\\Calibration Lib.lvlib\\calibration matrix D02"() -> (w2029:dbl[], error out=w2038:errorcluster)  [unwired: 1 in]
        n775 = Matrix Size(0:w2034) -> (1:w2032:i32)  [unwired: 1 out]
        n776 = property on="DISC 02" class="Bool (strict)"() -> ("Value"=w2031:bool)  [unwired: 2 in, 2 out]
        n777 = Select(t=w2032, s=w2031, f=0) -> (s? t:f=w2030:i32)
        n778 = shared-variable ".\\Calibration Lib.lvlib\\Method Selection"(error in=w2038) -> (w2043:enum32{"Method 1", "Method 2"}, error out=w2035:errorcluster)
        n779 = shared-variable ".\\D02.lvlib\\number of pellet 02"(w2030) -> ()  [unwired: 1 in, 1 out]
        n780 = case shown="\"Method 2\"" w2043 {
          tunnel: w2042 -> [w2061 w2064]
          tunnel: w2029 -> [_ w2070]
          tunnel: w2034 -> [w2063 w2069]
          tunnel: [w2063 w2067] -> w2040
          tunnel: w2025 -> [w2062 w2068]
          tunnel: [w2062 w2066] -> w2037
          tunnel: [w2061 w2064] -> w2041
          tunnel: [w2060 w2065] -> w2036
          tunnel: w2035 -> [w2060 w2065]
          frame "Method 1", Default {
          }
          frame "Method 2" {
            n781 = call "pixel2milimetr.vi"("1*3 Transform Matrix"=w2070, "circle array"=w2069, "Error in"=w2068) -> ("calibrated circles"=w2067:dbl[][], "Error out"=w2066:errorcluster)  [unwired: 11 in]
          }
        }
        n782 = shared-variable ".\\Maintenance.lvlib\\error_28"(w2037, error in=w2036) -> ()  [unwired: 1 out]
      }
      frame #9 {
        n783 = case shown="True" w2075 {
          tunnel: w2092 -> [_ w2163]
          tunnel: w2091 -> [w2101 w2160]
          tunnel: [w2101 w2159] -> w2090
          tunnel: w2089 -> [w2102 w2154]
          tunnel: [w2102 w2153] -> w2088
          tunnel: w2087 -> [w2100 w2150]
          tunnel: [w2100 w2149] -> w2086
          tunnel: [dbl[] [0.0, 0.0, 0.0, 0.0, 0.0, 0.0, 0.0, 0.0] w2113] -> w2076
          tunnel: [errorcluster {"status"=FALSE, "code"=0, "source"=""} ("error IO") w2133] -> w2074
          frame False {
          }
          frame True {
            w2112 = dbl[] [250.047, 512.0, 1000.0, 1953.125, 2744.0, 4096.0, 5832.0]  # fixed threshoulds
            n784 = shared-variable ".\\D02.lvlib\\GradingThrD02"() -> (w2138:dbl[], error out=w2136:errorcluster)  [unwired: 1 in]
            n785 = Index Array(array=w2163, index (col)=2 ("disabled index (col)")) -> (element=w2151:dbl[])  [unwired: 1 in]
            n786 = property on="live grading array size" class="DigNum (strict)"() -> ("Value"=w2143:i32)  [unwired: 2 in, 2 out]
            n787 = property on="avg grading array size" class="DigNum (strict)"() -> ("Value"=w2142:i32)  [unwired: 2 in, 2 out]
            n788 = shared-variable ".\\Calibration Lib.lvlib\\Method Selection"(error in=w2136) -> (w2139:enum32{"Method 1", "Method 2"}, error out=w2135:errorcluster)
            n789 = Array Size(array=w2151) -> (size(s)=w2152:i32)
            n790 = Subtract(x=w2143, y=w2152) -> (x-y=w2162:i32)
            n791 = Subtract(x=w2142, y=w2152) -> (x-y=w2155:i32)
            n792 = Multiply(x=w2112, y=0.25) -> (x*y=w2111:dbl[])
            n793 = Equal?(x=w2139, y=enum32{"Method 1", "Method 2"}."Method 1" ("Method Selection")) -> (x = y?=w2140:bool)
            n794 = property on="DISC 02" class="Bool (strict)"() -> ("Value"=w2128:bool)  [unwired: 2 in, 2 out]
            n795 = property on="DISC 02" class="Bool (strict)"() -> ("Value"=w2127:bool)  [unwired: 2 in, 2 out]
            n796 = call "array managment.vi"("2D array in"=w2160, "col sel"=1, "cir num"=w2152, "index"=w2162, "subarray"=w2151) -> ("2D array out"=w2159:dbl[][], "1D array out"=w2158:dbl[])  [unwired: 13 in]
            n797 = call "array managment.vi"("2D array in"=w2154, "col sel"=1, "cir num"=w2152, "index"=w2155, "subarray"=w2151) -> ("2D array out"=w2153:dbl[][], "1D array out"=w2157:dbl[])  [unwired: 13 in]
            n798 = Select(t=w2138, s=w2140, f=w2111) -> (s? t:f=w2137:dbl[])
            n799 = call "pelletpercents.vi"("Run/Stop"=w2127, "grading threshoulds"=w2137, "Sorted data"=w2158) -> ("Percentage"=w2144:dbl[])  [unwired: 8 in]
            n800 = call "pelletpercents.vi"("Run/Stop"=w2128, "grading threshoulds"=w2137, "Sorted data"=w2157) -> ("Percentage"=w2130:dbl[])  [unwired: 8 in]
            n801 = Number To Fractional String(number=w2130, precision (6)=i16 2) -> (F-format string=w2132:string[])  [unwired: 2 in]
            n802 = Number To Fractional String(number=w2144, precision (6)=i16 2) -> (F-format string=w2145:string[])  [unwired: 2 in]
            n803 = Fract/Exp String To Number(string=w2132) -> (number=w2129:dbl[])  [unwired: 3 in, 1 out]
            n804 = Fract/Exp String To Number(string=w2145) -> (number=w2113:dbl[])  [unwired: 3 in, 1 out]
            n805 = shared-variable ".\\D02.lvlib\\AvgResultD02"(w2129, error in=w2135) -> (error out=w2134:errorcluster)
            n806 = call "grading average.vi"("input array"=w2113) -> ("avg"=w2107:dbl)  [unwired: 10 in]
            "AVG 02" <- w2107
            n807 = property on="DISC 02" class="Bool (strict)"() -> ("Value"=w2106:bool)  [unwired: 2 in, 2 out]
            n808 = Index Array(array=w2113, index #1=2 ("index")) -> (element #1=w2126:dbl, element #2=w2123:dbl, element #3=w2124:dbl, element #4=w2125:dbl)  [unwired: 3 in]
            n809 = Not A Number/Path/Refnum?(number/path/refnum=w2107) -> (NaN/Path/Refnum?=w2104:bool)
            n810 = Not(x=w2104) -> (.not. x?=w2103:bool)
            n811 = Add(x=w2126, y=w2123) -> (x+y=w2115:dbl)
            "8-12.5 02" <- w2115
            n812 = Add(x=w2124, y=w2125) -> (x+y=w2116:dbl)
            "12.5-16 02" <- w2116
            n813 = And(x=w2106, y=w2103) -> (x .and. y?=w2105:bool)
            n814 = shared-variable ".\\D02.lvlib\\LiveResultD02"(w2113, error in=w2134) -> (error out=w2133:errorcluster)
            n815 = Select(t=w2107, s=w2105, f=12.0) -> (s? t:f=w2108:dbl)
            n816 = Add(x=w2116, y=w2115) -> (x+y=→"8-16mm 27":dbl)
            n817 = Add(x=w2123, y=w2124) -> (x+y=w2118:dbl)
            "10-14 02" <- w2118
            n818 = call "dif array management.vi"("2D array in"=w2150, "col sel"=1, "new element/subarray"=w2108) -> ("2D array out"=w2149:dbl[][])  [unwired: 15 in, 1 out]
            n819 = Greater Or Equal?(x=w2118, y=70.0) -> (x >= y?=w2121:bool)
            n820 = Select(t=u32 65282 ("Fill Color"), s=w2121, f=u32 4018019 ("Fill Color")) -> (s? t:f=w2117:u32)
            n821 = property on="10-14 02" class="Slide (strict)"("Fill Color"=w2117) -> ()  [unwired: 2 in, 2 out]
          }
        }
      }
      frame #10 {
        n822 = case shown="True" w2191 {
          tunnel: w2182 -> [_ w2225]
          frame False {
          }
          frame True {
            w2219 = enum16{"ID Delete", "Time Delete"}."Time Delete" ("Enum")
            n823 = property on="projector 02" class="Bool (strict)"() -> ("Value"=w2254:bool)  [unwired: 2 in, 2 out]
            n824 = Select(t="ON" ("time format string (%c)"), s=w2254, f="OFF" ("time format string (%c)")) -> (s? t:f=w2255:string)
            n825 = property on="cam 02" class="Bool (strict)"() -> ("Value"=w2252:bool)  [unwired: 2 in, 2 out]
            n826 = Select(t="ON" ("time format string (%c)"), s=w2252, f="OFF" ("time format string (%c)")) -> (s? t:f=w2253:string)
            n827 = property on="AUTO/MAN 02" class="Bool (strict)"() -> ("Value"=w2250:bool)  [unwired: 2 in, 2 out]
            n828 = Select(t="Auto", s=w2250, f="Manual") -> (s? t:f=w2251:string)
            n829 = property on="DISC 02" class="Bool (strict)"() -> ("Value"=w2248:bool)  [unwired: 2 in, 2 out]
            n830 = Select(t="Run", s=w2248, f="Stop") -> (s? t:f=w2249:string)
            n831 = Get Date/Time In Seconds() -> (seconds since 1Jan1904=w2245:timestamp)
            n832 = Format Date/Time String(time format string (%c)="%Y/%m/%d", seconds (now)=w2245) -> (date/time string=w2246:string)  [unwired: 1 in]
            n833 = Format Date/Time String(time format string (%c)="%H:%M:%S", seconds (now)=w2245) -> (date/time string=w2247:string)  [unwired: 1 in]
            n834 = Index Array(array=w2225, index #1=0 ("index")) -> (element #1=w2237:dbl, element #2=w2238:dbl, element #3=w2239:dbl, element #4=w2240:dbl, element #5=w2241:dbl, element #6=w2242:dbl, element #7=w2243:dbl, element #8=w2244:dbl)  [unwired: 7 in]
            n835 = shared-variable ".\\Setting Lib.lvlib\\database refresh period"() -> (w2223:i32, error out=w2222:errorcluster)  [unwired: 1 in]
            n836 = Bundle("date/time string"=w2246, "date/time string"=w2247, w2237, w2238, w2239, w2240, w2241, w2242, w2243, w2244, "f"=w2249, "f"=w2251, "time format string (%c)"=w2253, "time format string (%c)"=w2255) -> (w2224:T20)  [unwired: 1 in]
            n837 = Unbundle(w2224) -> ("date/time string"=w2257:string, "date/time string"=w2258:string, w2259:dbl, w2262:dbl, w2263:dbl, w2260:dbl, "f"=w2265:string, "f"=w2266:string, "time format string (%c)"=w2267:string, "time format string (%c)"=w2268:string)  [unwired: 4 out]
            n838 = Add(x=w2262, y=w2263) -> (x+y=w2264:dbl)
            n839 = Compound Arithmetic op=ADD(w2259, w2262, w2263, w2260) -> (w2261:dbl)
            n840 = To Variant(anything=w2224) -> (Variant=w2270:variant)
            n841 = call "Database.vi"("Maximum Row"=w2223, "Enum"=w2219, "Delete row?"=TRUE, "Data"=w2270, "Error in"=w2222, "Auto Increment ID?"=TRUE, "Table"="grading_disc_27", "Connection"="dsgs") -> ("Error out"=w2220:errorcluster)  [unwired: 3 in]
            n842 = Bundle("date/time string"=w2257, "date/time string"=w2258, w2261, w2264, "f"=w2265, "f"=w2266, "time format string (%c)"=w2267, "time format string (%c)"=w2268) -> (w2269:T21)  [unwired: 1 in]
            n843 = shared-variable ".\\Maintenance.lvlib\\error_34"(w2220) -> ()  [unwired: 1 in, 1 out]
            n844 = To Variant(anything=w2269) -> (Variant=w2256:variant)
            n845 = call "Database.vi"("Maximum Row"=w2223, "Enum"=w2219, "Delete row?"=TRUE, "Data"=w2256, "Auto Increment ID?"=TRUE, "Table"="main_grading_group_disc_27", "Connection"="dsgs") -> ("Error out"=w2221:errorcluster)  [unwired: 4 in]
            n846 = shared-variable ".\\Maintenance.lvlib\\error_35"(w2221) -> ()  [unwired: 1 in, 1 out]
          }
        }
        n847 = shared-variable ".\\D02.lvlib\\SaveD02"(error in=w2170) -> (w2176:bool, error out=w2173:errorcluster)
        n848 = Index Array(array=w2171, index (col)=1 ("disabled index (col)")) -> (element=w2179:dbl[])  [unwired: 1 in]
        n849 = Boolean To (0,1)(Boolean=w2176) -> (0, 1=w2177:i16)
        n850 = Build Array(w2177) -> (w2178:i16[])
        n851 = call-poly <vilib>:"Basic Level Trigger Detection.vi"("signal in"=w2178, "level"=0.5, "error in (no error)"=w2173) -> ("trigger detected?"=w2181:bool, "error out"=w2172:errorcluster)  [unwired: 10 in, 1 out]
        n852 = case shown="True" w2181 {
          selector: w2181 -> [_ w2214]
          tunnel: [FALSE w2214] -> w2180
          tunnel: w2179 -> [_ w2209]
          tunnel: w2172 -> [w2200 w2202]
          tunnel: [w2200 w2201] -> w2168
          frame False {
          }
          frame True {
            n853 = Array To Spreadsheet String(array=w2209, 3:"%.2f" ("format string")) -> (spreadsheet string=w2213:string)  [unwired: 1 in]
            n854 = Get Date/Time In Seconds() -> (seconds since 1Jan1904=w2210:timestamp)
            n855 = Format Date/Time String(time format string (%c)="%H:%M:%S", seconds (now)=w2210) -> (date/time string=w2212:string)  [unwired: 1 in]
            n856 = Format Date/Time String(time format string (%c)="%Y/%m/%d", seconds (now)=w2210) -> (date/time string=w2211:string)  [unwired: 1 in]
            n857 = Bundle("date/time string"=w2211, "date/time string"=w2212, "disc 02", "spreadsheet string"=w2213) -> (w2204:T22)  [unwired: 1 in]
            n858 = To Variant(anything=w2204) -> (Variant=w2203:variant)
            n859 = call "Database.vi"("Delete row?"=FALSE, "Data"=w2203, "Error in"=w2202, "Auto Increment ID?"=TRUE, "Table"="thresholds_calibration_table", "Connection"="dsgs") -> ("Error out"=w2201:errorcluster)  [unwired: 5 in]
          }
        }
        n860 = shared-variable ".\\D02.lvlib\\SaveD02Ok"(w2180, error in=w2168) -> (error out=w2169:errorcluster)
        n861 = shared-variable ".\\Maintenance.lvlib\\error_43"(w2168) -> ()  [unwired: 1 in, 1 out]
      }
      frame #11 {
        n862 = shared-variable ".\\D02.lvlib\\SaveD02"(FALSE ("SaveD27"), error in=w2284) -> (error out=w2283:errorcluster)
        n863 = case shown="8" "speed disc 27" {
          tunnel: w2283 -> [w2304 w2306 w2322 w2338 w2354]
          tunnel: [w2304 w2305 w2321 w2337 w2353] -> w2285
          frame 0, Default {
          }
          frame 1 {
            n864 = Get Date/Time In Seconds() -> (seconds since 1Jan1904=w2320:timestamp)
            n865 = Format Date/Time String(time format string (%c)="%Y/%m/%d", seconds (now)=w2320) -> (date/time string=w2319:string)  [unwired: 1 in]
            n866 = Format Date/Time String(time format string (%c)="%H:%M:%S", seconds (now)=w2320) -> (date/time string=w2318:string)  [unwired: 1 in]
            n867 = Bundle("60001", "date/time string"=w2319, "date/time string"=w2318, "Speed signal is changed and applied in disc 27") -> (w2317:T11)  [unwired: 1 in]
            n868 = To Variant(anything=w2317) -> (Variant=w2316:variant)
            n869 = call "Database.vi"("Maximum Row"=u64 0 ("Storage Time (Day)"), "Delete row?"=FALSE, "Data"=w2316, "Error in"=w2306, "Auto Increment ID?"=TRUE, "Table"="log_table", "Connection"="dsgs") -> ("Error out"=w2305:errorcluster)  [unwired: 4 in]
          }
          frame 2 {
            n870 = Get Date/Time In Seconds() -> (seconds since 1Jan1904=w2336:timestamp)
            n871 = Format Date/Time String(time format string (%c)="%Y/%m/%d", seconds (now)=w2336) -> (date/time string=w2335:string)  [unwired: 1 in]
            n872 = Format Date/Time String(time format string (%c)="%H:%M:%S", seconds (now)=w2336) -> (date/time string=w2334:string)  [unwired: 1 in]
            n873 = Bundle("60002", "date/time string"=w2335, "date/time string"=w2334, "Speed signal is changed and applied in disc 27") -> (w2333:T11)  [unwired: 1 in]
            n874 = To Variant(anything=w2333) -> (Variant=w2332:variant)
            n875 = call "Database.vi"("Maximum Row"=u64 0 ("Storage Time (Day)"), "Delete row?"=FALSE, "Data"=w2332, "Error in"=w2322, "Auto Increment ID?"=TRUE, "Table"="log_table", "Connection"="dsgs") -> ("Error out"=w2321:errorcluster)  [unwired: 4 in]
          }
          frame 4 {
            n876 = Get Date/Time In Seconds() -> (seconds since 1Jan1904=w2352:timestamp)
            n877 = Format Date/Time String(time format string (%c)="%Y/%m/%d", seconds (now)=w2352) -> (date/time string=w2351:string)  [unwired: 1 in]
            n878 = Format Date/Time String(time format string (%c)="%H:%M:%S", seconds (now)=w2352) -> (date/time string=w2350:string)  [unwired: 1 in]
            n879 = Bundle("60003", "date/time string"=w2351, "date/time string"=w2350, "Speed signal is changed but not applied in disc 27") -> (w2349:T11)  [unwired: 1 in]
            n880 = To Variant(anything=w2349) -> (Variant=w2348:variant)
            n881 = call "Database.vi"("Maximum Row"=u64 0 ("Storage Time (Day)"), "Delete row?"=FALSE, "Data"=w2348, "Error in"=w2338, "Auto Increment ID?"=TRUE, "Table"="log_table", "Connection"="dsgs") -> ("Error out"=w2337:errorcluster)  [unwired: 4 in]
          }
          frame 8 {
            n882 = Get Date/Time In Seconds() -> (seconds since 1Jan1904=w2368:timestamp)
            n883 = Format Date/Time String(time format string (%c)="%Y/%m/%d", seconds (now)=w2368) -> (date/time string=w2367:string)  [unwired: 1 in]
            n884 = Format Date/Time String(time format string (%c)="%H:%M:%S", seconds (now)=w2368) -> (date/time string=w2366:string)  [unwired: 1 in]
            n885 = Bundle("60004", "date/time string"=w2367, "date/time string"=w2366, "Speed signal is changed but not applied in disc 27") -> (w2365:T11)  [unwired: 1 in]
            n886 = To Variant(anything=w2365) -> (Variant=w2364:variant)
            n887 = call "Database.vi"("Maximum Row"=u64 0 ("Storage Time (Day)"), "Delete row?"=FALSE, "Data"=w2364, "Error in"=w2354, "Auto Increment ID?"=TRUE, "Table"="log_table", "Connection"="dsgs") -> ("Error out"=w2353:errorcluster)  [unwired: 4 in]
          }
        }
        n888 = shared-variable ".\\Maintenance.lvlib\\error_48"(w2285) -> ()  [unwired: 1 in, 1 out]
      }
      frame #12 {
        n889 = shared-variable ".\\D03.lvlib\\LiveViewD03"() -> (w2385:refnum<image>, error out=w2384:errorcluster)  [unwired: 1 in]
        n890 = shared-variable ".\\Setting Lib.lvlib\\processing file path"() -> (w2379:path, error out=w2375:errorcluster)  [unwired: 1 in]
        n891 = shared-variable ".\\D03.lvlib\\GradingThrD03"() -> (w2374:dbl[], error out=w2373:errorcluster)  [unwired: 1 in]
        n892 = call "IMAQ Copy"("error in (no error)"=w2384, "Image Dst"=w2386, "Image Src"=w2385) -> ("error out"=w2378:errorcluster, "Image Dst Out"=w2383:T7)  [unwired: 3 in]
        n893 = property on="DISC 03" class="Bool (strict)"() -> ("Value"=w2372:bool)  [unwired: 2 in, 2 out]
        n894 = shared-variable ".\\Maintenance.lvlib\\error_19"(w2378) -> ()  [unwired: 1 in, 1 out]
        n895 = call "find and draw circles.vi"("Image Src"=w2383, "module path"=w2379, "function name"="get_circels", "initialized array"=w2400, "Image Dst"=w2393, "error in (no error)"=w2375, "session in"=w2402, "Run/Stop"=w2372, "grading Thr"=w2374) -> ("session out"=w2401:refnum<k35>, "circle info"=w2396:dbl[][], "Image Out"=w2404:T7, "error out"=w2377:errorcluster, "pellet detected?"=w2380:bool)  [unwired: 6 in]
        n896 = shared-variable ".\\Maintenance.lvlib\\error_24"(w2377) -> ()  [unwired: 1 in, 1 out]
        n897 = shared-variable ".\\D03.lvlib\\PelletDetectedD03"(w2404, error in=w2373) -> (error out=w2376:errorcluster)
      }
      frame #13 {
        n898 = shared-variable ".\\Calibration Lib.lvlib\\calibration matrix D03"() -> (w2424:dbl[], error out=w2418:errorcluster)  [unwired: 1 in]
        n899 = shared-variable ".\\Calibration Lib.lvlib\\calibration factor D03"(error in=w2415) -> (w2423:sgl, error out=w2416:errorcluster)
        n900 = Matrix Size(0:w2412) -> (1:w2410:i32)  [unwired: 1 out]
        n901 = property on="DISC 03" class="Bool (strict)"() -> ("Value"=w2408:bool)  [unwired: 2 in, 2 out]
        n902 = shared-variable ".\\Calibration Lib.lvlib\\Method Selection"(error in=w2418) -> (w2425:enum32{"Method 1", "Method 2"}, error out=w2417:errorcluster)
        n903 = Select(t=w2410, s=w2408, f=0) -> (s? t:f=w2409:i32)
        n904 = case shown="\"Method 2\"" w2425 {
          tunnel: w2421 -> [w2441 w2444]
          tunnel: w2424 -> [_ w2450]
          tunnel: w2423 -> [_ _]
          tunnel: w2412 -> [w2443 w2449]
          tunnel: [w2443 w2447] -> w2420
          tunnel: w2416 -> [w2442 w2448]
          tunnel: [w2442 w2446] -> w2414
          tunnel: [w2441 w2444] -> w2422
          tunnel: w2417 -> [w2440 w2445]
          tunnel: [w2440 w2445] -> w2413
          frame "Method 1", Default {
          }
          frame "Method 2" {
            n905 = call "pixel2milimetr.vi"("1*3 Transform Matrix"=w2450, "circle array"=w2449, "Error in"=w2448) -> ("calibrated circles"=w2447:dbl[][], "Error out"=w2446:errorcluster)  [unwired: 11 in]
          }
        }
        n906 = shared-variable ".\\D03.lvlib\\number of pellet 03"(w2409) -> ()  [unwired: 1 in, 1 out]
        n907 = shared-variable ".\\Maintenance.lvlib\\error_29"(w2414, error in=w2413) -> ()  [unwired: 1 out]
      }
      frame #14 {
        n908 = case shown="True" w2455 {
          tunnel: w2471 -> [_ w2541]
          tunnel: w2470 -> [w2479 w2537]
          tunnel: [w2479 w2536] -> w2469
          tunnel: w2468 -> [w2478 w2532]
          tunnel: [w2478 w2531] -> w2467
          tunnel: w2466 -> [w2480 w2528]
          tunnel: [w2480 w2526] -> w2465
          tunnel: [dbl[] [0.0, 0.0, 0.0, 0.0, 0.0, 0.0, 0.0, 0.0] w2488] -> w2456
          tunnel: [errorcluster {"status"=FALSE, "code"=0, "source"=""} ("error IO") w2511] -> w2454
          frame False {
          }
          frame True {
            w2509 = dbl[] [250.047, 512.0, 1000.0, 1953.125, 2744.0, 4096.0, 5832.0]  # fixed threshoulds
            n909 = shared-variable ".\\Calibration Lib.lvlib\\Method Selection"() -> (w2517:enum32{"Method 1", "Method 2"}, error out=w2513:errorcluster)  [unwired: 1 in]
            n910 = Index Array(array=w2541, index (col)=2 ("disabled index (col)")) -> (element=w2529:dbl[])  [unwired: 1 in]
            n911 = Array Size(array=w2529) -> (size(s)=w2530:i32)
            n912 = property on="avg grading array size" class="DigNum (strict)"() -> ("Value"=w2521:i32)  [unwired: 2 in, 2 out]
            n913 = property on="live grading array size" class="DigNum (strict)"() -> ("Value"=w2520:i32)  [unwired: 2 in, 2 out]
            n914 = shared-variable ".\\D03.lvlib\\GradingThrD03"(error in=w2513) -> (w2516:dbl[], error out=w2512:errorcluster)
            n915 = Subtract(x=w2520, y=w2530) -> (x-y=w2540:i32)
            n916 = Subtract(x=w2521, y=w2530) -> (x-y=w2535:i32)
            n917 = Multiply(x=w2509, y=0.25) -> (x*y=w2508:dbl[])
            n918 = Equal?(x=w2517, y=enum32{"Method 1", "Method 2"}."Method 1" ("Method Selection")) -> (x = y?=w2518:bool)
            n919 = Select(t=w2516, s=w2518, f=w2508) -> (s? t:f=w2515:dbl[])
            n920 = property on="DISC 03" class="Bool (strict)"() -> ("Value"=w2503:bool)  [unwired: 2 in, 2 out]
            n921 = call "array managment.vi"("2D array in"=w2537, "col sel"=2, "cir num"=w2530, "index"=w2540, "subarray"=w2529) -> ("2D array out"=w2536:dbl[][], "1D array out"=w2539:dbl[])  [unwired: 13 in]
            n922 = call "array managment.vi"("2D array in"=w2532, "col sel"=2, "cir num"=w2530, "index"=w2535, "subarray"=w2529) -> ("2D array out"=w2531:dbl[][], "1D array out"=w2533:dbl[])  [unwired: 13 in]
            n923 = property on="DISC 03" class="Bool (strict)"() -> ("Value"=w2502:bool)  [unwired: 2 in, 2 out]
            n924 = call "pelletpercents.vi"("Run/Stop"=w2503, "grading threshoulds"=w2515, "Sorted data"=w2539) -> ("Percentage"=w2522:dbl[])  [unwired: 8 in]
            n925 = call "pelletpercents.vi"("Run/Stop"=w2502, "grading threshoulds"=w2515, "Sorted data"=w2533) -> ("Percentage"=w2504:dbl[])  [unwired: 8 in]
            n926 = Number To Fractional String(number=w2522, precision (6)=i16 2) -> (F-format string=w2523:string[])  [unwired: 2 in]
            n927 = Number To Fractional String(number=w2504, precision (6)=i16 2) -> (F-format string=w2507:string[])  [unwired: 2 in]
            n928 = Fract/Exp String To Number(string=w2523) -> (number=w2488:dbl[])  [unwired: 3 in, 1 out]
            n929 = property on="DISC 03" class="Bool (strict)"() -> ("Value"=w2484:bool)  [unwired: 2 in, 2 out]
            n930 = Fract/Exp String To Number(string=w2507) -> (number=w2506:dbl[])  [unwired: 3 in, 1 out]
            n931 = call "grading average.vi"("input array"=w2488) -> ("avg"=w2485:dbl)  [unwired: 10 in]
            "AVG 03" <- w2485
            n932 = Not A Number/Path/Refnum?(number/path/refnum=w2485) -> (NaN/Path/Refnum?=w2482:bool)
            n933 = shared-variable ".\\D03.lvlib\\AvgResultD03"(w2506, error in=w2512) -> (error out=w2514:errorcluster)
            n934 = Not(x=w2482) -> (.not. x?=w2481:bool)
            n935 = Index Array(array=w2488, index #1=2 ("index")) -> (element #1=w2501:dbl, element #2=w2498:dbl, element #3=w2499:dbl, element #4=w2500:dbl)  [unwired: 3 in]
            n936 = And(x=w2484, y=w2481) -> (x .and. y?=w2483:bool)
            n937 = Select(t=w2485, s=w2483, f=12.0) -> (s? t:f=w2486:dbl)
            n938 = Add(x=w2501, y=w2498) -> (x+y=w2490:dbl)
            "8-12.5 03" <- w2490
            n939 = Add(x=w2499, y=w2500) -> (x+y=w2491:dbl)
            "12.5-16 03" <- w2491
            n940 = Add(x=w2498, y=w2499) -> (x+y=w2493:dbl)
            "10-14 03" <- w2493
            n941 = shared-variable ".\\D03.lvlib\\LiveResultD03"(w2488, error in=w2514) -> (error out=w2511:errorcluster)
            n942 = Add(x=w2491, y=w2490) -> (x+y=→"8-16mm 03":dbl)
            n943 = call "dif array management.vi"("2D array in"=w2528, "col sel"=2, "new element/subarray"=w2486) -> ("2D array out"=w2526:dbl[][])  [unwired: 15 in, 1 out]
            n944 = Greater Or Equal?(x=w2493, y=70.0) -> (x >= y?=w2496:bool)
            n945 = Select(t=u32 65282 ("Fill Color"), s=w2496, f=u32 4018019 ("Fill Color")) -> (s? t:f=w2492:u32)
            n946 = property on="10-14 03" class="Slide (strict)"("Fill Color"=w2492) -> ()  [unwired: 2 in, 2 out]
          }
        }
      }
      frame #15 {
        n947 = case shown="True" w2567 {
          tunnel: w2559 -> [_ w2599]
          frame False {
          }
          frame True {
            w2594 = enum16{"ID Delete", "Time Delete"}."Time Delete" ("Enum")
            n948 = property on="projector 03" class="Bool (strict)"() -> ("Value"=w2629:bool)  [unwired: 2 in, 2 out]
            n949 = Select(t="ON" ("time format string (%c)"), s=w2629, f="OFF" ("time format string (%c)")) -> (s? t:f=w2630:string)
            n950 = property on="cam 03" class="Bool (strict)"() -> ("Value"=w2627:bool)  [unwired: 2 in, 2 out]
            n951 = Select(t="ON" ("time format string (%c)"), s=w2627, f="OFF" ("time format string (%c)")) -> (s? t:f=w2628:string)
            n952 = property on="AUTO/MAN 03" class="Bool (strict)"() -> ("Value"=w2625:bool)  [unwired: 2 in, 2 out]
            n953 = Select(t="Auto", s=w2625, f="Manual") -> (s? t:f=w2626:string)
            n954 = property on="DISC 03" class="Bool (strict)"() -> ("Value"=w2623:bool)  [unwired: 2 in, 2 out]
            n955 = Select(t="Run", s=w2623, f="Stop") -> (s? t:f=w2624:string)
            n956 = Get Date/Time In Seconds() -> (seconds since 1Jan1904=w2620:timestamp)
            n957 = Format Date/Time String(time format string (%c)="%Y/%m/%d", seconds (now)=w2620) -> (date/time string=w2621:string)  [unwired: 1 in]
            n958 = Format Date/Time String(time format string (%c)="%H:%M:%S", seconds (now)=w2620) -> (date/time string=w2622:string)  [unwired: 1 in]
            n959 = Index Array(array=w2599, index #1=0 ("index")) -> (element #1=w2612:dbl, element #2=w2613:dbl, element #3=w2614:dbl, element #4=w2615:dbl, element #5=w2616:dbl, element #6=w2617:dbl, element #7=w2618:dbl, element #8=w2619:dbl)  [unwired: 7 in]
            n960 = shared-variable ".\\Setting Lib.lvlib\\database refresh period"() -> (w2598:i32, error out=w2597:errorcluster)  [unwired: 1 in]
            n961 = Bundle("date/time string"=w2621, "date/time string"=w2622, w2612, w2613, w2614, w2615, w2616, w2617, w2618, w2619, "f"=w2624, "f"=w2626, "time format string (%c)"=w2628, "time format string (%c)"=w2630) -> (w2600:T20)  [unwired: 1 in]
            n962 = Unbundle(w2600) -> ("date/time string"=w2644:string, "date/time string"=w2643:string, w2642:dbl, w2639:dbl, w2638:dbl, w2641:dbl, "f"=w2636:string, "f"=w2635:string, "time format string (%c)"=w2634:string, "time format string (%c)"=w2633:string)  [unwired: 4 out]
            n963 = Add(x=w2639, y=w2638) -> (x+y=w2637:dbl)
            n964 = Compound Arithmetic op=ADD(w2642, w2639, w2638, w2641) -> (w2640:dbl)
            n965 = To Variant(anything=w2600) -> (Variant=w2645:variant)
            n966 = call "Database.vi"("Maximum Row"=w2598, "Enum"=w2594, "Delete row?"=TRUE, "Data"=w2645, "Error in"=w2597, "Auto Increment ID?"=TRUE, "Table"="grading_disc_28", "Connection"="dsgs") -> ("Error out"=w2596:errorcluster)  [unwired: 3 in]
            n967 = Bundle("date/time string"=w2644, "date/time string"=w2643, w2640, w2637, "f"=w2636, "f"=w2635, "time format string (%c)"=w2634, "time format string (%c)"=w2633) -> (w2632:T21)  [unwired: 1 in]
            n968 = shared-variable ".\\Maintenance.lvlib\\error_36"(w2596) -> ()  [unwired: 1 in, 1 out]
            n969 = To Variant(anything=w2632) -> (Variant=w2631:variant)
            n970 = call "Database.vi"("Maximum Row"=w2598, "Enum"=w2594, "Delete row?"=TRUE, "Data"=w2631, "Auto Increment ID?"=TRUE, "Table"="main_grading_group_disc_28", "Connection"="dsgs") -> ("Error out"=w2595:errorcluster)  [unwired: 4 in]
            n971 = shared-variable ".\\Maintenance.lvlib\\error_37"(w2595) -> ()  [unwired: 1 in, 1 out]
          }
        }
        n972 = shared-variable ".\\D03.lvlib\\SaveD03"(error in=w2547) -> (w2553:bool, error out=w2550:errorcluster)
        n973 = Index Array(array=w2548, index (col)=2 ("disabled index (col)")) -> (element=w2556:dbl[])  [unwired: 1 in]
        n974 = Boolean To (0,1)(Boolean=w2553) -> (0, 1=w2554:i16)
        n975 = Build Array(w2554) -> (w2555:i16[])
        n976 = call-poly <vilib>:"Basic Level Trigger Detection.vi"("signal in"=w2555, "level"=0.5, "error in (no error)"=w2550) -> ("trigger detected?"=w2558:bool, "error out"=w2549:errorcluster)  [unwired: 10 in, 1 out]
        n977 = case shown="True" w2558 {
          selector: w2558 -> [_ w2589]
          tunnel: [FALSE w2589] -> w2557
          tunnel: w2556 -> [_ w2584]
          tunnel: w2549 -> [w2575 w2577]
          tunnel: [w2575 w2576] -> w2546
          frame False {
          }
          frame True {
            n978 = Array To Spreadsheet String(array=w2584, 3:"%.2f" ("format string")) -> (spreadsheet string=w2588:string)  [unwired: 1 in]
            n979 = Get Date/Time In Seconds() -> (seconds since 1Jan1904=w2585:timestamp)
            n980 = Format Date/Time String(time format string (%c)="%H:%M:%S", seconds (now)=w2585) -> (date/time string=w2587:string)  [unwired: 1 in]
            n981 = Format Date/Time String(time format string (%c)="%Y/%m/%d", seconds (now)=w2585) -> (date/time string=w2586:string)  [unwired: 1 in]
            n982 = Bundle("date/time string"=w2586, "date/time string"=w2587, "disc 03", "spreadsheet string"=w2588) -> (w2579:T22)  [unwired: 1 in]
            n983 = To Variant(anything=w2579) -> (Variant=w2578:variant)
            n984 = call "Database.vi"("Delete row?"=FALSE, "Data"=w2578, "Error in"=w2577, "Auto Increment ID?"=TRUE, "Table"="thresholds_calibration_table", "Connection"="dsgs") -> ("Error out"=w2576:errorcluster)  [unwired: 5 in]
          }
        }
        n985 = shared-variable ".\\D03.lvlib\\SaveD03Ok"(w2557, error in=w2546) -> ()  [unwired: 1 out]
        n986 = shared-variable ".\\Maintenance.lvlib\\error_44"(w2546) -> ()  [unwired: 1 in, 1 out]
      }
      frame #16 {
        n987 = shared-variable ".\\D03.lvlib\\SaveD03"(FALSE ("SaveD28"), error in=w2658) -> (error out=w2657:errorcluster)
        n988 = case shown="4" "speed disc 28" {
          tunnel: "Error in 18" -> [w2678 w2680 w2696 w2712 w2728]
          tunnel: [w2678 w2679 w2695 w2711 w2727] -> w2660
          frame 0, Default {
          }
          frame 1 {
            n989 = Get Date/Time In Seconds() -> (seconds since 1Jan1904=w2694:timestamp)
            n990 = Format Date/Time String(time format string (%c)="%Y/%m/%d", seconds (now)=w2694) -> (date/time string=w2693:string)  [unwired: 1 in]
            n991 = Format Date/Time String(time format string (%c)="%H:%M:%S", seconds (now)=w2694) -> (date/time string=w2692:string)  [unwired: 1 in]
            n992 = Bundle("60001", "date/time string"=w2693, "date/time string"=w2692, "Speed signal is changed and applied in disc 28") -> (w2691:T11)  [unwired: 1 in]
            n993 = To Variant(anything=w2691) -> (Variant=w2690:variant)
            n994 = call "Database.vi"("Maximum Row"=u64 0 ("Storage Time (Day)"), "Delete row?"=FALSE, "Data"=w2690, "Error in"=w2680, "Auto Increment ID?"=TRUE, "Table"="log_table", "Connection"="dsgs") -> ("Error out"=w2679:errorcluster)  [unwired: 4 in]
          }
          frame 2 {
            n995 = Get Date/Time In Seconds() -> (seconds since 1Jan1904=w2710:timestamp)
            n996 = Format Date/Time String(time format string (%c)="%Y/%m/%d", seconds (now)=w2710) -> (date/time string=w2709:string)  [unwired: 1 in]
            n997 = Format Date/Time String(time format string (%c)="%H:%M:%S", seconds (now)=w2710) -> (date/time string=w2708:string)  [unwired: 1 in]
            n998 = Bundle("60002", "date/time string"=w2709, "date/time string"=w2708, "Speed signal is changed and applied in disc 28") -> (w2707:T11)  [unwired: 1 in]
            n999 = To Variant(anything=w2707) -> (Variant=w2706:variant)
            n1000 = call "Database.vi"("Maximum Row"=u64 0 ("Storage Time (Day)"), "Delete row?"=FALSE, "Data"=w2706, "Error in"=w2696, "Auto Increment ID?"=TRUE, "Table"="log_table", "Connection"="dsgs") -> ("Error out"=w2695:errorcluster)  [unwired: 4 in]
          }
          frame 4 {
            n1001 = Get Date/Time In Seconds() -> (seconds since 1Jan1904=w2726:timestamp)
            n1002 = Format Date/Time String(time format string (%c)="%Y/%m/%d", seconds (now)=w2726) -> (date/time string=w2725:string)  [unwired: 1 in]
            n1003 = Format Date/Time String(time format string (%c)="%H:%M:%S", seconds (now)=w2726) -> (date/time string=w2724:string)  [unwired: 1 in]
            n1004 = Bundle("60003", "date/time string"=w2725, "date/time string"=w2724, "Speed signal is changed but not applied in disc 28") -> (w2723:T11)  [unwired: 1 in]
            n1005 = To Variant(anything=w2723) -> (Variant=w2722:variant)
            n1006 = call "Database.vi"("Maximum Row"=u64 0 ("Storage Time (Day)"), "Delete row?"=FALSE, "Data"=w2722, "Error in"=w2712, "Auto Increment ID?"=TRUE, "Table"="log_table", "Connection"="dsgs") -> ("Error out"=w2711:errorcluster)  [unwired: 4 in]
          }
          frame 8 {
            n1007 = Get Date/Time In Seconds() -> (seconds since 1Jan1904=w2742:timestamp)
            n1008 = Format Date/Time String(time format string (%c)="%Y/%m/%d", seconds (now)=w2742) -> (date/time string=w2741:string)  [unwired: 1 in]
            n1009 = Format Date/Time String(time format string (%c)="%H:%M:%S", seconds (now)=w2742) -> (date/time string=w2740:string)  [unwired: 1 in]
            n1010 = Bundle("60004", "date/time string"=w2741, "date/time string"=w2740, "Speed signal is changed but not applied in disc 28") -> (w2739:T11)  [unwired: 1 in]
            n1011 = To Variant(anything=w2739) -> (Variant=w2738:variant)
            n1012 = call "Database.vi"("Maximum Row"=u64 0 ("Storage Time (Day)"), "Delete row?"=FALSE, "Data"=w2738, "Error in"=w2728, "Auto Increment ID?"=TRUE, "Table"="log_table", "Connection"="dsgs") -> ("Error out"=w2727:errorcluster)  [unwired: 4 in]
          }
        }
        n1013 = shared-variable ".\\Maintenance.lvlib\\error_49"(w2660) -> ()  [unwired: 1 in, 1 out]
      }
      frame #17 {
        n1014 = shared-variable ".\\Setting Lib.lvlib\\processing file path"(error in=w2746) -> (w2754:path, error out=w2752:errorcluster)
        n1015 = shared-variable ".\\D04.lvlib\\LiveViewD04"() -> (w2759:refnum<image>, error out=w2757:errorcluster)  [unwired: 1 in]
        n1016 = shared-variable ".\\D04.lvlib\\GradingThrD04"() -> (w2749:dbl[], error out=w2748:errorcluster)  [unwired: 1 in]
        n1017 = property on="DISC 04" class="Bool (strict)"() -> ("Value"=w2747:bool)  [unwired: 2 in, 2 out]
        n1018 = call "IMAQ Copy"("error in (no error)"=w2757, "Image Dst"=w2760, "Image Src"=w2759) -> ("error out"=w2753:errorcluster, "Image Dst Out"=w2758:T7)  [unwired: 3 in]
        n1019 = call "find and draw circles.vi"("Image Src"=w2758, "module path"=w2754, "function name"="get_circels", "initialized array"=w2772, "Image Dst"=w2767, "error in (no error)"=w2752, "session in"=w2775, "Run/Stop"=w2747, "grading Thr"=w2749) -> ("session out"=w2774:refnum<k35>, "circle info"=w2770:dbl[][], "Image Out"=w2776:T7, "error out"=w2750:errorcluster, "pellet detected?"=w2755:bool)  [unwired: 6 in]
        n1020 = shared-variable ".\\Maintenance.lvlib\\error_20"(w2753) -> ()  [unwired: 1 in, 1 out]
        n1021 = shared-variable ".\\Maintenance.lvlib\\error_25"(w2750) -> ()  [unwired: 1 in, 1 out]
        n1022 = shared-variable ".\\D04.lvlib\\PelletDetectedD04"(w2776, error in=w2748) -> (error out=w2751:errorcluster)
      }
      frame #18 {
        n1023 = shared-variable ".\\Calibration Lib.lvlib\\calibration matrix D04"() -> (w2795:dbl[], error out=w2789:errorcluster)  [unwired: 1 in]
        n1024 = Matrix Size(0:w2786) -> (1:w2784:i32)  [unwired: 1 out]
        n1025 = property on="DISC 04" class="Bool (strict)"() -> ("Value"=w2782:bool)  [unwired: 2 in, 2 out]
        n1026 = shared-variable ".\\Calibration Lib.lvlib\\Method Selection"(error in=w2789) -> (w2796:enum32{"Method 1", "Method 2"}, error out=w2790:errorcluster)
        n1027 = Select(t=w2784, s=w2782, f=0) -> (s? t:f=w2783:i32)
        n1028 = shared-variable ".\\D04.lvlib\\number of pellet 04"(w2783) -> ()  [unwired: 1 in, 1 out]
        n1029 = case shown="\"Method 2\"" w2796 {
          tunnel: w2792 -> [w2810 w2813]
          tunnel: w2795 -> [_ w2819]
          tunnel: w2786 -> [w2812 w2818]
          tunnel: [w2812 w2816] -> w2793
          tunnel: w2778 -> [w2811 w2817]
          tunnel: [w2811 w2815] -> w2788
          tunnel: [w2810 w2813] -> w2794
          tunnel: w2790 -> [w2809 w2814]
          tunnel: [w2809 w2814] -> w2787
          frame "Method 1", Default {
          }
          frame "Method 2" {
            n1030 = call "pixel2milimetr.vi"("1*3 Transform Matrix"=w2819, "circle array"=w2818, "Error in"=w2817) -> ("calibrated circles"=w2816:dbl[][], "Error out"=w2815:errorcluster)  [unwired: 11 in]
          }
        }
        n1031 = shared-variable ".\\Maintenance.lvlib\\error_30"(w2788, error in=w2787) -> ()  [unwired: 1 out]
      }
      frame #19 {
        n1032 = case shown="True" w2824 {
          tunnel: w2839 -> [_ w2908]
          tunnel: w2838 -> [w2845 w2904]
          tunnel: [w2845 w2903] -> w2837
          tunnel: w2836 -> [w2844 w2899]
          tunnel: [w2844 w2898] -> w2835
          tunnel: w2834 -> [w2846 w2894]
          tunnel: [w2846 w2893] -> w2833
          tunnel: [dbl[] [0.0, 0.0, 0.0, 0.0, 0.0, 0.0, 0.0, 0.0] w2855] -> w2825
          tunnel: [errorcluster {"status"=FALSE, "code"=0, "source"=""} ("error IO") w2878] -> w2823
          frame False {
          }
          frame True {
            w2875 = dbl[] [250.047, 512.0, 1000.0, 1953.125, 2744.0, 4096.0, 5832.0]  # fixed threshoulds
            n1033 = shared-variable ".\\Calibration Lib.lvlib\\Method Selection"() -> (w2884:enum32{"Method 1", "Method 2"}, error out=w2881:errorcluster)  [unwired: 1 in]
            n1034 = Index Array(array=w2908, index (col)=2 ("disabled index (col)")) -> (element=w2896:dbl[])  [unwired: 1 in]
            n1035 = property on="avg grading array size" class="DigNum (strict)"() -> ("Value"=w2887:i32)  [unwired: 2 in, 2 out]
            n1036 = property on="live grading array size" class="DigNum (strict)"() -> ("Value"=w2888:i32)  [unwired: 2 in, 2 out]
            n1037 = Array Size(array=w2896) -> (size(s)=w2897:i32)
            n1038 = shared-variable ".\\D04.lvlib\\GradingThrD04"(error in=w2881) -> (w2882:dbl[], error out=w2880:errorcluster)
            n1039 = Subtract(x=w2888, y=w2897) -> (x-y=w2906:i32)
            n1040 = Subtract(x=w2887, y=w2897) -> (x-y=w2900:i32)
            n1041 = Multiply(x=w2875, y=0.25) -> (x*y=w2876:dbl[])
            n1042 = Equal?(x=w2884, y=enum32{"Method 1", "Method 2"}."Method 1" ("Method Selection")) -> (x = y?=w2885:bool)
            n1043 = call "array managment.vi"("2D array in"=w2904, "col sel"=3, "cir num"=w2897, "index"=w2906, "subarray"=w2896) -> ("2D array out"=w2903:dbl[][], "1D array out"=w2905:dbl[])  [unwired: 13 in]
            n1044 = call "array managment.vi"("2D array in"=w2899, "col sel"=3, "cir num"=w2897, "index"=w2900, "subarray"=w2896) -> ("2D array out"=w2898:dbl[][], "1D array out"=w2902:dbl[])  [unwired: 13 in]
            n1045 = property on="DISC 04" class="Bool (strict)"() -> ("Value"=w2870:bool)  [unwired: 2 in, 2 out]
            n1046 = Select(t=w2882, s=w2885, f=w2876) -> (s? t:f=w2883:dbl[])
            n1047 = property on="DISC 04" class="Bool (strict)"() -> ("Value"=w2869:bool)  [unwired: 2 in, 2 out]
            n1048 = call "pelletpercents.vi"("Run/Stop"=w2870, "grading threshoulds"=w2883, "Sorted data"=w2905) -> ("Percentage"=w2889:dbl[])  [unwired: 8 in]
            n1049 = call "pelletpercents.vi"("Run/Stop"=w2869, "grading threshoulds"=w2883, "Sorted data"=w2902) -> ("Percentage"=w2871:dbl[])  [unwired: 8 in]
            n1050 = Number To Fractional String(number=w2889, precision (6)=i16 2) -> (F-format string=w2890:string[])  [unwired: 2 in]
            n1051 = Number To Fractional String(number=w2871, precision (6)=i16 2) -> (F-format string=w2874:string[])  [unwired: 2 in]
            n1052 = Fract/Exp String To Number(string=w2890) -> (number=w2855:dbl[])  [unwired: 3 in, 1 out]
            n1053 = property on="DISC 04" class="Bool (strict)"() -> ("Value"=w2851:bool)  [unwired: 2 in, 2 out]
            n1054 = Fract/Exp String To Number(string=w2874) -> (number=w2873:dbl[])  [unwired: 3 in, 1 out]
            n1055 = call "grading average.vi"("input array"=w2855) -> ("avg"=w2852:dbl)  [unwired: 10 in]
            "AVG 04" <- w2852
            n1056 = Not A Number/Path/Refnum?(number/path/refnum=w2852) -> (NaN/Path/Refnum?=w2849:bool)
            n1057 = shared-variable ".\\D04.lvlib\\AvgResultD04"(w2873, error in=w2880) -> (error out=w2879:errorcluster)
            n1058 = Index Array(array=w2855, index #1=2 ("index")) -> (element #1=w2868:dbl, element #2=w2865:dbl, element #3=w2866:dbl, element #4=w2867:dbl)  [unwired: 3 in]
            n1059 = Not(x=w2849) -> (.not. x?=w2848:bool)
            n1060 = And(x=w2851, y=w2848) -> (x .and. y?=w2850:bool)
            n1061 = Add(x=w2868, y=w2865) -> (x+y=w2857:dbl)
            "8-12.5 04" <- w2857
            n1062 = Add(x=w2866, y=w2867) -> (x+y=w2858:dbl)
            "12.5-16 04" <- w2858
            n1063 = Add(x=w2865, y=w2866) -> (x+y=w2860:dbl)
            "10-14 04" <- w2860
            n1064 = Select(t=w2852, s=w2850, f=12.0) -> (s? t:f=w2853:dbl)
            n1065 = shared-variable ".\\D04.lvlib\\LiveResultD04"(w2855, error in=w2879) -> (error out=w2878:errorcluster)
            n1066 = Add(x=w2858, y=w2857) -> (x+y=→"8-16mm 04":dbl)
            n1067 = call "dif array management.vi"("2D array in"=w2894, "col sel"=3, "new element/subarray"=w2853) -> ("2D array out"=w2893:dbl[][])  [unwired: 15 in, 1 out]
            n1068 = Greater Or Equal?(x=w2860, y=70.0) -> (x >= y?=w2863:bool)
            n1069 = Select(t=u32 65282 ("Fill Color"), s=w2863, f=u32 4018019 ("Fill Color")) -> (s? t:f=w2859:u32)
            n1070 = property on="10-14 04" class="Slide (strict)"("Fill Color"=w2859) -> ()  [unwired: 2 in, 2 out]
          }
        }
      }
      frame #20 {
        n1071 = case shown="True" w2934 {
          tunnel: w2927 -> [_ w2965]
          frame False {
          }
          frame True {
            w2960 = enum16{"ID Delete", "Time Delete"}."Time Delete" ("Enum")
            n1072 = property on="projector 04" class="Bool (strict)"() -> ("Value"=w2995:bool)  [unwired: 2 in, 2 out]
            n1073 = Select(t="ON" ("time format string (%c)"), s=w2995, f="OFF" ("time format string (%c)")) -> (s? t:f=w2996:string)
            n1074 = property on="cam 04" class="Bool (strict)"() -> ("Value"=w2993:bool)  [unwired: 2 in, 2 out]
            n1075 = Select(t="ON" ("time format string (%c)"), s=w2993, f="OFF" ("time format string (%c)")) -> (s? t:f=w2994:string)
            n1076 = property on="AUTO/MAN 04" class="Bool (strict)"() -> ("Value"=w2991:bool)  [unwired: 2 in, 2 out]
            n1077 = Select(t="Auto", s=w2991, f="Manual") -> (s? t:f=w2992:string)
            n1078 = property on="DISC 04" class="Bool (strict)"() -> ("Value"=w2989:bool)  [unwired: 2 in, 2 out]
            n1079 = Select(t="Run", s=w2989, f="Stop") -> (s? t:f=w2990:string)
            n1080 = Get Date/Time In Seconds() -> (seconds since 1Jan1904=w2986:timestamp)
            n1081 = Format Date/Time String(time format string (%c)="%Y/%m/%d", seconds (now)=w2986) -> (date/time string=w2987:string)  [unwired: 1 in]
            n1082 = Format Date/Time String(time format string (%c)="%H:%M:%S", seconds (now)=w2986) -> (date/time string=w2988:string)  [unwired: 1 in]
            n1083 = Index Array(array=w2965, index #1=0 ("index")) -> (element #1=w2978:dbl, element #2=w2979:dbl, element #3=w2980:dbl, element #4=w2981:dbl, element #5=w2982:dbl, element #6=w2983:dbl, element #7=w2984:dbl, element #8=w2985:dbl)  [unwired: 7 in]
            n1084 = Bundle("date/time string"=w2987, "date/time string"=w2988, w2978, w2979, w2980, w2981, w2982, w2983, w2984, w2985, "f"=w2990, "f"=w2992, "time format string (%c)"=w2994, "time format string (%c)"=w2996) -> (w2966:T20)  [unwired: 1 in]
            n1085 = shared-variable ".\\Setting Lib.lvlib\\database refresh period"() -> (w2964:i32, error out=w2963:errorcluster)  [unwired: 1 in]
            n1086 = Unbundle(w2966) -> ("date/time string"=w3010:string, "date/time string"=w3009:string, w3008:dbl, w3005:dbl, w3004:dbl, w3007:dbl, "f"=w3002:string, "f"=w3001:string, "time format string (%c)"=w3000:string, "time format string (%c)"=w2999:string)  [unwired: 4 out]
            n1087 = Add(x=w3005, y=w3004) -> (x+y=w3003:dbl)
            n1088 = Compound Arithmetic op=ADD(w3008, w3005, w3004, w3007) -> (w3006:dbl)
            n1089 = To Variant(anything=w2966) -> (Variant=w3011:variant)
            n1090 = call "Database.vi"("Maximum Row"=w2964, "Enum"=w2960, "Delete row?"=TRUE, "Data"=w3011, "Error in"=w2963, "Auto Increment ID?"=TRUE, "Table"="grading_disc_29", "Connection"="dsgs") -> ("Error out"=w2962:errorcluster)  [unwired: 3 in]
            n1091 = Bundle("date/time string"=w3010, "date/time string"=w3009, w3006, w3003, "f"=w3002, "f"=w3001, "time format string (%c)"=w3000, "time format string (%c)"=w2999) -> (w2998:T21)  [unwired: 1 in]
            n1092 = shared-variable ".\\Maintenance.lvlib\\error_38"(w2962) -> ()  [unwired: 1 in, 1 out]
            n1093 = To Variant(anything=w2998) -> (Variant=w2997:variant)
            n1094 = call "Database.vi"("Maximum Row"=w2964, "Enum"=w2960, "Delete row?"=TRUE, "Data"=w2997, "Auto Increment ID?"=TRUE, "Table"="main_grading_group_disc_29", "Connection"="dsgs") -> ("Error out"=w2961:errorcluster)  [unwired: 4 in]
            n1095 = shared-variable ".\\Maintenance.lvlib\\error_39"(w2961) -> ()  [unwired: 1 in, 1 out]
          }
        }
        n1096 = shared-variable ".\\D04.lvlib\\SaveD04"(error in=w2915) -> (w2921:bool, error out=w2918:errorcluster)
        n1097 = Index Array(array=w2916, index (col)=3 ("disabled index (col)")) -> (element=w2924:dbl[])  [unwired: 1 in]
        n1098 = Boolean To (0,1)(Boolean=w2921) -> (0, 1=w2922:i16)
        n1099 = Build Array(w2922) -> (w2923:i16[])
        n1100 = call-poly <vilib>:"Basic Level Trigger Detection.vi"("signal in"=w2923, "level"=0.5, "error in (no error)"=w2918) -> ("trigger detected?"=w2926:bool, "error out"=w2917:errorcluster)  [unwired: 10 in, 1 out]
        n1101 = case shown="True" w2926 {
          selector: w2926 -> [_ w2955]
          tunnel: [FALSE w2955] -> w2925
          tunnel: w2924 -> [_ w2950]
          tunnel: w2917 -> [w2941 w2943]
          tunnel: [w2941 w2942] -> w2913
          frame False {
          }
          frame True {
            n1102 = Array To Spreadsheet String(array=w2950, 3:"%.2f" ("format string")) -> (spreadsheet string=w2954:string)  [unwired: 1 in]
            n1103 = Get Date/Time In Seconds() -> (seconds since 1Jan1904=w2951:timestamp)
            n1104 = Format Date/Time String(time format string (%c)="%H:%M:%S", seconds (now)=w2951) -> (date/time string=w2953:string)  [unwired: 1 in]
            n1105 = Format Date/Time String(time format string (%c)="%Y/%m/%d", seconds (now)=w2951) -> (date/time string=w2952:string)  [unwired: 1 in]
            n1106 = Bundle("date/time string"=w2952, "date/time string"=w2953, "disc 04", "spreadsheet string"=w2954) -> (w2945:T22)  [unwired: 1 in]
            n1107 = To Variant(anything=w2945) -> (Variant=w2944:variant)
            n1108 = call "Database.vi"("Delete row?"=FALSE, "Data"=w2944, "Error in"=w2943, "Auto Increment ID?"=TRUE, "Table"="thresholds_calibration_table", "Connection"="dsgs") -> ("Error out"=w2942:errorcluster)  [unwired: 5 in]
          }
        }
        n1109 = shared-variable ".\\D04.lvlib\\SaveD04Ok"(w2925) -> (error out=w2914:errorcluster)  [unwired: 1 in]
        n1110 = shared-variable ".\\Maintenance.lvlib\\error_45"(w2913) -> ()  [unwired: 1 in, 1 out]
      }
      frame #21 {
        n1111 = shared-variable ".\\D04.lvlib\\SaveD04"(FALSE ("SaveD29"), error in=w3024) -> (error out=w3023:errorcluster)
        n1112 = case shown="4" "speed disc 29" {
          tunnel: w3023 -> [w3041 w3043 w3059 w3075 w3091]
          tunnel: [w3041 w3042 w3058 w3074 w3090] -> w3026
          frame 0, Default {
          }
          frame 1 {
            n1113 = Get Date/Time In Seconds() -> (seconds since 1Jan1904=w3057:timestamp)
            n1114 = Format Date/Time String(time format string (%c)="%Y/%m/%d", seconds (now)=w3057) -> (date/time string=w3056:string)  [unwired: 1 in]
            n1115 = Format Date/Time String(time format string (%c)="%H:%M:%S", seconds (now)=w3057) -> (date/time string=w3055:string)  [unwired: 1 in]
            n1116 = Bundle("60001", "date/time string"=w3056, "date/time string"=w3055, "Speed signal is changed and applied in disc 29") -> (w3054:T11)  [unwired: 1 in]
            n1117 = To Variant(anything=w3054) -> (Variant=w3053:variant)
            n1118 = call "Database.vi"("Maximum Row"=u64 0 ("Storage Time (Day)"), "Delete row?"=FALSE, "Data"=w3053, "Error in"=w3043, "Auto Increment ID?"=TRUE, "Table"="log_table", "Connection"="dsgs") -> ("Error out"=w3042:errorcluster)  [unwired: 4 in]
          }
          frame 2 {
            n1119 = Get Date/Time In Seconds() -> (seconds since 1Jan1904=w3073:timestamp)
            n1120 = Format Date/Time String(time format string (%c)="%Y/%m/%d", seconds (now)=w3073) -> (date/time string=w3072:string)  [unwired: 1 in]
            n1121 = Format Date/Time String(time format string (%c)="%H:%M:%S", seconds (now)=w3073) -> (date/time string=w3071:string)  [unwired: 1 in]
            n1122 = Bundle("60002", "date/time string"=w3072, "date/time string"=w3071, "Speed signal is changed and applied in disc 29") -> (w3070:T11)  [unwired: 1 in]
            n1123 = To Variant(anything=w3070) -> (Variant=w3069:variant)
            n1124 = call "Database.vi"("Maximum Row"=u64 0 ("Storage Time (Day)"), "Delete row?"=FALSE, "Data"=w3069, "Error in"=w3059, "Auto Increment ID?"=TRUE, "Table"="log_table", "Connection"="dsgs") -> ("Error out"=w3058:errorcluster)  [unwired: 4 in]
          }
          frame 4 {
            n1125 = Get Date/Time In Seconds() -> (seconds since 1Jan1904=w3089:timestamp)
            n1126 = Format Date/Time String(time format string (%c)="%Y/%m/%d", seconds (now)=w3089) -> (date/time string=w3088:string)  [unwired: 1 in]
            n1127 = Format Date/Time String(time format string (%c)="%H:%M:%S", seconds (now)=w3089) -> (date/time string=w3087:string)  [unwired: 1 in]
            n1128 = Bundle("60003", "date/time string"=w3088, "date/time string"=w3087, "Speed signal is changed but not applied in disc 29") -> (w3086:T11)  [unwired: 1 in]
            n1129 = To Variant(anything=w3086) -> (Variant=w3085:variant)
            n1130 = call "Database.vi"("Maximum Row"=u64 0 ("Storage Time (Day)"), "Delete row?"=FALSE, "Data"=w3085, "Error in"=w3075, "Auto Increment ID?"=TRUE, "Table"="log_table", "Connection"="dsgs") -> ("Error out"=w3074:errorcluster)  [unwired: 4 in]
          }
          frame 8 {
            n1131 = Get Date/Time In Seconds() -> (seconds since 1Jan1904=w3105:timestamp)
            n1132 = Format Date/Time String(time format string (%c)="%Y/%m/%d", seconds (now)=w3105) -> (date/time string=w3104:string)  [unwired: 1 in]
            n1133 = Format Date/Time String(time format string (%c)="%H:%M:%S", seconds (now)=w3105) -> (date/time string=w3103:string)  [unwired: 1 in]
            n1134 = Bundle("60004", "date/time string"=w3104, "date/time string"=w3103, "Speed signal is changed but not applied in disc 29") -> (w3102:T11)  [unwired: 1 in]
            n1135 = To Variant(anything=w3102) -> (Variant=w3101:variant)
            n1136 = call "Database.vi"("Maximum Row"=u64 0 ("Storage Time (Day)"), "Delete row?"=FALSE, "Data"=w3101, "Error in"=w3091, "Auto Increment ID?"=TRUE, "Table"="log_table", "Connection"="dsgs") -> ("Error out"=w3090:errorcluster)  [unwired: 4 in]
          }
        }
        n1137 = shared-variable ".\\Maintenance.lvlib\\error_50"(w3026) -> ()  [unwired: 1 in, 1 out]
      }
      frame #22 {
        n1138 = shared-variable ".\\D05.lvlib\\LiveViewD05"() -> (w3121:refnum<image>, error out=w3120:errorcluster)  [unwired: 1 in]
        n1139 = shared-variable ".\\Setting Lib.lvlib\\processing file path"() -> (w3117:path, error out=w3113:errorcluster)  [unwired: 1 in]
        n1140 = shared-variable ".\\D05.lvlib\\GradingThrD05"() -> (w3112:dbl[], error out=w3111:errorcluster)  [unwired: 1 in]
        n1141 = call "IMAQ Copy"("error in (no error)"=w3120, "Image Dst"=w3122, "Image Src"=w3121) -> ("error out"=w3116:errorcluster, "Image Dst Out"=w3119:T7)  [unwired: 3 in]
        n1142 = property on="DISC 05" class="Bool (strict)"() -> ("Value"=w3110:bool)  [unwired: 2 in, 2 out]
        n1143 = call "find and draw circles.vi"("Image Src"=w3119, "module path"=w3117, "function name"="get_circels", "initialized array"=w3107, "Image Dst"=w3129, "error in (no error)"=w3113, "session in"=w3135, "Run/Stop"=w3110, "grading Thr"=w3112) -> ("session out"=w3134:refnum<k35>, "circle info"=w3132:dbl[][], "Image Out"=w3137:T7, "error out"=w3114:errorcluster, "pellet detected?"=w3118:bool)  [unwired: 6 in]
        n1144 = shared-variable ".\\Maintenance.lvlib\\error_21"(w3116) -> ()  [unwired: 1 in, 1 out]
        n1145 = shared-variable ".\\Maintenance.lvlib\\error_26"(w3114) -> ()  [unwired: 1 in, 1 out]
        n1146 = shared-variable ".\\D05.lvlib\\PelletDetectedD05"(w3137, error in=w3111) -> (error out=w3115:errorcluster)
      }
      frame #23 {
        n1147 = shared-variable ".\\Calibration Lib.lvlib\\calibration matrix D05"() -> (w3156:dbl[], error out=w3151:errorcluster)  [unwired: 1 in]
        n1148 = Matrix Size(0:w3147) -> (1:w3146:i32)  [unwired: 1 out]
        n1149 = property on="DISC 05" class="Bool (strict)"() -> ("Value"=w3144:bool)  [unwired: 2 in, 2 out]
        n1150 = Select(t=w3146, s=w3144, f=0) -> (s? t:f=w3145:i32)
        n1151 = shared-variable ".\\Calibration Lib.lvlib\\Method Selection"(error in=w3151) -> (w3157:enum32{"Method 1", "Method 2"}, error out=w3150:errorcluster)
        n1152 = shared-variable ".\\D05.lvlib\\number of pellet 05"(w3145) -> ()  [unwired: 1 in, 1 out]
        n1153 = case shown="\"Method 2\"" w3157 {
          tunnel: w3155 -> [w3168 w3171]
          tunnel: w3156 -> [_ w3177]
          tunnel: w3147 -> [w3170 w3176]
          tunnel: [w3170 w3174] -> w3153
          tunnel: w3138 -> [w3169 w3175]
          tunnel: [w3169 w3173] -> w3149
          tunnel: [w3168 w3171] -> w3154
          tunnel: w3150 -> [w3167 w3172]
          tunnel: [w3167 w3172] -> w3148
          frame "Method 1", Default {
          }
          frame "Method 2" {
            n1154 = call "pixel2milimetr.vi"("1*3 Transform Matrix"=w3177, "circle array"=w3176, "Error in"=w3175) -> ("calibrated circles"=w3174:dbl[][], "Error out"=w3173:errorcluster)  [unwired: 11 in]
          }
        }
        n1155 = shared-variable ".\\Maintenance.lvlib\\error_31"(w3149, error in=w3148) -> ()  [unwired: 1 out]
      }
      frame #24 {
        n1156 = case shown="True" w3183 {
          tunnel: w3197 -> [_ w3265]
          tunnel: w3196 -> [w3202 w3260]
          tunnel: [w3202 w3259] -> w3195
          tunnel: w3194 -> [w3203 w3255]
          tunnel: [w3203 w3253] -> w3193
          tunnel: w3192 -> [w3201 w3250]
          tunnel: [w3201 w3249] -> w3191
          tunnel: [dbl[] [0.0, 0.0, 0.0, 0.0, 0.0, 0.0, 0.0, 0.0] w3211] -> w3184
          tunnel: [errorcluster {"status"=FALSE, "code"=0, "source"=""} ("error IO") w3234] -> w3182
          frame False {
          }
          frame True {
            w3231 = dbl[] [250.047, 512.0, 1000.0, 1953.125, 2744.0, 4096.0, 5832.0]  # fixed threshoulds
            n1157 = shared-variable ".\\D05.lvlib\\GradingThrD05"() -> (w3239:dbl[], error out=w3236:errorcluster)  [unwired: 1 in]
            n1158 = Index Array(array=w3265, index (col)=2 ("disabled index (col)")) -> (element=w3252:dbl[])  [unwired: 1 in]
            n1159 = property on="avg grading array size" class="DigNum (strict)"() -> ("Value"=w3243:i32)  [unwired: 2 in, 2 out]
            n1160 = shared-variable ".\\Calibration Lib.lvlib\\Method Selection"(error in=w3236) -> (w3240:enum32{"Method 1", "Method 2"}, error out=w3235:errorcluster)
            n1161 = property on="live grading array size" class="DigNum (strict)"() -> ("Value"=w3244:i32)  [unwired: 2 in, 2 out]
            n1162 = Array Size(array=w3252) -> (size(s)=w3254:i32)
            n1163 = Subtract(x=w3244, y=w3254) -> (x-y=w3263:i32)
            n1164 = Subtract(x=w3243, y=w3254) -> (x-y=w3258:i32)
            n1165 = Multiply(x=w3231, y=0.25) -> (x*y=w3232:dbl[])
            n1166 = Equal?(x=w3240, y=enum32{"Method 1", "Method 2"}."Method 1" ("Method Selection")) -> (x = y?=w3241:bool)
            n1167 = call "array managment.vi"("2D array in"=w3260, "col sel"=4, "cir num"=w3254, "index"=w3263, "subarray"=w3252) -> ("2D array out"=w3259:dbl[][], "1D array out"=w3261:dbl[])  [unwired: 13 in]
            n1168 = call "array managment.vi"("2D array in"=w3255, "col sel"=4, "cir num"=w3254, "index"=w3258, "subarray"=w3252) -> ("2D array out"=w3253:dbl[][], "1D array out"=w3256:dbl[])  [unwired: 13 in]
            n1169 = Select(t=w3239, s=w3241, f=w3232) -> (s? t:f=w3238:dbl[])
            n1170 = property on="DISC 05" class="Bool (strict)"() -> ("Value"=w3226:bool)  [unwired: 2 in, 2 out]
            n1171 = property on="DISC 05" class="Bool (strict)"() -> ("Value"=w3225:bool)  [unwired: 2 in, 2 out]
            n1172 = call "pelletpercents.vi"("Run/Stop"=w3226, "grading threshoulds"=w3238, "Sorted data"=w3261) -> ("Percentage"=w3245:dbl[])  [unwired: 8 in]
            n1173 = call "pelletpercents.vi"("Run/Stop"=w3225, "grading threshoulds"=w3238, "Sorted data"=w3256) -> ("Percentage"=w3228:dbl[])  [unwired: 8 in]
            n1174 = Number To Fractional String(number=w3245, precision (6)=i16 2) -> (F-format string=w3246:string[])  [unwired: 2 in]
            n1175 = Number To Fractional String(number=w3228, precision (6)=i16 2) -> (F-format string=w3230:string[])  [unwired: 2 in]
            n1176 = Fract/Exp String To Number(string=w3246) -> (number=w3211:dbl[])  [unwired: 3 in, 1 out]
            n1177 = property on="DISC 05" class="Bool (strict)"() -> ("Value"=w3208:bool)  [unwired: 2 in, 2 out]
            n1178 = Fract/Exp String To Number(string=w3230) -> (number=w3227:dbl[])  [unwired: 3 in, 1 out]
            n1179 = call "grading average.vi"("input array"=w3211) -> ("avg"=w3207:dbl)  [unwired: 10 in]
            "AVG 05" <- w3207
            n1180 = shared-variable ".\\D05.lvlib\\AvgResultD05"(w3227, error in=w3235) -> (error out=w3237:errorcluster)
            n1181 = Not A Number/Path/Refnum?(number/path/refnum=w3207) -> (NaN/Path/Refnum?=w3205:bool)
            n1182 = Not(x=w3205) -> (.not. x?=w3204:bool)
            n1183 = Index Array(array=w3211, index #1=2 ("index")) -> (element #1=w3224:dbl, element #2=w3221:dbl, element #3=w3222:dbl, element #4=w3223:dbl)  [unwired: 3 in]
            n1184 = And(x=w3208, y=w3204) -> (x .and. y?=w3206:bool)
            n1185 = Add(x=w3224, y=w3221) -> (x+y=w3213:dbl)
            "8-12.5 05" <- w3213
            n1186 = Add(x=w3222, y=w3223) -> (x+y=w3214:dbl)
            "12.5-16 05" <- w3214
            n1187 = Add(x=w3221, y=w3222) -> (x+y=w3216:dbl)
            "10-14 05" <- w3216
            n1188 = shared-variable ".\\D05.lvlib\\LiveResultD05"(w3211, error in=w3237) -> (error out=w3234:errorcluster)
            n1189 = Add(x=w3214, y=w3213) -> (x+y=→"8-16mm 05":dbl)
            n1190 = Select(t=w3207, s=w3206, f=12.0) -> (s? t:f=w3209:dbl)
            n1191 = call "dif array management.vi"("2D array in"=w3250, "col sel"=4, "new element/subarray"=w3209) -> ("2D array out"=w3249:dbl[][])  [unwired: 15 in, 1 out]
            n1192 = Greater Or Equal?(x=w3216, y=70.0) -> (x >= y?=w3219:bool)
            n1193 = Select(t=u32 65282 ("Fill Color"), s=w3219, f=u32 4018019 ("Fill Color")) -> (s? t:f=w3215:u32)
            n1194 = property on="10-14 05" class="Slide (strict)"("Fill Color"=w3215) -> ()  [unwired: 2 in, 2 out]
          }
        }
      }
      frame #25 {
        n1195 = case shown="True" w3285 {
          tunnel: w3284 -> [_ w3319]
          frame False {
          }
          frame True {
            w3314 = enum16{"ID Delete", "Time Delete"}."Time Delete" ("Enum")
            n1196 = property on="projector 05" class="Bool (strict)"() -> ("Value"=w3349:bool)  [unwired: 2 in, 2 out]
            n1197 = Select(t="ON" ("time format string (%c)"), s=w3349, f="OFF" ("time format string (%c)")) -> (s? t:f=w3350:string)
            n1198 = property on="cam 05" class="Bool (strict)"() -> ("Value"=w3347:bool)  [unwired: 2 in, 2 out]
            n1199 = Select(t="ON" ("time format string (%c)"), s=w3347, f="OFF" ("time format string (%c)")) -> (s? t:f=w3348:string)
            n1200 = property on="AUTO/MAN 05" class="Bool (strict)"() -> ("Value"=w3345:bool)  [unwired: 2 in, 2 out]
            n1201 = Select(t="Auto", s=w3345, f="Manual") -> (s? t:f=w3346:string)
            n1202 = property on="DISC 05" class="Bool (strict)"() -> ("Value"=w3343:bool)  [unwired: 2 in, 2 out]
            n1203 = Select(t="Run", s=w3343, f="Stop") -> (s? t:f=w3344:string)
            n1204 = Get Date/Time In Seconds() -> (seconds since 1Jan1904=w3340:timestamp)
            n1205 = Format Date/Time String(time format string (%c)="%Y/%m/%d", seconds (now)=w3340) -> (date/time string=w3341:string)  [unwired: 1 in]
            n1206 = Format Date/Time String(time format string (%c)="%H:%M:%S", seconds (now)=w3340) -> (date/time string=w3342:string)  [unwired: 1 in]
            n1207 = Index Array(array=w3319, index #1=0 ("index")) -> (element #1=w3332:dbl, element #2=w3333:dbl, element #3=w3334:dbl, element #4=w3335:dbl, element #5=w3336:dbl, element #6=w3337:dbl, element #7=w3338:dbl, element #8=w3339:dbl)  [unwired: 7 in]
            n1208 = Bundle("date/time string"=w3341, "date/time string"=w3342, w3332, w3333, w3334, w3335, w3336, w3337, w3338, w3339, "f"=w3344, "f"=w3346, "time format string (%c)"=w3348, "time format string (%c)"=w3350) -> (w3320:T20)  [unwired: 1 in]
            n1209 = shared-variable ".\\Setting Lib.lvlib\\database refresh period"() -> (w3318:i32, error out=w3317:errorcluster)  [unwired: 1 in]
            n1210 = Unbundle(w3320) -> ("date/time string"=w3364:string, "date/time string"=w3363:string, w3362:dbl, w3359:dbl, w3358:dbl, w3361:dbl, "f"=w3356:string, "f"=w3355:string, "time format string (%c)"=w3354:string, "time format string (%c)"=w3353:string)  [unwired: 4 out]
            n1211 = Add(x=w3359, y=w3358) -> (x+y=w3357:dbl)
            n1212 = Compound Arithmetic op=ADD(w3362, w3359, w3358, w3361) -> (w3360:dbl)
            n1213 = To Variant(anything=w3320) -> (Variant=w3365:variant)
            n1214 = call "Database.vi"("Maximum Row"=w3318, "Enum"=w3314, "Delete row?"=TRUE, "Data"=w3365, "Error in"=w3317, "Auto Increment ID?"=TRUE, "Table"="grading_disc_30", "Connection"="dsgs") -> ("Error out"=w3315:errorcluster)  [unwired: 3 in]
            n1215 = Bundle("date/time string"=w3364, "date/time string"=w3363, w3360, w3357, "f"=w3356, "f"=w3355, "time format string (%c)"=w3354, "time format string (%c)"=w3353) -> (w3352:T21)  [unwired: 1 in]
            n1216 = shared-variable ".\\Maintenance.lvlib\\error_40"(w3315) -> ()  [unwired: 1 in, 1 out]
            n1217 = To Variant(anything=w3352) -> (Variant=w3351:variant)
            n1218 = call "Database.vi"("Maximum Row"=w3318, "Enum"=w3314, "Delete row?"=TRUE, "Data"=w3351, "Auto Increment ID?"=TRUE, "Table"="main_grading_group_disc_30", "Connection"="dsgs") -> ("Error out"=w3316:errorcluster)  [unwired: 4 in]
            n1219 = shared-variable ".\\Maintenance.lvlib\\error_41"(w3316) -> ()  [unwired: 1 in, 1 out]
          }
        }
        n1220 = shared-variable ".\\D05.lvlib\\SaveD05"(error in=w3272) -> (w3278:bool, error out=w3275:errorcluster)
        n1221 = Index Array(array=w3273, index (col)=4 ("disabled index (col)")) -> (element=w3281:dbl[])  [unwired: 1 in]
        n1222 = Boolean To (0,1)(Boolean=w3278) -> (0, 1=w3279:i16)
        n1223 = Build Array(w3279) -> (w3280:i16[])
        n1224 = call-poly <vilib>:"Basic Level Trigger Detection.vi"("signal in"=w3280, "level"=0.5, "error in (no error)"=w3275) -> ("trigger detected?"=w3283:bool, "error out"=w3274:errorcluster)  [unwired: 10 in, 1 out]
        n1225 = case shown="True" w3283 {
          selector: w3283 -> [_ w3309]
          tunnel: [FALSE w3309] -> w3282
          tunnel: w3281 -> [_ w3304]
          tunnel: w3274 -> [w3295 w3297]
          tunnel: [w3295 w3296] -> w3270
          frame False {
          }
          frame True {
            n1226 = Array To Spreadsheet String(array=w3304, 3:"%.2f" ("format string")) -> (spreadsheet string=w3308:string)  [unwired: 1 in]
            n1227 = Get Date/Time In Seconds() -> (seconds since 1Jan1904=w3305:timestamp)
            n1228 = Format Date/Time String(time format string (%c)="%H:%M:%S", seconds (now)=w3305) -> (date/time string=w3307:string)  [unwired: 1 in]
            n1229 = Format Date/Time String(time format string (%c)="%Y/%m/%d", seconds (now)=w3305) -> (date/time string=w3306:string)  [unwired: 1 in]
            n1230 = Bundle("date/time string"=w3306, "date/time string"=w3307, "disc 05", "spreadsheet string"=w3308) -> (w3299:T22)  [unwired: 1 in]
            n1231 = To Variant(anything=w3299) -> (Variant=w3298:variant)
            n1232 = call "Database.vi"("Delete row?"=FALSE, "Data"=w3298, "Error in"=w3297, "Auto Increment ID?"=TRUE, "Table"="thresholds_calibration_table", "Connection"="dsgs") -> ("Error out"=w3296:errorcluster)  [unwired: 5 in]
          }
        }
        n1233 = shared-variable ".\\D05.lvlib\\SaveD05Ok"(w3282, error in=w3270) -> (error out=w3271:errorcluster)
        n1234 = shared-variable ".\\Maintenance.lvlib\\error_46"(w3270) -> ()  [unwired: 1 in, 1 out]
      }
      frame #26 {
        n1235 = shared-variable ".\\D05.lvlib\\SaveD05"(FALSE ("SaveD30"), error in=w3379) -> (error out=w3378:errorcluster)
        n1236 = case shown="8" "speed disc 30" {
          tunnel: w3378 -> [w3392 w3394 w3410 w3426 w3442]
          tunnel: [w3392 w3393 w3409 w3425 w3441] -> w3381
          frame 0, Default {
          }
          frame 1 {
            n1237 = Get Date/Time In Seconds() -> (seconds since 1Jan1904=w3408:timestamp)
            n1238 = Format Date/Time String(time format string (%c)="%Y/%m/%d", seconds (now)=w3408) -> (date/time string=w3407:string)  [unwired: 1 in]
            n1239 = Format Date/Time String(time format string (%c)="%H:%M:%S", seconds (now)=w3408) -> (date/time string=w3406:string)  [unwired: 1 in]
            n1240 = Bundle("60001", "date/time string"=w3407, "date/time string"=w3406, "Speed signal is changed and applied in disc 30") -> (w3405:T11)  [unwired: 1 in]
            n1241 = To Variant(anything=w3405) -> (Variant=w3404:variant)
            n1242 = call "Database.vi"("Maximum Row"=u64 0 ("Storage Time (Day)"), "Delete row?"=FALSE, "Data"=w3404, "Error in"=w3394, "Auto Increment ID?"=TRUE, "Table"="log_table", "Connection"="dsgs") -> ("Error out"=w3393:errorcluster)  [unwired: 4 in]
          }
          frame 2 {
            n1243 = Get Date/Time In Seconds() -> (seconds since 1Jan1904=w3424:timestamp)
            n1244 = Format Date/Time String(time format string (%c)="%Y/%m/%d", seconds (now)=w3424) -> (date/time string=w3423:string)  [unwired: 1 in]
            n1245 = Format Date/Time String(time format string (%c)="%H:%M:%S", seconds (now)=w3424) -> (date/time string=w3422:string)  [unwired: 1 in]
            n1246 = Bundle("60002", "date/time string"=w3423, "date/time string"=w3422, "Speed signal is changed and applied in disc 30") -> (w3421:T11)  [unwired: 1 in]
            n1247 = To Variant(anything=w3421) -> (Variant=w3420:variant)
            n1248 = call "Database.vi"("Maximum Row"=u64 0 ("Storage Time (Day)"), "Delete row?"=FALSE, "Data"=w3420, "Error in"=w3410, "Auto Increment ID?"=TRUE, "Table"="log_table", "Connection"="dsgs") -> ("Error out"=w3409:errorcluster)  [unwired: 4 in]
          }
          frame 4 {
            n1249 = Get Date/Time In Seconds() -> (seconds since 1Jan1904=w3440:timestamp)
            n1250 = Format Date/Time String(time format string (%c)="%Y/%m/%d", seconds (now)=w3440) -> (date/time string=w3439:string)  [unwired: 1 in]
            n1251 = Format Date/Time String(time format string (%c)="%H:%M:%S", seconds (now)=w3440) -> (date/time string=w3438:string)  [unwired: 1 in]
            n1252 = Bundle("60003", "date/time string"=w3439, "date/time string"=w3438, "Speed signal is changed but not applied in disc 30") -> (w3437:T11)  [unwired: 1 in]
            n1253 = To Variant(anything=w3437) -> (Variant=w3436:variant)
            n1254 = call "Database.vi"("Maximum Row"=u64 0 ("Storage Time (Day)"), "Delete row?"=FALSE, "Data"=w3436, "Error in"=w3426, "Auto Increment ID?"=TRUE, "Table"="log_table", "Connection"="dsgs") -> ("Error out"=w3425:errorcluster)  [unwired: 4 in]
          }
          frame 8 {
            n1255 = Get Date/Time In Seconds() -> (seconds since 1Jan1904=w3455:timestamp)
            n1256 = Format Date/Time String(time format string (%c)="%Y/%m/%d", seconds (now)=w3455) -> (date/time string=w3454:string)  [unwired: 1 in]
            n1257 = Format Date/Time String(time format string (%c)="%H:%M:%S", seconds (now)=w3455) -> (date/time string=w3453:string)  [unwired: 1 in]
            n1258 = Bundle("60004", "date/time string"=w3454, "date/time string"=w3453, "Speed signal is changed but not applied in disc 30") -> (w3452:T11)  [unwired: 1 in]
            n1259 = To Variant(anything=w3452) -> (Variant=w3451:variant)
            n1260 = call "Database.vi"("Delete row?"=FALSE, "Data"=w3451, "Error in"=w3442, "Auto Increment ID?"=TRUE, "Table"="log_table", "Connection"="dsgs") -> ("Error out"=w3441:errorcluster)  [unwired: 5 in]
          }
        }
        n1261 = shared-variable ".\\Maintenance.lvlib\\error_51"(w3381) -> ()  [unwired: 1 in, 1 out]
      }
      frame #27 {
        n1262 = shared-variable ".\\D06.lvlib\\LiveViewD06"() -> (w3466:refnum<image>, error out=w3467:errorcluster)  [unwired: 1 in]
        n1263 = shared-variable ".\\Setting Lib.lvlib\\processing file path"() -> (w3469:path, error out=w3472:errorcluster)  [unwired: 1 in]
        n1264 = shared-variable ".\\D06.lvlib\\GradingThrD06"() -> (w3473:dbl[], error out=w3474:errorcluster)  [unwired: 1 in]
        n1265 = call "IMAQ Copy"("error in (no error)"=w3467, "Image Dst"=w3463, "Image Src"=w3466) -> ("error out"=w3470:errorcluster, "Image Dst Out"=w3468:T7)  [unwired: 3 in]
        n1266 = property on="DISC 06" class="Bool (strict)"() -> ("Value"=w3460:bool)  [unwired: 2 in, 2 out]
        n1267 = call "find and draw circles.vi"("Image Src"=w3468, "module path"=w3469, "function name"="get_circels", "initialized array"=w3461, "Image Dst"=w3462, "error in (no error)"=w3472, "Run/Stop"=w3460, "grading Thr"=w3473) -> ("session out"=w3458:refnum<k35>, "circle info"=w3459:dbl[][], "Image Out"=w3464:T7, "error out"=w3471:errorcluster, "pellet detected?"=w3457:bool)  [unwired: 7 in]
        n1268 = shared-variable ".\\Maintenance.lvlib\\error_21"(w3470) -> ()  [unwired: 1 in, 1 out]
        n1269 = shared-variable ".\\Maintenance.lvlib\\error_26"(w3471) -> ()  [unwired: 1 in, 1 out]
        n1270 = shared-variable ".\\D06.lvlib\\PelletDetectedD06"(w3464, error in=w3474) -> ()  [unwired: 1 out]
      }
      frame #28 {
        n1271 = shared-variable ".\\Calibration Lib.lvlib\\calibration matrix D06"() -> (w3499:dbl[], error out=w3497:errorcluster)  [unwired: 1 in]
        n1272 = shared-variable ".\\Calibration Lib.lvlib\\calibration factor D06"() -> (w3498:sgl, error out=w3496:errorcluster)  [unwired: 1 in]
        n1273 = Matrix Size(0:w3488) -> (1:w3492:i32)  [unwired: 1 out]
        n1274 = Select(t=w3492, s=w3489, f=0) -> (s? t:f=w3491:i32)
        n1275 = shared-variable ".\\Calibration Lib.lvlib\\Method Selection"(error in=w3497) -> (w3500:enum32{"Method 1", "Method 2"}, error out=w3495:errorcluster)
        n1276 = shared-variable ".\\D05.lvlib\\number of pellet 05"(w3491) -> ()  [unwired: 1 in, 1 out]
        n1277 = case shown="\"Method 2\"" w3500 {
          tunnel: w3487 -> [w3511 w3515]
          tunnel: w3499 -> [_ w3520]
          tunnel: w3498 -> [_ _]
          tunnel: w3488 -> [w3513 w3519]
          tunnel: [w3513 w3517] -> w3486
          tunnel: w3496 -> [w3512 w3518]
          tunnel: [w3512 w3516] -> w3494
          tunnel: [w3511 w3515] -> _
          tunnel: w3495 -> [w3510 w3514]
          tunnel: [w3510 w3514] -> w3493
          frame "Method 1", Default {
          }
          frame "Method 2" {
            n1278 = call "pixel2milimetr.vi"("1*3 Transform Matrix"=w3520, "circle array"=w3519, "Error in"=w3518) -> ("calibrated circles"=w3517:dbl[][], "Error out"=w3516:errorcluster)  [unwired: 11 in]
          }
        }
        n1279 = shared-variable ".\\Maintenance.lvlib\\error_31"(w3494, error in=w3493) -> ()  [unwired: 1 out]
      }
      frame #29 {
        n1280 = case shown="True" w3522 {
          tunnel: w3525 -> [_ w3602]
          tunnel: w3527 -> [w3539 w3597]
          tunnel: [w3539 w3596] -> w3526
          tunnel: w3524 -> [w3540 w3592]
          tunnel: [w3540 w3590] -> w3523
          tunnel: w3529 -> [w3538 w3549]
          tunnel: [w3538 w3587] -> w3528
          tunnel: [dbl[] [0.0, 0.0, 0.0, 0.0, 0.0, 0.0, 0.0, 0.0] w3555] -> _
          tunnel: [errorcluster {"status"=FALSE, "code"=0, "source"=""} ("error IO") w3574] -> _
          frame False {
          }
          frame True {
            w3571 = dbl[] [250.047, 512.0, 1000.0, 1953.125, 2744.0, 4096.0, 5832.0]  # fixed threshoulds
            n1281 = shared-variable ".\\D05.lvlib\\GradingThrD05"() -> (w3579:dbl[], error out=w3576:errorcluster)  [unwired: 1 in]
            n1282 = property on="avg grading array size" class="DigNum (strict)"() -> ("Value"=w3547:i32)  [unwired: 2 in, 2 out]
            n1283 = property on="live grading array size" class="DigNum (strict)"() -> ("Value"=w3548:i32)  [unwired: 2 in, 2 out]
            n1284 = Index Array(array=w3602, index (col)=2 ("disabled index (col)")) -> (element=w3589:dbl[])  [unwired: 1 in]
            n1285 = shared-variable ".\\Calibration Lib.lvlib\\Method Selection"(error in=w3576) -> (w3580:enum32{"Method 1", "Method 2"}, error out=w3575:errorcluster)
            n1286 = Array Size(array=w3589) -> (size(s)=w3591:i32)
            n1287 = Subtract(x=w3548, y=w3591) -> (x-y=w3600:i32)
            n1288 = Subtract(x=w3547, y=w3591) -> (x-y=w3595:i32)
            n1289 = Multiply(x=w3571, y=0.25) -> (x*y=w3572:dbl[])
            n1290 = Equal?(x=w3580, y=enum32{"Method 1", "Method 2"}."Method 1" ("Method Selection")) -> (x = y?=w3581:bool)
            n1291 = call "array managment.vi"("2D array in"=w3597, "col sel"=4, "cir num"=w3591, "index"=w3600, "subarray"=w3589) -> ("2D array out"=w3596:dbl[][], "1D array out"=w3598:dbl[])  [unwired: 13 in]
            n1292 = call "array managment.vi"("2D array in"=w3592, "col sel"=4, "cir num"=w3591, "index"=w3595, "subarray"=w3589) -> ("2D array out"=w3590:dbl[][], "1D array out"=w3593:dbl[])  [unwired: 13 in]
            n1293 = Select(t=w3579, s=w3581, f=w3572) -> (s? t:f=w3578:dbl[])
            n1294 = property on="DISC 06" class="Bool (strict)"() -> ("Value"=w3546:bool)  [unwired: 2 in, 2 out]
            n1295 = property on="DISC 06" class="Bool (strict)"() -> ("Value"=w3545:bool)  [unwired: 2 in, 2 out]
            n1296 = call "pelletpercents.vi"("Run/Stop"=w3546, "grading threshoulds"=w3578, "Sorted data"=w3598) -> ("Percentage"=w3583:dbl[])  [unwired: 8 in]
            n1297 = call "pelletpercents.vi"("Run/Stop"=w3545, "grading threshoulds"=w3578, "Sorted data"=w3593) -> ("Percentage"=w3568:dbl[])  [unwired: 8 in]
            n1298 = Number To Fractional String(number=w3583, precision (6)=i16 2) -> (F-format string=w3584:string[])  [unwired: 2 in]
            n1299 = Number To Fractional String(number=w3568, precision (6)=i16 2) -> (F-format string=w3570:string[])  [unwired: 2 in]
            n1300 = property on="DISC 06" class="Bool (strict)"() -> ("Value"=w3544:bool)  [unwired: 2 in, 2 out]
            n1301 = Fract/Exp String To Number(string=w3584) -> (number=w3555:dbl[])  [unwired: 3 in, 1 out]
            n1302 = Fract/Exp String To Number(string=w3570) -> (number=w3567:dbl[])  [unwired: 3 in, 1 out]
            n1303 = call "grading average.vi"("input array"=w3555) -> ("avg"=w3541:dbl)  [unwired: 10 in]
            "AVG 06" <- w3541
            n1304 = shared-variable ".\\D05.lvlib\\AvgResultD05"(w3567, error in=w3575) -> (error out=w3577:errorcluster)
            n1305 = Not A Number/Path/Refnum?(number/path/refnum=w3541) -> (NaN/Path/Refnum?=w3551:bool)
            n1306 = Not(x=w3551) -> (.not. x?=w3550:bool)
            n1307 = Index Array(array=w3555, index #1=2 ("index")) -> (element #1=w3566:dbl, element #2=w3563:dbl, element #3=w3564:dbl, element #4=w3565:dbl)  [unwired: 3 in]
            n1308 = And(x=w3544, y=w3550) -> (x .and. y?=w3552:bool)
            n1309 = Add(x=w3566, y=w3563) -> (x+y=w3543:dbl)
            "8-12.5 06" <- w3543
            n1310 = Add(x=w3564, y=w3565) -> (x+y=w3542:dbl)
            "12.5-16 06" <- w3542
            n1311 = Add(x=w3563, y=w3564) -> (x+y=w3558:dbl)
            "10-14 6" <- w3558
            n1312 = shared-variable ".\\D05.lvlib\\LiveResultD05"(w3555, error in=w3577) -> (error out=w3574:errorcluster)
            n1313 = Add(x=w3542, y=w3543) -> (x+y=→"8-16mm 6":dbl)
            n1314 = Select(t=w3541, s=w3552, f=12.0) -> (s? t:f=w3553:dbl)
            n1315 = call "dif array management.vi"("2D array in"=w3549, "col sel"=5, "new element/subarray"=w3553) -> ("2D array out"=w3587:dbl[][])  [unwired: 15 in, 1 out]
            n1316 = Greater Or Equal?(x=w3558, y=70.0) -> (x >= y?=w3561:bool)
            n1317 = Select(t=u32 65282 ("Fill Color"), s=w3561, f=u32 4018019 ("Fill Color")) -> (s? t:f=w3557:u32)
            n1318 = property on="10-14 6" class="Slide (strict)"("Fill Color"=w3557) -> ()  [unwired: 2 in, 2 out]
          }
        }
      }
      frame #30 {
      }
      frame #31 {
        n1319 = shared-variable ".\\D05.lvlib\\LiveResultD05"() -> (w3674:dbl[])  [unwired: 1 in, 1 out]
        n1320 = shared-variable ".\\D04.lvlib\\LiveResultD04"() -> (w3681:dbl[])  [unwired: 1 in, 1 out]
        n1321 = shared-variable ".\\D03.lvlib\\LiveResultD03"() -> (w3678:dbl[])  [unwired: 1 in, 1 out]
        n1322 = shared-variable ".\\D02.lvlib\\LiveResultD02"() -> (w3686:dbl[])  [unwired: 1 in, 1 out]
        n1323 = shared-variable ".\\D01.lvlib\\liveResultArray"() -> (w3689:dbl[])  [unwired: 1 in, 1 out]
        n1324 = shared-variable ".\\D05.lvlib\\LiveResultD05"() -> (w3669:dbl[])  [unwired: 1 in, 1 out]
        n1325 = shared-variable ".\\D04.lvlib\\LiveResultD04"() -> (w3662:dbl[])  [unwired: 1 in, 1 out]
        n1326 = shared-variable ".\\D03.lvlib\\LiveResultD03"() -> (w3665:dbl[])  [unwired: 1 in, 1 out]
        n1327 = shared-variable ".\\D02.lvlib\\LiveResultD02"() -> (w3657:dbl[])  [unwired: 1 in, 1 out]
        n1328 = shared-variable ".\\D01.lvlib\\liveResultArray"() -> (w3654:dbl[])  [unwired: 1 in, 1 out]
        n1329 = property on="AVG 04" class="DigNum (strict)"() -> ("Value"=w3624:dbl)  [unwired: 2 in, 2 out]
        n1330 = property on="AVG 02" class="DigNum (strict)"() -> ("Value"=w3626:dbl)  [unwired: 2 in, 2 out]
        n1331 = property on="AVG 03" class="DigNum (strict)"() -> ("Value"=w3625:dbl)  [unwired: 2 in, 2 out]
        n1332 = property on="AVG 05" class="DigNum (strict)"() -> ("Value"=w3623:dbl)  [unwired: 2 in, 2 out]
        n1333 = property on="AVG 01" class="DigNum (strict)"() -> ("Value"=w3627:dbl)  [unwired: 2 in, 2 out]
        n1334 = property on="10-14 01" class="Slide (strict)"() -> ("Value"=w3706:dbl)  [unwired: 2 in, 2 out]
        n1335 = property on="10-14 02" class="Slide (strict)"() -> ("Value"=w3705:dbl)  [unwired: 2 in, 2 out]
        n1336 = property on="10-14 03" class="Slide (strict)"() -> ("Value"=w3704:dbl)  [unwired: 2 in, 2 out]
        n1337 = property on="10-14 04" class="Slide (strict)"() -> ("Value"=w3703:dbl)  [unwired: 2 in, 2 out]
        n1338 = property on="10-14 05" class="Slide (strict)"() -> ("Value"=w3702:dbl)  [unwired: 2 in, 2 out]
        n1339 = property on="12.5-16 01" class="Slide (strict)"() -> ("Value"=w3723:dbl)  [unwired: 2 in, 2 out]
        n1340 = property on="12.5-16 02" class="Slide (strict)"() -> ("Value"=w3722:dbl)  [unwired: 2 in, 2 out]
        n1341 = property on="12.5-16 03" class="Slide (strict)"() -> ("Value"=w3721:dbl)  [unwired: 2 in, 2 out]
        n1342 = property on="12.5-16 04" class="Slide (strict)"() -> ("Value"=w3720:dbl)  [unwired: 2 in, 2 out]
        n1343 = property on="12.5-16 05" class="Slide (strict)"() -> ("Value"=w3719:dbl)  [unwired: 2 in, 2 out]
        n1344 = property on="8-12.5 01" class="Slide (strict)"() -> ("Value"=w3736:dbl)  [unwired: 2 in, 2 out]
        n1345 = property on="8-12.5 02" class="Slide (strict)"() -> ("Value"=w3735:dbl)  [unwired: 2 in, 2 out]
        n1346 = property on="8-12.5 03" class="Slide (strict)"() -> ("Value"=w3734:dbl)  [unwired: 2 in, 2 out]
        n1347 = property on="8-12.5 04" class="Slide (strict)"() -> ("Value"=w3733:dbl)  [unwired: 2 in, 2 out]
        n1348 = property on="8-12.5 05" class="Slide (strict)"() -> ("Value"=w3732:dbl)  [unwired: 2 in, 2 out]
        n1349 = property on="DISC 01" class="Bool (strict)"() -> ("Value"=w3741:bool)  [unwired: 2 in, 2 out]
        n1350 = property on="DISC 02" class="Bool (strict)"() -> ("Value"=w3739:bool)  [unwired: 2 in, 2 out]
        n1351 = property on="DISC 03" class="Bool (strict)"() -> ("Value"=w3738:bool)  [unwired: 2 in, 2 out]
        n1352 = property on="DISC 04" class="Bool (strict)"() -> ("Value"=w3737:bool)  [unwired: 2 in, 2 out]
        n1353 = property on="DISC 05" class="Bool (strict)"() -> ("Value"=w3740:bool)  [unwired: 2 in, 2 out]
        n1354 = Index Array(array=w3674, index #1=0 ("index")) -> (element #1=w3673:dbl, element #2=w3672:dbl)  [unwired: 1 in]
        n1355 = Index Array(array=w3681, index #1=0 ("index")) -> (element #1=w3682:dbl, element #2=w3683:dbl)  [unwired: 1 in]
        n1356 = Index Array(array=w3678, index #1=0 ("index")) -> (element #1=w3677:dbl, element #2=w3676:dbl)  [unwired: 1 in]
        n1357 = Index Array(array=w3686, index #1=0 ("index")) -> (element #1=w3685:dbl, element #2=w3684:dbl)  [unwired: 1 in]
        n1358 = Index Array(array=w3689, index #1=0 ("index")) -> (element #1=w3690:dbl, element #2=w3691:dbl)  [unwired: 1 in]
        n1359 = Index Array(array=w3669, index #1=6 ("index")) -> (element #1=w3670:dbl, element #2=w3671:dbl)  [unwired: 1 in]
        n1360 = Index Array(array=w3662, index #1=6 ("index")) -> (element #1=w3661:dbl, element #2=w3660:dbl)  [unwired: 1 in]
        n1361 = Index Array(array=w3665, index #1=6 ("index")) -> (element #1=w3666:dbl, element #2=w3667:dbl)  [unwired: 1 in]
        n1362 = Index Array(array=w3657, index #1=6 ("index")) -> (element #1=w3658:dbl, element #2=w3659:dbl)  [unwired: 1 in]
        n1363 = Index Array(array=w3654, index #1=6 ("index")) -> (element #1=w3653:dbl, element #2=w3652:dbl)  [unwired: 1 in]
        n1364 = Boolean To (0,1)(Boolean=w3741) -> (0, 1=w3618:i16)
        n1365 = Boolean To (0,1)(Boolean=w3739) -> (0, 1=w3617:i16)
        n1366 = Boolean To (0,1)(Boolean=w3738) -> (0, 1=w3616:i16)
        n1367 = Boolean To (0,1)(Boolean=w3737) -> (0, 1=w3615:i16)
        n1368 = Boolean To (0,1)(Boolean=w3740) -> (0, 1=w3614:i16)
        n1369 = Add(x=w3673, y=w3672) -> (x+y=w3646:dbl)
        n1370 = Add(x=w3682, y=w3683) -> (x+y=w3645:dbl)
        n1371 = Add(x=w3677, y=w3676) -> (x+y=w3644:dbl)
        n1372 = Add(x=w3685, y=w3684) -> (x+y=w3643:dbl)
        n1373 = Add(x=w3690, y=w3691) -> (x+y=w3642:dbl)
        n1374 = Add(x=w3670, y=w3671) -> (x+y=w3651:dbl)
        n1375 = Add(x=w3661, y=w3660) -> (x+y=w3650:dbl)
        n1376 = Add(x=w3666, y=w3667) -> (x+y=w3649:dbl)
        n1377 = Add(x=w3658, y=w3659) -> (x+y=w3648:dbl)
        n1378 = Add(x=w3653, y=w3652) -> (x+y=w3647:dbl)
        n1379 = shared-variable ".\\control setting.lvlib\\Error2DArray"(w3619) -> ()  [unwired: 1 in, 1 out]
        n1380 = Multiply(x=w3706, y=w3618) -> (x*y=w3708:dbl)
        n1381 = Multiply(x=w3705, y=w3617) -> (x*y=w3711:dbl)
        n1382 = Multiply(x=w3704, y=w3616) -> (x*y=w3707:dbl)
        n1383 = Multiply(x=w3703, y=w3615) -> (x*y=w3710:dbl)
        n1384 = Multiply(x=w3702, y=w3614) -> (x*y=w3709:dbl)
        n1385 = Compound Arithmetic op=ADD(w3618, w3617, w3616, w3615, w3614) -> (w3730:i16)
        n1386 = Multiply(x=w3651, y=w3614) -> (x*y=w3636:dbl)
        n1387 = Multiply(x=w3650, y=w3615) -> (x*y=w3635:dbl)
        n1388 = Multiply(x=w3649, y=w3616) -> (x*y=w3634:dbl)
        n1389 = Multiply(x=w3648, y=w3617) -> (x*y=w3633:dbl)
        n1390 = Multiply(x=w3647, y=w3618) -> (x*y=w3632:dbl)
        n1391 = Multiply(x=w3646, y=w3614) -> (x*y=w3641:dbl)
        n1392 = Multiply(x=w3645, y=w3615) -> (x*y=w3640:dbl)
        n1393 = Multiply(x=w3644, y=w3616) -> (x*y=w3639:dbl)
        n1394 = Multiply(x=w3643, y=w3617) -> (x*y=w3638:dbl)
        n1395 = Multiply(x=w3642, y=w3618) -> (x*y=w3637:dbl)
        n1396 = Compound Arithmetic op=ADD(w3627, w3626, w3625, w3624, w3623) -> (w3622:dbl)
        n1397 = Multiply(x=w3723, y=w3618) -> (x*y=w3717:dbl)
        n1398 = Multiply(x=w3722, y=w3617) -> (x*y=w3714:dbl)
        n1399 = Multiply(x=w3721, y=w3616) -> (x*y=w3718:dbl)
        n1400 = Multiply(x=w3720, y=w3615) -> (x*y=w3715:dbl)
        n1401 = Multiply(x=w3719, y=w3614) -> (x*y=w3716:dbl)
        n1402 = Multiply(x=w3736, y=w3618) -> (x*y=w3726:dbl)
        n1403 = Multiply(x=w3735, y=w3617) -> (x*y=w3727:dbl)
        n1404 = Multiply(x=w3734, y=w3616) -> (x*y=w3728:dbl)
        n1405 = Multiply(x=w3733, y=w3615) -> (x*y=w3724:dbl)
        n1406 = Multiply(x=w3732, y=w3614) -> (x*y=w3725:dbl)
        n1407 = Equal To 0?(x=w3730) -> (x = 0?=w3731:bool)
        n1408 = Compound Arithmetic op=ADD(w3641, w3640, w3639, w3638, w3637) -> (w3631:dbl)
        n1409 = Compound Arithmetic op=ADD(w3636, w3635, w3634, w3633, w3632) -> (w3630:dbl)
        n1410 = Compound Arithmetic op=ADD(w3708, w3711, w3707, w3710, w3709) -> (w3701:dbl)
        n1411 = Select(t=i16 1, s=w3731, f=w3730) -> (s? t:f=w3621:i16)
        n1412 = Compound Arithmetic op=ADD(w3717, w3714, w3718, w3715, w3716) -> (w3712:dbl)
        n1413 = Compound Arithmetic op=ADD(w3726, w3727, w3728, w3724, w3725) -> (w3713:dbl)
        n1414 = Divide(x=w3712, y=w3621) -> (x/y=w3694:dbl)
        "12.5-16 total" <- w3694
        n1415 = Divide(x=w3713, y=w3621) -> (x/y=w3693:dbl)
        "8-12.5 total" <- w3693
        n1416 = Divide(x=w3631, y=w3621) -> (x/y=→"Under Size":dbl)
        n1417 = Divide(x=w3630, y=w3621) -> (x/y=→"Over Size":dbl)
        n1418 = Divide(x=w3701, y=w3621) -> (x/y=w3696:dbl)
        "10-14 total" <- w3696
        n1419 = Divide(x=w3622, y=w3621) -> (x/y=→"AVG":dbl)
        n1420 = Add(x=w3694, y=w3693) -> (x+y=→"8-16mm total":dbl)
        n1421 = Greater Or Equal?(x=w3696, y=70.0) -> (x >= y?=w3699:bool)
        n1422 = Select(t=u32 65282 ("Fill Color"), s=w3699, f=u32 4018019 ("Fill Color")) -> (s? t:f=w3695:u32)
        n1423 = property on="10-14 total" class="Slide (strict)"("Fill Color"=w3695) -> ()  [unwired: 2 in, 2 out]
        "2D array out" <- w3619
      }
    }
  }
  n1424 = call "maintenance.vi"() -> ()  [unwired: 12 in]
  n1425 = call "report.vi"() -> ()  [unwired: 12 in]
  n1426 = call "DetectedPelletPage.vi"() -> ()  [unwired: 12 in]
  n1427 = call "setting.vi"() -> ()  [unwired: 12 in]
  n1428 = call "live view D01.vi"() -> ()  [unwired: 16 in]
  n1429 = call "live view D02.vi"() -> ()  [unwired: 16 in]
  n1430 = call "live view D03.vi"() -> ()  [unwired: 16 in]
  n1431 = call "live view D04.vi"() -> ()  [unwired: 16 in]
  n1432 = call "live view D05.vi"() -> ()  [unwired: 16 in]
  n1433 = call "live view D06.vi"() -> ()  [unwired: 16 in]
  n1434 = call "TrendsD26.vi"() -> ()  [unwired: 12 in]
  n1435 = call "TrendsD27.vi"() -> ()  [unwired: 12 in]
  n1436 = call "TrendsD03.vi"() -> ()  [unwired: 12 in]
  n1437 = call "TrendsD04.vi"() -> ()  [unwired: 12 in]
  n1438 = call "TrendsD05.vi"() -> ()  [unwired: 12 in]
  n1439 = call "Login.vi"() -> ()  [unwired: 12 in]
  n1440 = property on="Login" class="Bool (strict)"("Value"=TRUE ("Login")) -> ()  [unwired: 2 in, 2 out]
  n1441 = disable-structure shown="Disabled" {
    disable-tunnel: [w3752 _] -> w29
    disable-tunnel: [w3751 _] -> w28
    frame Disabled {
      n1442 = call-poly <userlib>:"DAQNavi Create Channel.vi"("physical channels"="PCI-1710,BID#0/port0:1") -> ("task out"=w3752:i32, "error out"=w3751:errorcluster)  [unwired: 13 in]
    }
    frame Enabled {
    }
  }
  n1443 = Initialize Array(i8 0 ("element"), 24 ("dimension size")) -> (w55:i8[])
  n1444 = Close Python Session(session in=w97) -> (11:w34:errorcluster)  [unwired: 1 in]
  n1445 = for {
    tunnel: w55 -> [w3756] mode=indexing
    tunnel: [w3753] -> w30 mode=indexing
    i -> [w3755]
    n1446 = Increment(x=w3755) -> (x+1=w3754:i32)
    n1447 = Add(x=w3756, y=w3754) -> (x+y=w3753:i32)
  }
  n1448 = shared-variable ".\\Maintenance.lvlib\\error_52"(w34) -> ()  [unwired: 1 in, 1 out]
  n1449 = call <vilib>:"FL Load Fuzzy System.vi"("error in (no error)"=errorcluster {"status"=FALSE, "code"=0, "source"=""}, "file path"=path "D:/DSGS projector/software/fuzzy2.fs") -> ("error out"=w31:errorcluster, "fuzzy system out"=w32:T23)  [unwired: 8 in]
  n1450 = Initialize Array(0.0 ("element"), 2 ("dimension size")) -> (w24:dbl[])
  n1451 = Initialize Array(0.0 ("element"), 2 ("dimension size")) -> (w12:dbl[])
  n1452 = Initialize Array(i16 0 ("element"), 35 ("dimension size")) -> (w9:i16[])
  n1453 = Initialize Array(0.0 ("element"), 2 ("dimension size")) -> (w15:dbl[])
  n1454 = Initialize Array(0.0 ("element"), 2 ("dimension size")) -> (w21:dbl[])
  n1455 = Initialize Array(0.0 ("element"), 2 ("dimension size")) -> (w18:dbl[])
  n1456 = while {
    tunnel: w32 -> [w3786]
    tunnel: w31 -> [w3790]
    tunnel: w30 -> [w3785]
    tunnel: w29 -> [w3811]
    tunnel: w28 -> [w3810]
    shift-right: [w3784] -> _
    shift-left: w24 -> [w3797]
    shift-right: [w3760] -> _
    shift-left: w21 -> [w3794]
    shift-right: [w3761] -> _
    shift-left: w18 -> [w3792]
    shift-right: [w3762] -> _
    shift-left: w15 -> [w3789]
    shift-right: [w3763] -> _
    shift-left: w12 -> [w3787]
    tunnel: w9 -> [w3759]
    tunnel: string[] [] ("rules as text") -> [w3758]
    stop <- FALSE stop-if-true
    # "Control Loop"
    n1457 = property on="AUTO/MAN 01" class="Bool (strict)"() -> ("Value"=w3806:bool)  [unwired: 2 in, 2 out]
    n1458 = property on="DISC 01" class="Bool (strict)"() -> ("Value"=w3805:bool)  [unwired: 2 in, 2 out]
    n1459 = property on="AUTO/MAN 03" class="Bool (strict)"() -> ("Value"=w3802:bool)  [unwired: 2 in, 2 out]
    n1460 = And(x=w3806, y=w3805) -> (x .and. y?=w3796:bool)
    n1461 = property on="DISC 04" class="Bool (strict)"() -> ("Value"=w3800:bool)  [unwired: 2 in, 2 out]
    n1462 = property on="DISC 03" class="Bool (strict)"() -> ("Value"=w3757:bool)  [unwired: 2 in, 2 out]
    n1463 = case shown="True" w3796 {
      tunnel: w3786 -> [_ w4587]
      tunnel: w3790 -> [w4556 w4586]
      tunnel: [w4556 w4582] -> w3781
      tunnel: [w4556 w4582] -> w3780
      tunnel: [FALSE ("t") w4585] -> w3783
      tunnel: [FALSE ("t") w4584] -> w3782
      tunnel: w3797 -> [w4553 w4580]
      tunnel: [w4553 w4579] -> w3784
      tunnel: w3785 -> [_ w4563]
      tunnel: w3759 -> [_ w4561]
      tunnel: w3758 -> [_ w4557]
      frame False {
      }
      frame True {
        n1464 = flat-sequence {
          tunnel: w4580 -> [w4615]
          tunnel: w4587 -> [w4616]
          tunnel: w4586 -> [w4617]
          tunnel: w4563 -> [w4618]
          tunnel: [w4618] -> w4576
          tunnel: [w4617] -> w4575
          tunnel: [w4616] -> w4574
          tunnel: [w4615] -> w4573
          tunnel: [w4594] -> w4564
          tunnel: [w4593] -> w4562
          tunnel: w4561 -> [w4593]
          tunnel: [w4592] -> w4558
          tunnel: w4557 -> [w4592]
          tunnel: [w4624] -> w4572
          tunnel: [w4644] -> w4571
          tunnel: [w4637] -> w4570
          tunnel: [w4636] -> w4569
          tunnel: [w4635] -> w4568
          tunnel: [w4634] -> w4567
          tunnel: [w4629] -> w4566
          tunnel: w4576 -> [w4635]
          tunnel: w4575 -> [w4639]
          tunnel: w4574 -> [w4644]
          tunnel: w4573 -> [w4634]
          tunnel: [w4624] -> w4565
          tunnel: w4564 -> [w4622]
          tunnel: w4562 -> [w4621]
          tunnel: [w4621] -> w4560
          tunnel: [w4620] -> w4559
          tunnel: w4558 -> [w4620]
          tunnel: [w4651] -> w4591
          tunnel: [w4655] -> w4590
          tunnel: [w4652] -> w4581
          tunnel: [w4649] -> w4577
          tunnel: w4565 -> [_]
          tunnel: w4566 -> [w4647]
          tunnel: w4567 -> [w4650]
          tunnel: w4568 -> [w4648]
          tunnel: w4569 -> [w4651]
          tunnel: w4570 -> [w4654]
          tunnel: w4571 -> [w4653]
          tunnel: w4572 -> [w4656]
          tunnel: w4560 -> [w4646]
          tunnel: w4559 -> [w4645]
          tunnel: w4591 -> [w4720]
          tunnel: w4590 -> [w4713]
          tunnel: [w4718] -> w4589
          tunnel: [w4717] -> w4588
          tunnel: [w4716] -> w4583
          tunnel: w4581 -> [w4715]
          tunnel: [w4714] -> w4578
          tunnel: w4577 -> [w4714]
          tunnel: w4589 -> [w4747]
          tunnel: w4588 -> [w4748]
          tunnel: [w4742] -> w4585
          tunnel: [w4739] -> w4584
          tunnel: [w4745] -> w4582
          tunnel: w4583 -> [w4745]
          tunnel: [w4738] -> w4579
          tunnel: w4578 -> [w4738]
          frame #0 {
            n1465 = shared-variable ".\\control setting.lvlib\\SetPoints"() -> (w4607:dbl[])  [unwired: 1 in, 1 out]
            n1466 = property on="2D array out" class="Arr (strict)"() -> ("Value"=w4614:dbl[][])  [unwired: 2 in, 2 out]
            n1467 = Index Array(array=w4614, index (row)=0, index (col)=0 ("disabled index (col)")) -> (element=w4609:dbl)
            n1468 = Index Array(array=w4607, index=0) -> (element=w4606:dbl)
            n1469 = Subtract(x=w4609, y=w4606) -> (x-y=w4605:dbl)
            n1470 = property on="speed  min 01" class="Bool (strict)"() -> ("Value"=w4598:bool)  [unwired: 2 in, 2 out]
            n1471 = property on="speed max 01" class="Bool (strict)"() -> ("Value"=w4601:bool)  [unwired: 2 in, 2 out]
            n1472 = Absolute Value(x=w4605) -> (abs(x)=w4611:dbl)
            n1473 = Less Than 0?(x=w4605) -> (x < 0?=w4602:bool)
            n1474 = Greater Than 0?(x=w4605) -> (x > 0?=w4597:bool)
            n1475 = property on="no change D01" class="Bool (strict)"() -> ("Value"=w4604:bool)  [unwired: 2 in, 2 out]
            n1476 = Not And(1:w4601, 2:w4602) -> (0:w4599:bool)
            n1477 = Not And(1:w4598, 2:w4597) -> (0:w4595:bool)
            n1478 = Greater?(x=w4611, y=1.0) -> (0:w4603:bool)
            n1479 = And(x=w4604, y=w4603) -> (x .and. y?=w4600:bool)
            n1480 = And(x=w4600, y=w4599) -> (x .and. y?=w4596:bool)
            n1481 = And(x=w4596, y=w4595) -> (x .and. y?=w4594:bool)
            "sudden change D01" <- w4594
          }
          frame #1 {
            w4630 = u16 0 items=["Falling Edge", "Rising Edge"] ("trigger slope")
            # "D26 Tick count to reach the pulse time (defult : 5min)"
            n1482 = Boolean To (0,1)(Boolean=w4622) -> (0, 1=w4625:i16)
            n1483 = Build Array(w4625) -> (w4626:i16[])
            n1484 = call-poly <vilib>:"Basic Level Trigger Detection.vi"("signal in"=w4626, "level"=0.5) -> ("trigger detected?"=w4619:bool)  [unwired: 11 in, 2 out]
            n1485 = shared-variable ".\\control setting.lvlib\\PlsePeriod"() -> (w4628:i16)  [unwired: 1 in, 1 out]
            n1486 = call "Elapsed Time"("Time Target (s)"=w4628, "Reset"=w4619, "error in (no error)"=w4639) -> ("Elapsed Time (s)"=w4623:dbl, "error out"=w4638:errorcluster)  [unwired: 9 in, 6 out]
            n1487 = In Range and Coerce(upper limit=10.0, x=w4623, lower limit=0.1) -> (In Range?=w4636:bool)  [unwired: 1 out]
            n1488 = Boolean To (0,1)(Boolean=w4636) -> (0, 1=w4631:i16)
            n1489 = Build Array(w4631) -> (w4632:i16[])
            n1490 = Build Array(w4631) -> (w4643:i16[])
            n1491 = call-poly <vilib>:"Basic Level Trigger Detection.vi"("signal in"=w4632, "level"=0.5, "trigger slope"=w4630) -> ("trigger detected?"=w4629:bool)  [unwired: 10 in, 2 out]
            n1492 = call-poly <vilib>:"Basic Level Trigger Detection.vi"("signal in"=w4643, "level"=0.5, "error in (no error)"=w4638) -> ("trigger detected?"=w4624:bool, "error out"=w4637:errorcluster)  [unwired: 10 in, 1 out]
          }
          frame #2 {
            # "calculate the pulse width by fuzzy controler"
            n1493 = case shown="True" w4647 {
              tunnel: w4650 -> [w4657 w4665]
              tunnel: [w4657 w4660] -> w4649
              frame False {
              }
              frame True {
                n1494 = Delete From Array(array=w4665, index=1) -> (array with subset deleted=w4663:dbl[])  [unwired: 1 in, 1 out]
                n1495 = property on="SPEED 01" class="DigNum (strict)"() -> ("Value"=w4661:dbl)  [unwired: 2 in, 2 out]
                n1496 = Insert Into Array(array=w4663, index=0, new element=w4661) -> (w4660:dbl[])
                n1497 = Index Array(array=w4660, index #1=0 ("index")) -> (element #2=→"previous speed D01":dbl)  [unwired: 1 in, 1 out]
              }
            }
            n1498 = case shown="True" w4656 {
              tunnel: w4653 -> [_ w4703]
              tunnel: [w4667 w4674] -> w4655
              tunnel: w4654 -> [w4666 w4701]
              tunnel: [w4666 w4699] -> w4652
              tunnel: w4648 -> [_ w4687]
              tunnel: w4646 -> [_ w4680]
              tunnel: w4645 -> [_ w4678]
              frame False {
                n1499 = property on="puls width D01" class="DigNum (strict)"() -> ("Value"=w4667:dbl)  [unwired: 2 in, 2 out]
              }
              frame True {
                n1500 = property on="2D array out" class="Arr (strict)"(error in=w4701) -> (error out=w4700:errorcluster, "Value"=w4691:dbl[][])  [unwired: 1 in, 1 out]
                n1501 = shared-variable ".\\control setting.lvlib\\SetPoints"() -> (w4694:dbl[])  [unwired: 1 in, 1 out]
                n1502 = Index Array(array=w4691, index (row)=0 ("disabled index (row)"), index (col)=0 ("disabled index (col)")) -> (element=w4697:dbl)
                n1503 = Index Array(array=w4691, index (col)=0 ("disabled index (col)")) -> (element=w4689:dbl[])  [unwired: 1 in]
                n1504 = Reverse 1D Array(array=w4689) -> (reversed array=w4688:dbl[])
                n1505 = Index Array(array=w4694, index=0) -> (element=w4692:dbl)
                n1506 = call <vilib>:"Linear Fit.vi"("Y"=w4688, "X"=w4687) -> ("slope"=w4684:dbl)  [unwired: 9 in, 4 out]
                n1507 = Subtract(x=w4697, y=w4692) -> (x-y=w4685:dbl)
                "last error 01" <- w4685
                n1508 = Multiply(x=w4684, y=24.0) -> (x*y=w4682:dbl)
                "slope D01" <- w4682
                n1509 = Build Array(w4685, w4682) -> (w4686:dbl[])
                n1510 = call-poly <vilib>:"FL Fuzzy Controller.vi"("error in (no error)"=w4700, "input values"=w4686, "fuzzy system in"=w4703) -> ("error out"=w4699:errorcluster, "rule weights"=w4679:dbl[], "output value"=w4696:dbl, "fuzzy system out"=w4681:T23)  [unwired: 4 in, 1 out]
                n1511 = Divide(x=w4696, y=0.25) -> (x/y=w4676:dbl)
                n1512 = property on="speed  min 01" class="Bool (strict)"() -> ("Value"=w4672:bool)  [unwired: 2 in, 2 out]
                n1513 = Round To Nearest(number=w4676) -> (nearest integer value=w4668:dbl)
                n1514 = property on="speed max 01" class="Bool (strict)"() -> ("Value"=w4673:bool)  [unwired: 2 in, 2 out]
                n1515 = Multiply(x=w4668, y=1.2) -> (x*y=w4674:dbl)
                "puls width D01" <- w4674
                n1516 = call "rules update.vi"("fuzzy system in"=w4681, "Array in"=w4680, "rule weights 2"=w4679, "rules as text"=w4678) -> ("rules as text out"=→"rules as text out":string[])  [unwired: 15 in]
                n1517 = call "change situation.vi"("pulse width"=w4668, "speed max"=w4673, "speed min"=w4672) -> ("no change"=→"no change D01":bool, "increas"=→"increase D01":bool, "decreas"=→"decrease D01":bool)  [unwired: 14 in]
              }
            }
          }
          frame #3 {
            # "create pulse width by Timer"
            n1518 = Absolute Value(x=w4713) -> (abs(x)=w4719:dbl)
            n1519 = local read "previous speed D01"() -> (w4707:dbl)
            n1520 = local read "sudden change D01"() -> (w4709:bool)
            n1521 = local read "last error 01"() -> (w4708:dbl)
            n1522 = local read "no change D01"() -> (w4710:bool)
            n1523 = local read "decrease D01"() -> (w4712:bool)
            n1524 = case shown="True" w4720 {
              selector: w4720 -> [_ w4734]
              tunnel: [FALSE w4728] -> w4718
              tunnel: w4719 -> [_ w4727]
              tunnel: [w4721 w4724] -> w4716
              tunnel: w4715 -> [w4721 w4723]
              frame False {
              }
              frame True {
                w4726 = 1.0 ("lower limit")
                n1525 = Boolean To (0,1)(Boolean=w4734) -> (0, 1=w4733:i16)
                n1526 = Build Array(w4733) -> (w4732:i16[])
                n1527 = call-poly <vilib>:"Basic Level Trigger Detection.vi"("signal in"=w4732, "level"=0.5) -> ("trigger detected?"=w4730:bool)  [unwired: 11 in, 2 out]
                n1528 = call "Elapsed Time2"("Time Target (s)"=9.0, "Reset"=w4730, "error in (no error)"=w4723) -> ("Elapsed Time (s)"=w4729:dbl, "error out"=w4724:errorcluster)  [unwired: 9 in, 6 out]
                "Elapsed Time (s) 2" <- w4729
                n1529 = Add(x=w4727, y=w4726) -> (x+y=w4725:dbl)
                n1530 = In Range and Coerce(upper limit=w4725, x=w4729, lower limit=w4726) -> (In Range?=w4728:bool)  [unwired: 1 out]
              }
            }
            n1531 = local read "increase D01"() -> (w4711:bool)
            n1532 = local read "puls width D01"() -> (w4706:dbl)
            n1533 = local read "slope D01"() -> (w4705:dbl)
            n1534 = Less Than 0?(x=w4713) -> (x < 0?=w4717:bool)
            n1535 = Bundle("decrease D01"=w4712, "increase D01"=w4711, "no change D01"=w4710, "sudden change D01"=w4709, "last error 01"=w4708, "previous speed D01"=w4707, "puls width D01"=w4706, "slope D01"=w4705) -> (w4704:T35)  [unwired: 1 in]
            n1536 = shared-variable ".\\control setting.lvlib\\ControlInfoD01"(w4704) -> ()  [unwired: 1 in, 1 out]
          }
          frame #4 {
            # "incrise"
            n1537 = property on="speed  min 01" class="Bool (strict)"() -> ("Value"=w4736:bool)  [unwired: 2 in, 2 out]
            n1538 = Select(t=FALSE, s=w4748, f=w4747) -> (s? t:f=w4743:bool)
            n1539 = Select(t=w4747, s=w4748, f=FALSE ("t")) -> (s? t:f=w4740:bool)
            n1540 = property on="speed max 01" class="Bool (strict)"() -> ("Value"=w4737:bool)  [unwired: 2 in, 2 out]
            n1541 = Select(t=FALSE, s=w4737, f=w4743) -> (s? t:f=w4742:bool)
            n1542 = Select(t=FALSE, s=w4736, f=w4740) -> (s? t:f=w4739:bool)
          }
        }
      }
    }
    n1543 = property on="AUTO/MAN 04" class="Bool (strict)"() -> ("Value"=w3801:bool)  [unwired: 2 in, 2 out]
    n1544 = property on="DISC 02" class="Bool (strict)"() -> ("Value"=w3803:bool)  [unwired: 2 in, 2 out]
    n1545 = property on="AUTO/MAN 05" class="Bool (strict)"() -> ("Value"=w3799:bool)  [unwired: 2 in, 2 out]
    n1546 = property on="AUTO/MAN 02" class="Bool (strict)"() -> ("Value"=w3804:bool)  [unwired: 2 in, 2 out]
    n1547 = property on="DISC 05" class="Bool (strict)"() -> ("Value"=w3798:bool)  [unwired: 2 in, 2 out]
    n1548 = And(x=w3801, y=w3800) -> (x .and. y?=w3791:bool)
    n1549 = And(x=w3804, y=w3803) -> (x .and. y?=w3795:bool)
    n1550 = And(x=w3802, y=w3757) -> (x .and. y?=w3793:bool)
    n1551 = And(x=w3799, y=w3798) -> (x .and. y?=w3788:bool)
    n1552 = case shown="True" w3788 {
      tunnel: w3786 -> [_ w3850]
      tunnel: w3790 -> [w3831 w3849]
      tunnel: [w3831 w3845] -> w3765
      tunnel: [w3831 w3845] -> w3764
      tunnel: [FALSE ("t") w3848] -> w3767
      tunnel: [FALSE ("t") w3847] -> w3766
      tunnel: w3787 -> [w3828 w3838]
      tunnel: [w3828 w3834] -> w3763
      tunnel: w3785 -> [_ w3833]
      frame False {
      }
      frame True {
        n1553 = flat-sequence {
          tunnel: w3850 -> [w3882]
          tunnel: w3849 -> [w3883]
          tunnel: w3833 -> [w3884]
          tunnel: [w3884] -> w3843
          tunnel: [w3883] -> w3842
          tunnel: [w3882] -> w3841
          tunnel: [w3862] -> w3840
          tunnel: [w3861] -> w3839
          tunnel: w3838 -> [w3861]
          tunnel: [w3902] -> w3859
          tunnel: [w3909] -> w3858
          tunnel: [w3899] -> w3857
          tunnel: [w3887] -> w3856
          tunnel: [w3898] -> w3855
          tunnel: w3843 -> [w3898]
          tunnel: w3842 -> [w3901]
          tunnel: w3841 -> [w3909]
          tunnel: w3840 -> [w3893]
          tunnel: w3839 -> [w3891]
          tunnel: [w3891] -> w3837
          tunnel: [w3886] -> w3832
          tunnel: w3859 -> [w3919]
          tunnel: w3858 -> [w3915]
          tunnel: w3857 -> [w3916]
          tunnel: [w3918] -> w3854
          tunnel: w3856 -> [w3918]
          tunnel: [w3917] -> w3853
          tunnel: w3855 -> [w3914]
          tunnel: [w3913] -> w3844
          tunnel: w3837 -> [w3912]
          tunnel: [w3911] -> w3835
          tunnel: w3832 -> [w3910]
          tunnel: w3854 -> [w3978]
          tunnel: w3853 -> [w3975]
          tunnel: [w3976] -> w3852
          tunnel: [w3974] -> w3851
          tunnel: [w3973] -> w3846
          tunnel: w3844 -> [w3972]
          tunnel: [w3971] -> w3836
          tunnel: w3835 -> [w3971]
          tunnel: w3852 -> [w4005]
          tunnel: w3851 -> [w4006]
          tunnel: [w3999] -> w3848
          tunnel: [w3997] -> w3847
          tunnel: [w4003] -> w3845
          tunnel: w3846 -> [w4003]
          tunnel: [w3994] -> w3834
          tunnel: w3836 -> [w3994]
          frame #0 {
            n1554 = shared-variable ".\\control setting.lvlib\\SetPoints"() -> (w3874:dbl[])  [unwired: 1 in, 1 out]
            n1555 = property on="2D array out" class="Arr (strict)"() -> ("Value"=w3881:dbl[][])  [unwired: 2 in, 2 out]
            n1556 = Index Array(array=w3874, index=4) -> (element=w3873:dbl)
            n1557 = Index Array(array=w3881, index (row)=0, index (col)=4 ("disabled index (col)")) -> (element=w3876:dbl)
            n1558 = property on="no change D05" class="Bool (strict)"() -> ("Value"=w3860:bool)  [unwired: 2 in, 2 out]
            n1559 = Subtract(x=w3876, y=w3873) -> (x-y=w3872:dbl)
            n1560 = property on="speed  min 05" class="Bool (strict)"() -> ("Value"=w3866:bool)  [unwired: 2 in, 2 out]
            n1561 = property on="speed max 05" class="Bool (strict)"() -> ("Value"=w3869:bool)  [unwired: 2 in, 2 out]
            n1562 = Absolute Value(x=w3872) -> (abs(x)=w3878:dbl)
            n1563 = Less Than 0?(x=w3872) -> (x < 0?=w3870:bool)
            n1564 = Greater Than 0?(x=w3872) -> (x > 0?=w3865:bool)
            n1565 = Not And(1:w3869, 2:w3870) -> (0:w3867:bool)
            n1566 = Not And(1:w3866, 2:w3865) -> (0:w3863:bool)
            n1567 = Greater?(x=w3878, y=1.0) -> (0:w3871:bool)
            n1568 = And(x=w3860, y=w3871) -> (x .and. y?=w3868:bool)
            n1569 = And(x=w3868, y=w3867) -> (x .and. y?=w3864:bool)
            n1570 = And(x=w3864, y=w3863) -> (x .and. y?=w3862:bool)
            "sudden change D05" <- w3862
          }
          frame #1 {
            w3885 = u16 0 items=["Falling Edge", "Rising Edge"] ("trigger slope")
            # "D30 Tick count to reach the pulse time (defult : 5min)"
            n1571 = Boolean To (0,1)(Boolean=w3893) -> (0, 1=w3894:i16)
            n1572 = Build Array(w3894) -> (w3895:i16[])
            n1573 = shared-variable ".\\control setting.lvlib\\PlsePeriod"() -> (w3897:i16)  [unwired: 1 in, 1 out]
            n1574 = call-poly <vilib>:"Basic Level Trigger Detection.vi"("signal in"=w3895, "level"=0.5) -> ("trigger detected?"=w3892:bool)  [unwired: 11 in, 2 out]
            n1575 = call "Elapsed Time9"("Time Target (s)"=w3897, "Reset"=w3892, "error in (no error)"=w3901) -> ("Elapsed Time (s)"=w3905:dbl, "error out"=w3900:errorcluster)  [unwired: 9 in, 6 out]
            n1576 = In Range and Coerce(upper limit=10.0, x=w3905, lower limit=0.1) -> (In Range?=w3887:bool)  [unwired: 1 out]
            n1577 = Boolean To (0,1)(Boolean=w3887) -> (0, 1=w3908:i16)
            n1578 = Boolean To (0,1)(Boolean=w3887) -> (0, 1=w3888:i16)
            n1579 = Build Array(w3908) -> (w3907:i16[])
            n1580 = Build Array(w3888) -> (w3889:i16[])
            n1581 = call-poly <vilib>:"Basic Level Trigger Detection.vi"("signal in"=w3907, "level"=0.5, "error in (no error)"=w3900) -> ("trigger detected?"=w3902:bool, "error out"=w3899:errorcluster)  [unwired: 10 in, 1 out]
            n1582 = call-poly <vilib>:"Basic Level Trigger Detection.vi"("signal in"=w3889, "level"=0.5, "trigger slope"=w3885) -> ("trigger detected?"=w3886:bool)  [unwired: 10 in, 2 out]
          }
          frame #2 {
            # "calculate the pulse width by fuzzy controler"
            n1583 = case shown="True" w3919 {
              tunnel: w3915 -> [_ w3961]
              tunnel: [w3930 w3951] -> w3917
              tunnel: w3914 -> [_ w3941]
              tunnel: w3916 -> [w3929 w3959]
              tunnel: [w3929 w3957] -> w3913
              frame False {
                n1584 = property on="output value 5" class="DigNum (strict)"() -> ("Value"=w3930:dbl)  [unwired: 2 in, 2 out]
              }
              frame True {
                n1585 = property on="2D array out" class="Arr (strict)"(error in=w3959) -> (error out=w3958:errorcluster, "Value"=w3943:dbl[][])  [unwired: 1 in, 1 out]
                n1586 = shared-variable ".\\control setting.lvlib\\SetPoints"() -> (w3949:dbl[])  [unwired: 1 in, 1 out]
                n1587 = Index Array(array=w3943, index (row)=0 ("disabled index (row)"), index (col)=4 ("disabled index (col)")) -> (element=w3956:dbl)
                n1588 = Index Array(array=w3943, index (col)=4 ("disabled index (col)")) -> (element=w3946:dbl[])  [unwired: 1 in]
                n1589 = Reverse 1D Array(array=w3946) -> (reversed array=w3945:dbl[])
                n1590 = Index Array(array=w3949, index=4) -> (element=w3948:dbl)
                n1591 = Subtract(x=w3956, y=w3948) -> (x-y=w3937:dbl)
                "last error 05" <- w3937
                n1592 = call <vilib>:"Linear Fit.vi"("Y"=w3945, "X"=w3941) -> ("slope"=w3940:dbl)  [unwired: 9 in, 4 out]
                n1593 = Multiply(x=w3940, y=24.0) -> (x*y=w3938:dbl)
                "slope D05" <- w3938
                n1594 = Build Array(w3937, w3938) -> (w3942:dbl[])
                n1595 = call-poly <vilib>:"FL Fuzzy Controller.vi"("error in (no error)"=w3958, "input values"=w3942, "fuzzy system in"=w3961) -> ("error out"=w3957:errorcluster, "output value"=w3954:dbl)  [unwired: 4 in, 3 out]
                n1596 = property on="speed  min 05" class="Bool (strict)"() -> ("Value"=w3934:bool)  [unwired: 2 in, 2 out]
                n1597 = property on="speed max 05" class="Bool (strict)"() -> ("Value"=w3935:bool)  [unwired: 2 in, 2 out]
                n1598 = Divide(x=w3954, y=0.25) -> (x/y=w3947:dbl)
                n1599 = Round To Nearest(number=w3947) -> (nearest integer value=w3936:dbl)
                n1600 = Multiply(x=w3936, y=1.2) -> (x*y=w3951:dbl)
                "pulse width D05" <- w3951
                n1601 = call "change situation.vi"("pulse width"=w3936, "speed max"=w3935, "speed min"=w3934) -> ("no change"=→"no change D05":bool, "increas"=→"increase D05":bool, "decreas"=→"decrease D05":bool)  [unwired: 14 in]
              }
            }
            n1602 = case shown="True" w3910 {
              tunnel: w3912 -> [w3920 w3928]
              tunnel: [w3920 w3924] -> w3911
              frame False {
              }
              frame True {
                n1603 = Delete From Array(array=w3928, index=1) -> (array with subset deleted=w3926:dbl[])  [unwired: 1 in, 1 out]
                n1604 = property on="SPEED 05" class="DigNum (strict)"() -> ("Value"=w3921:dbl)  [unwired: 2 in, 2 out]
                n1605 = Insert Into Array(array=w3926, index=0, new element=w3921) -> (w3924:dbl[])
                n1606 = Index Array(array=w3924, index #1=0 ("index")) -> (element #2=→"previouse speed D05":dbl)  [unwired: 1 in, 1 out]
              }
            }
          }
          frame #3 {
            # "create pulse width by Timer"
            n1607 = Absolute Value(x=w3975) -> (abs(x)=w3977:dbl)
            n1608 = case shown="True" w3978 {
              selector: w3978 -> [_ w3992]
              tunnel: [FALSE w3986] -> w3976
              tunnel: w3977 -> [_ w3985]
              tunnel: [w3979 w3982] -> w3973
              tunnel: w3972 -> [w3979 w3981]
              frame False {
              }
              frame True {
                w3984 = 1.0 ("lower limit")
                n1609 = Boolean To (0,1)(Boolean=w3992) -> (0, 1=w3991:i16)
                n1610 = Build Array(w3991) -> (w3990:i16[])
                n1611 = call-poly <vilib>:"Basic Level Trigger Detection.vi"("signal in"=w3990, "level"=0.5) -> ("trigger detected?"=w3988:bool)  [unwired: 11 in, 2 out]
                n1612 = call "Elapsed Time10"("Time Target (s)"=9.0, "Reset"=w3988, "error in (no error)"=w3981) -> ("Elapsed Time (s)"=w3987:dbl, "error out"=w3982:errorcluster)  [unwired: 9 in, 6 out]
                "Elapsed Time (s) 6" <- w3987
                n1613 = Add(x=w3985, y=w3984) -> (x+y=w3983:dbl)
                n1614 = In Range and Coerce(upper limit=w3983, x=w3987, lower limit=w3984) -> (In Range?=w3986:bool)  [unwired: 1 out]
              }
            }
            n1615 = local read "decrease D05"() -> (w3970:bool)
            n1616 = local read "increase D05"() -> (w3969:bool)
            n1617 = local read "no change D05"() -> (w3968:bool)
            n1618 = local read "sudden change D05"() -> (w3967:bool)
            n1619 = local read "last error 05"() -> (w3966:dbl)
            n1620 = local read "previouse speed D05"() -> (w3965:dbl)
            n1621 = local read "pulse width D05"() -> (w3964:dbl)
            n1622 = local read "slope D05"() -> (w3963:dbl)
            n1623 = Less Than 0?(x=w3975) -> (x < 0?=w3974:bool)
            n1624 = Bundle("decrease D05"=w3970, "increase D05"=w3969, "no change D05"=w3968, "sudden change D05"=w3967, "last error 05"=w3966, "previouse speed D05"=w3965, "pulse width D05"=w3964, "slope D05"=w3963) -> (w3962:T36)  [unwired: 1 in]
            n1625 = shared-variable ".\\control setting.lvlib\\ControlInfoD05"(w3962) -> ()  [unwired: 1 in, 1 out]
            "output value 5" <- w3975
          }
          frame #4 {
            # "incrise"
            # "block increase or decrease if speed limit is minimum or maximum"
            n1626 = property on="speed  min 05" class="Bool (strict)"() -> ("Value"=w3995:bool)  [unwired: 2 in, 2 out]
            n1627 = Select(t=FALSE, s=w4006, f=w4005) -> (s? t:f=w4000:bool)
            n1628 = Select(t=w4005, s=w4006, f=FALSE ("t")) -> (s? t:f=w3998:bool)
            n1629 = property on="speed max 05" class="Bool (strict)"() -> ("Value"=w3996:bool)  [unwired: 2 in, 2 out]
            n1630 = Select(t=FALSE, s=w3996, f=w4000) -> (s? t:f=w3999:bool)
            n1631 = Select(t=FALSE, s=w3995, f=w3998) -> (s? t:f=w3997:bool)
          }
        }
      }
    }
    n1632 = case shown="True" w3795 {
      tunnel: w3786 -> [_ w4392]
      tunnel: w3790 -> [w4373 w4391]
      tunnel: [w4373 w4374] -> w3779
      tunnel: [w4373 w4374] -> w3778
      tunnel: [FALSE ("t") w4390] -> w3777
      tunnel: [FALSE ("t") w4389] -> w3772
      tunnel: w3794 -> [w4370 w4381]
      tunnel: [w4370 w4379] -> w3760
      tunnel: w3785 -> [_ w4375]
      frame False {
      }
      frame True {
        n1633 = flat-sequence {
          tunnel: w4392 -> [w4426]
          tunnel: w4391 -> [w4427]
          tunnel: w4375 -> [w4428]
          tunnel: [w4428] -> w4386
          tunnel: [w4427] -> w4385
          tunnel: [w4426] -> w4384
          tunnel: [w4406] -> w4383
          tunnel: [w4405] -> w4382
          tunnel: w4381 -> [w4405]
          tunnel: [w4446] -> w4403
          tunnel: [w4453] -> w4402
          tunnel: [w4443] -> w4401
          tunnel: [w4431] -> w4400
          tunnel: [w4442] -> w4399
          tunnel: w4386 -> [w4442]
          tunnel: w4385 -> [w4445]
          tunnel: w4384 -> [w4453]
          tunnel: w4383 -> [w4437]
          tunnel: w4382 -> [w4435]
          tunnel: [w4435] -> w4380
          tunnel: [w4429] -> w4376
          tunnel: w4403 -> [w4463]
          tunnel: w4402 -> [w4459]
          tunnel: w4401 -> [w4460]
          tunnel: [w4462] -> w4398
          tunnel: w4400 -> [w4462]
          tunnel: [w4461] -> w4397
          tunnel: w4399 -> [w4458]
          tunnel: [w4458] -> w4396
          tunnel: [w4457] -> w4387
          tunnel: w4380 -> [w4456]
          tunnel: [w4455] -> w4377
          tunnel: w4376 -> [w4454]
          tunnel: w4398 -> [w4523]
          tunnel: w4397 -> [w4520]
          tunnel: [w4521] -> w4395
          tunnel: [w4519] -> w4394
          tunnel: [w4518] -> w4393
          tunnel: w4396 -> [w4518]
          tunnel: [w4517] -> w4388
          tunnel: w4387 -> [w4516]
          tunnel: [w4515] -> w4378
          tunnel: w4377 -> [w4515]
          tunnel: w4395 -> [w4550]
          tunnel: w4394 -> [w4551]
          tunnel: w4393 -> [_]
          tunnel: [w4545] -> w4390
          tunnel: [w4542] -> w4389
          tunnel: [w4548] -> w4374
          tunnel: w4388 -> [w4548]
          tunnel: [w4539] -> w4379
          tunnel: w4378 -> [w4539]
          frame #0 {
            n1634 = shared-variable ".\\control setting.lvlib\\SetPoints"() -> (w4414:dbl[])  [unwired: 1 in, 1 out]
            n1635 = property on="2D array out" class="Arr (strict)"() -> ("Value"=w4407:dbl[][])  [unwired: 2 in, 2 out]
            n1636 = Index Array(array=w4407, index (row)=0, index (col)=1 ("disabled index (col)")) -> (element=w4412:dbl)
            n1637 = Index Array(array=w4414, index=1) -> (element=w4415:dbl)
            n1638 = Subtract(x=w4412, y=w4415) -> (x-y=w4416:dbl)
            n1639 = property on="speed  min 02" class="Bool (strict)"() -> ("Value"=w4422:bool)  [unwired: 2 in, 2 out]
            n1640 = property on="speed max 02" class="Bool (strict)"() -> ("Value"=w4419:bool)  [unwired: 2 in, 2 out]
            n1641 = Absolute Value(x=w4416) -> (abs(x)=w4410:dbl)
            n1642 = Less Than 0?(x=w4416) -> (x < 0?=w4418:bool)
            n1643 = Greater Than 0?(x=w4416) -> (x > 0?=w4423:bool)
            n1644 = property on="no change D02" class="Bool (strict)"() -> ("Value"=w4404:bool)  [unwired: 2 in, 2 out]
            n1645 = Not And(1:w4419, 2:w4418) -> (0:w4421:bool)
            n1646 = Not And(1:w4422, 2:w4423) -> (0:w4425:bool)
            n1647 = Greater?(x=w4410, y=1.0) -> (0:w4417:bool)
            n1648 = And(x=w4404, y=w4417) -> (x .and. y?=w4420:bool)
            n1649 = And(x=w4420, y=w4421) -> (x .and. y?=w4424:bool)
            n1650 = And(x=w4424, y=w4425) -> (x .and. y?=w4406:bool)
            "sudden change D02" <- w4406
          }
          frame #1 {
            w4430 = u16 0 items=["Falling Edge", "Rising Edge"] ("trigger slope")
            # "D27 Tick count to reach the pulse time (defult : 5min)"
            n1651 = Boolean To (0,1)(Boolean=w4437) -> (0, 1=w4440:i16)
            n1652 = Build Array(w4440) -> (w4439:i16[])
            n1653 = shared-variable ".\\control setting.lvlib\\PlsePeriod"() -> (w4441:i16)  [unwired: 1 in, 1 out]
            n1654 = call-poly <vilib>:"Basic Level Trigger Detection.vi"("signal in"=w4439, "level"=0.5) -> ("trigger detected?"=w4436:bool)  [unwired: 11 in, 2 out]
            n1655 = call "Elapsed Time3"("Time Target (s)"=w4441, "Reset"=w4436, "error in (no error)"=w4445) -> ("Elapsed Time (s)"=w4449:dbl, "error out"=w4444:errorcluster)  [unwired: 9 in, 6 out]
            n1656 = In Range and Coerce(upper limit=10.0, x=w4449, lower limit=0.1) -> (In Range?=w4431:bool)  [unwired: 1 out]
            n1657 = Boolean To (0,1)(Boolean=w4431) -> (0, 1=w4452:i16)
            n1658 = Boolean To (0,1)(Boolean=w4431) -> (0, 1=w4432:i16)
            n1659 = Build Array(w4452) -> (w4451:i16[])
            n1660 = Build Array(w4432) -> (w4433:i16[])
            n1661 = call-poly <vilib>:"Basic Level Trigger Detection.vi"("signal in"=w4451, "level"=0.5, "error in (no error)"=w4444) -> ("trigger detected?"=w4446:bool, "error out"=w4443:errorcluster)  [unwired: 10 in, 1 out]
            n1662 = call-poly <vilib>:"Basic Level Trigger Detection.vi"("signal in"=w4433, "level"=0.5, "trigger slope"=w4430) -> ("trigger detected?"=w4429:bool)  [unwired: 10 in, 2 out]
          }
          frame #2 {
            # "calculate the pulse width by fuzzy controler"
            n1663 = case shown="True" w4463 {
              tunnel: w4459 -> [_ w4505]
              tunnel: [w4474 w4475] -> w4461
              tunnel: w4458 -> [_ w4487]
              tunnel: w4460 -> [w4473 w4503]
              tunnel: [w4473 w4501] -> w4457
              frame False {
                n1664 = property on="output value 2" class="DigNum (strict)"() -> ("Value"=w4474:dbl)  [unwired: 2 in, 2 out]
              }
              frame True {
                n1665 = property on="2D array out" class="Arr (strict)"(error in=w4503) -> (error out=w4502:errorcluster, "Value"=w4488:dbl[][])  [unwired: 1 in, 1 out]
                n1666 = shared-variable ".\\control setting.lvlib\\SetPoints"() -> (w4494:dbl[])  [unwired: 1 in, 1 out]
                n1667 = Index Array(array=w4488, index (row)=0 ("disabled index (row)"), index (col)=1 ("disabled index (col)")) -> (element=w4499:dbl)
                n1668 = Index Array(array=w4488, index (col)=1 ("disabled index (col)")) -> (element=w4490:dbl[])  [unwired: 1 in]
                n1669 = Reverse 1D Array(array=w4490) -> (reversed array=w4489:dbl[])
                n1670 = Index Array(array=w4494, index=1) -> (element=w4493:dbl)
                n1671 = Subtract(x=w4499, y=w4493) -> (x-y=w4482:dbl)
                "last error 02" <- w4482
                n1672 = call <vilib>:"Linear Fit.vi"("Y"=w4489, "X"=w4487) -> ("slope"=w4485:dbl)  [unwired: 9 in, 4 out]
                n1673 = Multiply(x=w4485, y=24.0) -> (x*y=w4483:dbl)
                "slope D02" <- w4483
                n1674 = Build Array(w4482, w4483) -> (w4486:dbl[])
                n1675 = call-poly <vilib>:"FL Fuzzy Controller.vi"("error in (no error)"=w4502, "input values"=w4486, "fuzzy system in"=w4505) -> ("error out"=w4501:errorcluster, "output value"=w4498:dbl)  [unwired: 4 in, 3 out]
                n1676 = property on="speed  min 02" class="Bool (strict)"() -> ("Value"=w4479:bool)  [unwired: 2 in, 2 out]
                n1677 = Divide(x=w4498, y=0.25) -> (x/y=w4492:dbl)
                n1678 = Round To Nearest(number=w4492) -> (nearest integer value=w4475:dbl)
                n1679 = property on="speed max 02" class="Bool (strict)"() -> ("Value"=w4480:bool)  [unwired: 2 in, 2 out]
                n1680 = Multiply(x=w4475, y=1.2) -> (x*y=→"pulse width D02":dbl)
                n1681 = call "change situation.vi"("pulse width"=w4475, "speed max"=w4480, "speed min"=w4479) -> ("no change"=→"no change D02":bool, "increas"=→"increase D02":bool, "decreas"=→"decrease D02":bool)  [unwired: 14 in]
              }
            }
            n1682 = case shown="True" w4454 {
              tunnel: w4456 -> [w4464 w4472]
              tunnel: [w4464 w4468] -> w4455
              frame False {
              }
              frame True {
                n1683 = Delete From Array(array=w4472, index=1) -> (array with subset deleted=w4470:dbl[])  [unwired: 1 in, 1 out]
                n1684 = property on="SPEED 02" class="DigNum (strict)"() -> ("Value"=w4465:dbl)  [unwired: 2 in, 2 out]
                n1685 = Insert Into Array(array=w4470, index=0, new element=w4465) -> (w4468:dbl[])
                n1686 = Index Array(array=w4468, index #1=0 ("index")) -> (element #2=→"previous speed D02":dbl)  [unwired: 1 in, 1 out]
              }
            }
          }
          frame #3 {
            # "create pulse width by Timer"
            n1687 = Absolute Value(x=w4520) -> (abs(x)=w4522:dbl)
            n1688 = local read "decrease D02"() -> (w4507:bool)
            n1689 = local read "increase D02"() -> (w4508:bool)
            n1690 = local read "no change D02"() -> (w4509:bool)
            n1691 = local read "sudden change D02"() -> (w4510:bool)
            n1692 = local read "last error 02"() -> (w4511:dbl)
            n1693 = local read "previous speed D02"() -> (w4512:dbl)
            n1694 = local read "pulse width D02"() -> (w4513:dbl)
            n1695 = local read "slope D02"() -> (w4514:dbl)
            n1696 = case shown="True" w4523 {
              selector: w4523 -> [_ w4537]
              tunnel: [FALSE w4531] -> w4521
              tunnel: w4522 -> [_ w4530]
              tunnel: [w4524 w4527] -> w4517
              tunnel: w4516 -> [w4524 w4526]
              frame False {
              }
              frame True {
                w4529 = 1.0 ("lower limit")
                n1697 = Boolean To (0,1)(Boolean=w4537) -> (0, 1=w4536:i16)
                n1698 = Build Array(w4536) -> (w4535:i16[])
                n1699 = call-poly <vilib>:"Basic Level Trigger Detection.vi"("signal in"=w4535, "level"=0.5) -> ("trigger detected?"=w4533:bool)  [unwired: 11 in, 2 out]
                n1700 = call "Elapsed Time4"("Time Target (s)"=9.0, "Reset"=w4533, "error in (no error)"=w4526) -> ("Elapsed Time (s)"=w4532:dbl, "error out"=w4527:errorcluster)  [unwired: 9 in, 6 out]
                "Elapsed Time (s) 3" <- w4532
                n1701 = Add(x=w4530, y=w4529) -> (x+y=w4528:dbl)
                n1702 = In Range and Coerce(upper limit=w4528, x=w4532, lower limit=w4529) -> (In Range?=w4531:bool)  [unwired: 1 out]
              }
            }
            n1703 = Less Than 0?(x=w4520) -> (x < 0?=w4519:bool)
            n1704 = Bundle("decrease D02"=w4507, "increase D02"=w4508, "no change D02"=w4509, "sudden change D02"=w4510, "last error 02"=w4511, "previous speed D02"=w4512, "pulse width D02"=w4513, "slope D02"=w4514) -> (w4506:T37)  [unwired: 1 in]
            n1705 = shared-variable ".\\control setting.lvlib\\ControlInfoD02"(w4506) -> ()  [unwired: 1 in, 1 out]
            "output value 2" <- w4520
          }
          frame #4 {
            # "decrise"
            # "incrise"
            n1706 = property on="speed  min 02" class="Bool (strict)"() -> ("Value"=w4540:bool)  [unwired: 2 in, 2 out]
            n1707 = Select(t=FALSE, s=w4551, f=w4550) -> (s? t:f=w4546:bool)
            n1708 = Select(t=w4550, s=w4551, f=FALSE ("t")) -> (s? t:f=w4543:bool)
            n1709 = property on="speed max 02" class="Bool (strict)"() -> ("Value"=w4541:bool)  [unwired: 2 in, 2 out]
            n1710 = Select(t=FALSE, s=w4541, f=w4546) -> (s? t:f=w4545:bool)
            n1711 = Select(t=FALSE, s=w4540, f=w4543) -> (s? t:f=w4542:bool)
          }
        }
      }
    }
    n1712 = case shown="True" w3791 {
      tunnel: w3786 -> [_ w4030]
      tunnel: w3790 -> [w4011 w4029]
      tunnel: [w4011 w4025] -> w3774
      tunnel: [w4011 w4025] -> w3773
      tunnel: [FALSE ("t") w4028] -> w3769
      tunnel: [FALSE ("t") w4027] -> w3768
      tunnel: w3789 -> [w4008 w4018]
      tunnel: [w4008 w4014] -> w3762
      tunnel: w3785 -> [_ w4012]
      frame False {
      }
      frame True {
        n1713 = flat-sequence {
          tunnel: w4030 -> [w4062]
          tunnel: w4029 -> [w4063]
          tunnel: w4012 -> [w4064]
          tunnel: [w4064] -> w4023
          tunnel: [w4063] -> w4022
          tunnel: [w4062] -> w4021
          tunnel: [w4042] -> w4020
          tunnel: [w4041] -> w4019
          tunnel: w4018 -> [w4041]
          tunnel: [w4082] -> w4039
          tunnel: [w4089] -> w4038
          tunnel: [w4079] -> w4037
          tunnel: [w4067] -> w4036
          tunnel: [w4078] -> w4035
          tunnel: w4023 -> [w4078]
          tunnel: w4022 -> [w4081]
          tunnel: w4021 -> [w4089]
          tunnel: w4020 -> [w4073]
          tunnel: w4019 -> [w4071]
          tunnel: [w4071] -> w4017
          tunnel: [w4066] -> w4013
          tunnel: w4039 -> [w4099]
          tunnel: w4038 -> [w4095]
          tunnel: w4037 -> [w4096]
          tunnel: [w4098] -> w4034
          tunnel: w4036 -> [w4098]
          tunnel: [w4097] -> w4033
          tunnel: w4035 -> [w4090]
          tunnel: [w4094] -> w4024
          tunnel: w4017 -> [w4093]
          tunnel: [w4092] -> w4015
          tunnel: w4013 -> [w4091]
          tunnel: w4034 -> [w4158]
          tunnel: w4033 -> [w4155]
          tunnel: [w4156] -> w4032
          tunnel: [w4154] -> w4031
          tunnel: [w4153] -> w4026
          tunnel: w4024 -> [w4152]
          tunnel: [w4151] -> w4016
          tunnel: w4015 -> [w4151]
          tunnel: w4032 -> [w4185]
          tunnel: w4031 -> [w4186]
          tunnel: [w4179] -> w4028
          tunnel: [w4177] -> w4027
          tunnel: [w4183] -> w4025
          tunnel: w4026 -> [w4183]
          tunnel: [w4174] -> w4014
          tunnel: w4016 -> [w4174]
          frame #0 {
            n1714 = shared-variable ".\\control setting.lvlib\\SetPoints"() -> (w4050:dbl[])  [unwired: 1 in, 1 out]
            n1715 = property on="2D array out" class="Arr (strict)"() -> ("Value"=w4043:dbl[][])  [unwired: 2 in, 2 out]
            n1716 = Index Array(array=w4050, index=3) -> (element=w4051:dbl)
            n1717 = Index Array(array=w4043, index (row)=0, index (col)=3 ("disabled index (col)")) -> (element=w4048:dbl)
            n1718 = Subtract(x=w4048, y=w4051) -> (x-y=w4052:dbl)
            n1719 = property on="speed  min 04" class="Bool (strict)"() -> ("Value"=w4058:bool)  [unwired: 2 in, 2 out]
            n1720 = property on="speed max 04" class="Bool (strict)"() -> ("Value"=w4055:bool)  [unwired: 2 in, 2 out]
            n1721 = property on="no change D04" class="Bool (strict)"() -> ("Value"=w4040:bool)  [unwired: 2 in, 2 out]
            n1722 = Absolute Value(x=w4052) -> (abs(x)=w4046:dbl)
            n1723 = Less Than 0?(x=w4052) -> (x < 0?=w4054:bool)
            n1724 = Greater Than 0?(x=w4052) -> (x > 0?=w4059:bool)
            n1725 = Not And(1:w4055, 2:w4054) -> (0:w4057:bool)
            n1726 = Not And(1:w4058, 2:w4059) -> (0:w4061:bool)
            n1727 = Greater?(x=w4046, y=1.0) -> (0:w4053:bool)
            n1728 = And(x=w4040, y=w4053) -> (x .and. y?=w4056:bool)
            n1729 = And(x=w4056, y=w4057) -> (x .and. y?=w4060:bool)
            n1730 = And(x=w4060, y=w4061) -> (x .and. y?=w4042:bool)
            "sudden change D04" <- w4042
          }
          frame #1 {
            w4065 = u16 0 items=["Falling Edge", "Rising Edge"] ("trigger slope")
            # "D29 Tick count to reach the pulse time (defult : 5min)"
            n1731 = Boolean To (0,1)(Boolean=w4073) -> (0, 1=w4076:i16)
            n1732 = Build Array(w4076) -> (w4075:i16[])
            n1733 = shared-variable ".\\control setting.lvlib\\PlsePeriod"() -> (w4077:i16)  [unwired: 1 in, 1 out]
            n1734 = call-poly <vilib>:"Basic Level Trigger Detection.vi"("signal in"=w4075, "level"=0.5) -> ("trigger detected?"=w4072:bool)  [unwired: 11 in, 2 out]
            n1735 = call "Elapsed Time7"("Time Target (s)"=w4077, "Reset"=w4072, "error in (no error)"=w4081) -> ("Elapsed Time (s)"=w4085:dbl, "error out"=w4080:errorcluster)  [unwired: 9 in, 6 out]
            n1736 = In Range and Coerce(upper limit=10.0, x=w4085, lower limit=0.1) -> (In Range?=w4067:bool)  [unwired: 1 out]
            n1737 = Boolean To (0,1)(Boolean=w4067) -> (0, 1=w4088:i16)
            n1738 = Boolean To (0,1)(Boolean=w4067) -> (0, 1=w4068:i16)
            n1739 = Build Array(w4088) -> (w4087:i16[])
            n1740 = Build Array(w4068) -> (w4069:i16[])
            n1741 = call-poly <vilib>:"Basic Level Trigger Detection.vi"("signal in"=w4087, "level"=0.5, "error in (no error)"=w4080) -> ("trigger detected?"=w4082:bool, "error out"=w4079:errorcluster)  [unwired: 10 in, 1 out]
            n1742 = call-poly <vilib>:"Basic Level Trigger Detection.vi"("signal in"=w4069, "level"=0.5, "trigger slope"=w4065) -> ("trigger detected?"=w4066:bool)  [unwired: 10 in, 2 out]
          }
          frame #2 {
            # "calculate the pulse width by fuzzy controler"
            n1743 = case shown="True" w4099 {
              tunnel: w4095 -> [_ w4141]
              tunnel: [w4110 w4131] -> w4097
              tunnel: w4096 -> [w4109 w4139]
              tunnel: [w4109 w4137] -> w4094
              tunnel: w4090 -> [_ w4121]
              frame False {
                n1744 = property on="output value 4" class="DigNum (strict)"() -> ("Value"=w4110:dbl)  [unwired: 2 in, 2 out]
              }
              frame True {
                n1745 = property on="2D array out" class="Arr (strict)"(error in=w4139) -> (error out=w4138:errorcluster, "Value"=w4123:dbl[][])  [unwired: 1 in, 1 out]
                n1746 = shared-variable ".\\control setting.lvlib\\SetPoints"() -> (w4129:dbl[])  [unwired: 1 in, 1 out]
                n1747 = Index Array(array=w4123, index (row)=0 ("disabled index (row)"), index (col)=3 ("disabled index (col)")) -> (element=w4135:dbl)
                n1748 = Index Array(array=w4123, index (col)=3 ("disabled index (col)")) -> (element=w4126:dbl[])  [unwired: 1 in]
                n1749 = Reverse 1D Array(array=w4126) -> (reversed array=w4125:dbl[])
                n1750 = Index Array(array=w4129, index=3) -> (element=w4128:dbl)
                n1751 = Subtract(x=w4135, y=w4128) -> (x-y=w4117:dbl)
                "last error 04" <- w4117
                n1752 = call <vilib>:"Linear Fit.vi"("Y"=w4125, "X"=w4121) -> ("slope"=w4120:dbl)  [unwired: 9 in, 4 out]
                n1753 = Multiply(x=w4120, y=24.0) -> (x*y=w4118:dbl)
                "slope D04" <- w4118
                n1754 = Build Array(w4117, w4118) -> (w4122:dbl[])
                n1755 = call-poly <vilib>:"FL Fuzzy Controller.vi"("error in (no error)"=w4138, "input values"=w4122, "fuzzy system in"=w4141) -> ("error out"=w4137:errorcluster, "output value"=w4133:dbl)  [unwired: 4 in, 3 out]
                n1756 = property on="speed  min 04" class="Bool (strict)"() -> ("Value"=w4114:bool)  [unwired: 2 in, 2 out]
                n1757 = property on="speed max 04" class="Bool (strict)"() -> ("Value"=w4115:bool)  [unwired: 2 in, 2 out]
                n1758 = Divide(x=w4133, y=0.25) -> (x/y=w4127:dbl)
                n1759 = Round To Nearest(number=w4127) -> (nearest integer value=w4116:dbl)
                n1760 = call "change situation.vi"("pulse width"=w4116, "speed max"=w4115, "speed min"=w4114) -> ("no change"=→"no change D04":bool, "increas"=→"increase D04":bool, "decreas"=→"decrease D04":bool)  [unwired: 14 in]
                n1761 = Multiply(x=w4116, y=1.2) -> (x*y=w4131:dbl)
                "pulse width D04" <- w4131
              }
            }
            n1762 = case shown="True" w4091 {
              tunnel: w4093 -> [w4100 w4108]
              tunnel: [w4100 w4104] -> w4092
              frame False {
              }
              frame True {
                n1763 = Delete From Array(array=w4108, index=1) -> (array with subset deleted=w4106:dbl[])  [unwired: 1 in, 1 out]
                n1764 = property on="SPEED 04" class="DigNum (strict)"() -> ("Value"=w4101:dbl)  [unwired: 2 in, 2 out]
                n1765 = Insert Into Array(array=w4106, index=0, new element=w4101) -> (w4104:dbl[])
                n1766 = Index Array(array=w4104, index #1=0 ("index")) -> (element #2=→"previouse speed D04":dbl)  [unwired: 1 in, 1 out]
              }
            }
          }
          frame #3 {
            # "create pulse width by Timer"
            n1767 = Absolute Value(x=w4155) -> (abs(x)=w4157:dbl)
            n1768 = case shown="True" w4158 {
              selector: w4158 -> [_ w4172]
              tunnel: [FALSE w4166] -> w4156
              tunnel: w4157 -> [_ w4165]
              tunnel: [w4159 w4162] -> w4153
              tunnel: w4152 -> [w4159 w4161]
              frame False {
              }
              frame True {
                w4164 = 1.0 ("lower limit")
                n1769 = Boolean To (0,1)(Boolean=w4172) -> (0, 1=w4171:i16)
                n1770 = Build Array(w4171) -> (w4170:i16[])
                n1771 = call-poly <vilib>:"Basic Level Trigger Detection.vi"("signal in"=w4170, "level"=0.5) -> ("trigger detected?"=w4168:bool)  [unwired: 11 in, 2 out]
                n1772 = call "Elapsed Time8"("Time Target (s)"=9.0, "Reset"=w4168, "error in (no error)"=w4161) -> ("Elapsed Time (s)"=w4167:dbl, "error out"=w4162:errorcluster)  [unwired: 9 in, 6 out]
                "Elapsed Time (s) 5" <- w4167
                n1773 = Add(x=w4165, y=w4164) -> (x+y=w4163:dbl)
                n1774 = In Range and Coerce(upper limit=w4163, x=w4167, lower limit=w4164) -> (In Range?=w4166:bool)  [unwired: 1 out]
              }
            }
            n1775 = Less Than 0?(x=w4155) -> (x < 0?=w4154:bool)
            n1776 = local read "decrease D04"() -> (w4143:bool)
            n1777 = local read "increase D04"() -> (w4144:bool)
            n1778 = local read "no change D04"() -> (w4145:bool)
            n1779 = local read "sudden change D04"() -> (w4146:bool)
            n1780 = local read "last error 04"() -> (w4147:dbl)
            n1781 = local read "previouse speed D04"() -> (w4148:dbl)
            n1782 = local read "pulse width D04"() -> (w4149:dbl)
            n1783 = local read "slope D04"() -> (w4150:dbl)
            n1784 = Bundle("decrease D04"=w4143, "increase D04"=w4144, "no change D04"=w4145, "sudden change D04"=w4146, "last error 04"=w4147, "previouse speed D04"=w4148, "pulse width D04"=w4149, "slope D04"=w4150) -> (w4142:T38)  [unwired: 1 in]
            n1785 = shared-variable ".\\control setting.lvlib\\ControlInfoD04"(w4142) -> ()  [unwired: 1 in, 1 out]
            "output value 4" <- w4155
          }
          frame #4 {
            # "incrise"
            n1786 = property on="speed  min 04" class="Bool (strict)"() -> ("Value"=w4175:bool)  [unwired: 2 in, 2 out]
            n1787 = Select(t=FALSE, s=w4186, f=w4185) -> (s? t:f=w4180:bool)
            n1788 = Select(t=w4185, s=w4186, f=FALSE ("t")) -> (s? t:f=w4178:bool)
            n1789 = property on="speed max 04" class="Bool (strict)"() -> ("Value"=w4176:bool)  [unwired: 2 in, 2 out]
            n1790 = Select(t=FALSE, s=w4175, f=w4178) -> (s? t:f=w4177:bool)
            n1791 = Select(t=FALSE, s=w4176, f=w4180) -> (s? t:f=w4179:bool)
          }
        }
      }
    }
    n1792 = case shown="True" w3793 {
      tunnel: w3786 -> [_ w4211]
      tunnel: w3790 -> [w4191 w4210]
      tunnel: [w4191 w4206] -> w3776
      tunnel: [w4191 w4206] -> w3775
      tunnel: [FALSE ("t") w4209] -> w3771
      tunnel: [FALSE ("t") w4208] -> w3770
      tunnel: w3792 -> [w4188 w4199]
      tunnel: [w4188 w4197] -> w3761
      tunnel: w3785 -> [_ w4193]
      frame False {
      }
      frame True {
        n1793 = flat-sequence {
          tunnel: w4211 -> [w4243]
          tunnel: w4210 -> [w4244]
          tunnel: w4193 -> [w4245]
          tunnel: [w4245] -> w4204
          tunnel: [w4244] -> w4203
          tunnel: [w4243] -> w4202
          tunnel: [w4223] -> w4201
          tunnel: [w4222] -> w4200
          tunnel: w4199 -> [w4222]
          tunnel: [w4264] -> w4220
          tunnel: [w4271] -> w4219
          tunnel: [w4261] -> w4218
          tunnel: [w4250] -> w4217
          tunnel: [w4260] -> w4216
          tunnel: w4204 -> [w4260]
          tunnel: w4203 -> [w4263]
          tunnel: w4202 -> [w4271]
          tunnel: w4201 -> [w4246]
          tunnel: w4200 -> [w4254]
          tunnel: [w4254] -> w4198
          tunnel: [w4248] -> w4194
          tunnel: [w4247] -> w4192
          tunnel: w4220 -> [w4282]
          tunnel: w4219 -> [w4278]
          tunnel: w4218 -> [w4279]
          tunnel: [w4281] -> w4215
          tunnel: w4217 -> [w4281]
          tunnel: [w4280] -> w4214
          tunnel: w4216 -> [w4277]
          tunnel: [w4276] -> w4205
          tunnel: w4198 -> [w4275]
          tunnel: [w4274] -> w4195
          tunnel: w4194 -> [w4273]
          tunnel: w4192 -> [w4272]
          tunnel: w4215 -> [w4340]
          tunnel: w4214 -> [w4337]
          tunnel: [w4338] -> w4213
          tunnel: [w4336] -> w4212
          tunnel: [w4335] -> w4207
          tunnel: w4205 -> [w4334]
          tunnel: [w4333] -> w4196
          tunnel: w4195 -> [w4333]
          tunnel: w4213 -> [w4367]
          tunnel: w4212 -> [w4368]
          tunnel: [w4361] -> w4209
          tunnel: [w4359] -> w4208
          tunnel: [w4365] -> w4206
          tunnel: w4207 -> [w4365]
          tunnel: [w4356] -> w4197
          tunnel: w4196 -> [w4356]
          frame #0 {
            n1794 = shared-variable ".\\control setting.lvlib\\SetPoints"() -> (w4235:dbl[])  [unwired: 1 in, 1 out]
            n1795 = property on="2D array out" class="Arr (strict)"() -> ("Value"=w4242:dbl[][])  [unwired: 2 in, 2 out]
            n1796 = Index Array(array=w4242, index (row)=0, index (col)=2 ("disabled index (col)")) -> (element=w4237:dbl)
            n1797 = Index Array(array=w4235, index=2) -> (element=w4234:dbl)
            n1798 = Subtract(x=w4237, y=w4234) -> (x-y=w4233:dbl)
            n1799 = property on="speed  min 03" class="Bool (strict)"() -> ("Value"=w4227:bool)  [unwired: 2 in, 2 out]
            n1800 = property on="speed max 03" class="Bool (strict)"() -> ("Value"=w4230:bool)  [unwired: 2 in, 2 out]
            n1801 = Absolute Value(x=w4233) -> (abs(x)=w4239:dbl)
            n1802 = Less Than 0?(x=w4233) -> (x < 0?=w4231:bool)
            n1803 = Greater Than 0?(x=w4233) -> (x > 0?=w4226:bool)
            n1804 = property on="no change D03" class="Bool (strict)"() -> ("Value"=w4221:bool)  [unwired: 2 in, 2 out]
            n1805 = Not And(1:w4230, 2:w4231) -> (0:w4228:bool)
            n1806 = Not And(1:w4227, 2:w4226) -> (0:w4224:bool)
            n1807 = Greater?(x=w4239, y=1.0) -> (0:w4232:bool)
            n1808 = And(x=w4221, y=w4232) -> (x .and. y?=w4229:bool)
            n1809 = And(x=w4229, y=w4228) -> (x .and. y?=w4225:bool)
            n1810 = And(x=w4225, y=w4224) -> (x .and. y?=w4223:bool)
            "sudden change D03" <- w4223
          }
          frame #1 {
            w4249 = u16 0 items=["Falling Edge", "Rising Edge"] ("trigger slope")
            # "D28 Tick count to reach the pulse time (defult : 5min)"
            n1811 = Boolean To (0,1)(Boolean=w4246) -> (0, 1=w4256:i16)
            n1812 = Build Array(w4256) -> (w4257:i16[])
            n1813 = shared-variable ".\\control setting.lvlib\\PlsePeriod"() -> (w4259:i16)  [unwired: 1 in, 1 out]
            n1814 = call-poly <vilib>:"Basic Level Trigger Detection.vi"("signal in"=w4257, "level"=0.5) -> ("trigger detected?"=w4255:bool)  [unwired: 11 in, 2 out]
            n1815 = call "Elapsed Time5"("Time Target (s)"=w4259, "Reset"=w4255, "error in (no error)"=w4263) -> ("Elapsed Time (s)"=w4267:dbl, "error out"=w4262:errorcluster)  [unwired: 9 in, 6 out]
            n1816 = In Range and Coerce(upper limit=10.0, x=w4267, lower limit=0.1) -> (In Range?=w4250:bool)  [unwired: 1 out]
            n1817 = Boolean To (0,1)(Boolean=w4250) -> (0, 1=w4270:i16)
            n1818 = Boolean To (0,1)(Boolean=w4250) -> (0, 1=w4251:i16)
            n1819 = Build Array(w4270) -> (w4269:i16[])
            n1820 = Build Array(w4251) -> (w4252:i16[])
            n1821 = property on="2D array out" class="Arr (strict)"() -> ("Value"=w4247:dbl[][])  [unwired: 2 in, 2 out]
            n1822 = call-poly <vilib>:"Basic Level Trigger Detection.vi"("signal in"=w4269, "level"=0.5, "error in (no error)"=w4262) -> ("trigger detected?"=w4264:bool, "error out"=w4261:errorcluster)  [unwired: 10 in, 1 out]
            n1823 = call-poly <vilib>:"Basic Level Trigger Detection.vi"("signal in"=w4252, "level"=0.5, "trigger slope"=w4249) -> ("trigger detected?"=w4248:bool)  [unwired: 10 in, 2 out]
          }
          frame #2 {
            # "calculate the pulse width by fuzzy controler"
            n1824 = case shown="True" w4282 {
              tunnel: w4278 -> [_ w4323]
              tunnel: [w4293 w4315] -> w4280
              tunnel: w4277 -> [_ w4306]
              tunnel: w4279 -> [w4292 w4301]
              tunnel: [w4292 w4321] -> w4276
              tunnel: w4272 -> [_ w4302]
              frame False {
                n1825 = property on="output value 3" class="DigNum (strict)"() -> ("Value"=w4293:dbl)  [unwired: 2 in, 2 out]
              }
              frame True {
                n1826 = shared-variable ".\\control setting.lvlib\\SetPoints"() -> (w4313:dbl[])  [unwired: 1 in, 1 out]
                n1827 = Index Array(array=w4302, index (row)=0 ("disabled index (row)"), index (col)=2 ("disabled index (col)")) -> (element=w4319:dbl)
                n1828 = Index Array(array=w4302, index (col)=2 ("disabled index (col)")) -> (element=w4309:dbl[])  [unwired: 1 in]
                n1829 = Reverse 1D Array(array=w4309) -> (reversed array=w4308:dbl[])
                n1830 = Index Array(array=w4313, index=2) -> (element=w4312:dbl)
                n1831 = Subtract(x=w4319, y=w4312) -> (x-y=w4300:dbl)
                "last error 03" <- w4300
                n1832 = call <vilib>:"Linear Fit.vi"("Y"=w4308, "X"=w4306) -> ("slope"=w4305:dbl)  [unwired: 9 in, 4 out]
                n1833 = Multiply(x=w4305, y=24.0) -> (x*y=w4303:dbl)
                "slope D03" <- w4303
                n1834 = Build Array(w4300, w4303) -> (w4307:dbl[])
                n1835 = call-poly <vilib>:"FL Fuzzy Controller.vi"("error in (no error)"=w4301, "input values"=w4307, "fuzzy system in"=w4323) -> ("error out"=w4321:errorcluster, "output value"=w4318:dbl)  [unwired: 4 in, 3 out]
                n1836 = property on="speed max 03" class="Bool (strict)"() -> ("Value"=w4298:bool)  [unwired: 2 in, 2 out]
                n1837 = property on="speed  min 03" class="Bool (strict)"() -> ("Value"=w4297:bool)  [unwired: 2 in, 2 out]
                n1838 = Divide(x=w4318, y=0.25) -> (x/y=w4311:dbl)
                n1839 = Round To Nearest(number=w4311) -> (nearest integer value=w4299:dbl)
                n1840 = Multiply(x=w4299, y=1.2) -> (x*y=w4315:dbl)
                "pulse width D03" <- w4315
                n1841 = call "change situation.vi"("pulse width"=w4299, "speed max"=w4298, "speed min"=w4297) -> ("no change"=→"no change D03":bool, "increas"=→"increase D03":bool, "decreas"=→"decrease D03":bool)  [unwired: 14 in]
              }
            }
            n1842 = case shown="True" w4273 {
              tunnel: w4275 -> [w4283 w4291]
              tunnel: [w4283 w4287] -> w4274
              frame False {
              }
              frame True {
                n1843 = Delete From Array(array=w4291, index=1) -> (array with subset deleted=w4289:dbl[])  [unwired: 1 in, 1 out]
                n1844 = property on="SPEED 03" class="DigNum (strict)"() -> ("Value"=w4284:dbl)  [unwired: 2 in, 2 out]
                n1845 = Insert Into Array(array=w4289, index=0, new element=w4284) -> (w4287:dbl[])
                n1846 = Index Array(array=w4287, index #1=0 ("index")) -> (element #2=→"previous speed D03":dbl)  [unwired: 1 in, 1 out]
              }
            }
          }
          frame #3 {
            # "create pulse width by Timer"
            n1847 = Absolute Value(x=w4337) -> (abs(x)=w4339:dbl)
            n1848 = case shown="True" w4340 {
              selector: w4340 -> [_ w4354]
              tunnel: [FALSE w4348] -> w4338
              tunnel: w4339 -> [_ w4347]
              tunnel: [w4341 w4344] -> w4335
              tunnel: w4334 -> [w4341 w4343]
              frame False {
              }
              frame True {
                w4346 = 1.0 ("lower limit")
                n1849 = Boolean To (0,1)(Boolean=w4354) -> (0, 1=w4353:i16)
                n1850 = Build Array(w4353) -> (w4352:i16[])
                n1851 = call-poly <vilib>:"Basic Level Trigger Detection.vi"("signal in"=w4352, "level"=0.5) -> ("trigger detected?"=w4350:bool)  [unwired: 11 in, 2 out]
                n1852 = call "Elapsed Time6"("Time Target (s)"=9.0, "Reset"=w4350, "error in (no error)"=w4343) -> ("Elapsed Time (s)"=w4349:dbl, "error out"=w4344:errorcluster)  [unwired: 9 in, 6 out]
                "Elapsed Time (s) 4" <- w4349
                n1853 = Add(x=w4347, y=w4346) -> (x+y=w4345:dbl)
                n1854 = In Range and Coerce(upper limit=w4345, x=w4349, lower limit=w4346) -> (In Range?=w4348:bool)  [unwired: 1 out]
              }
            }
            n1855 = Less Than 0?(x=w4337) -> (x < 0?=w4336:bool)
            n1856 = local read "decrease D03"() -> (w4332:bool)
            n1857 = local read "increase D03"() -> (w4331:bool)
            n1858 = local read "no change D03"() -> (w4330:bool)
            n1859 = local read "sudden change D03"() -> (w4329:bool)
            n1860 = local read "last error 03"() -> (w4328:dbl)
            n1861 = local read "previous speed D03"() -> (w4327:dbl)
            n1862 = local read "pulse width D03"() -> (w4326:dbl)
            n1863 = local read "slope D03"() -> (w4325:dbl)
            n1864 = Bundle("decrease D03"=w4332, "increase D03"=w4331, "no change D03"=w4330, "sudden change D03"=w4329, "last error 03"=w4328, "previous speed D03"=w4327, "pulse width D03"=w4326, "slope D03"=w4325) -> (w4324:T39)  [unwired: 1 in]
            n1865 = shared-variable ".\\control setting.lvlib\\ControlInfoD03"(w4324) -> ()  [unwired: 1 in, 1 out]
            "output value 3" <- w4337
          }
          frame #4 {
            # "decrise"
            # "incrise"
            n1866 = property on="speed  min 03" class="Bool (strict)"() -> ("Value"=w4357:bool)  [unwired: 2 in, 2 out]
            n1867 = Select(t=FALSE, s=w4368, f=w4367) -> (s? t:f=w4362:bool)
            n1868 = Select(t=w4367, s=w4368, f=FALSE ("t")) -> (s? t:f=w4360:bool)
            n1869 = property on="speed max 03" class="Bool (strict)"() -> ("Value"=w4358:bool)  [unwired: 2 in, 2 out]
            n1870 = Select(t=FALSE, s=w4358, f=w4362) -> (s? t:f=w4361:bool)
            n1871 = Select(t=FALSE, s=w4357, f=w4360) -> (s? t:f=w4359:bool)
          }
        }
      }
    }
    n1872 = Wait (ms)(milliseconds to wait=u32 10) -> ()  [unwired: 1 out]
    n1873 = Merge Errors(w3765, w3764) -> (→"error out 8":errorcluster)
    n1874 = Build Array(w3783, w3782, w3777, w3772, w3771, w3770, w3769, w3768) -> (w3808:bool[])
    n1875 = Build Array(w3767, w3766) -> (w3807:bool[])
    n1876 = Boolean Array To Number(Boolean array=w3808) -> (number=w3816:u32)
    n1877 = Boolean Array To Number(Boolean array=w3807) -> (number=w3814:u32)
    n1878 = shared-variable ".\\trends.lvlib\\d05Pulse"(w3807) -> ()  [unwired: 1 in, 1 out]
    n1879 = shared-variable ".\\trends.lvlib\\pulseTrendBoolean"(w3808) -> ()  [unwired: 1 in, 1 out]
    n1880 = To Unsigned Byte Integer(number=w3816) -> (unsigned 8bit integer=w3815:u8)
    n1881 = To Unsigned Byte Integer(number=w3814) -> (unsigned 8bit integer=w3813:u8)
    n1882 = Merge Errors(w3779, w3778) -> (→"error out 5":errorcluster)
    n1883 = Build Array(w3815, w3813) -> (w3809:u8[])
    n1884 = Merge Errors(w3774, w3773) -> (→"error out 7":errorcluster)
    n1885 = Merge Errors(w3781, w3780) -> (→"error out 3":errorcluster)
    n1886 = disable-structure shown="Disabled" {
      disable-tunnel: [w3827 _] -> w3812
      disable-tunnel: w3811 -> [w3826 _]
      disable-tunnel: w3810 -> [w3825 _]
      disable-tunnel: w3809 -> [w3824 _]
      frame Disabled {
        n1887 = call-poly <userlib>:"DAQNavi Write.vi"("error in (no error)"=w3825, "data"=w3824, "task in"=w3826) -> ("error out"=w3827:errorcluster)  [unwired: 6 in, 2 out]
      }
      frame Enabled {
      }
    }
    "error out 13" <- w3812
    n1888 = shared-variable ".\\trends.lvlib\\pulseTrends"(w3809) -> ()  [unwired: 1 in, 1 out]
    n1889 = Merge Errors(w3776, w3775) -> (→"error out 6":errorcluster)
  }
  "live grading array size" <- w85
  "avg grading array size" <- w80
